vi "TLB Native Dynamic Events ver 0.24.vi"() -> ()   [LabVIEW 2018]
uses:
  Labview Training Phase 2/Enum Controls/States for Action Engine.ctl
  TLB Type Definitions/State Type Definitions, for 0.26g versions and later 2.ctl
  TLB Type Definitions/Intruction Type Definitions.ctl
  TLB Type Definitions/Encoder cluster.ctl
  TLB Type Definitions/PING CLUSTER.ctl
  <vilib>/Studica/Studica Toolkit/NavX/NavX.lvlib
  <vilib>/Studica/Studica Toolkit/Background/DIO Channel.ctl
  Underlying VI's/NavX VI/navX type def.ctl
  <vilib>/Studica/Studica Toolkit/Background/I2C Channel.ctl
  TLB Type Definitions/Vision cluster.ctl
  <vilib>/NI_Real-Time Target Support.lvlib
  TLB Type Definitions/Stepper cluster.ctl
  Experimental VI's/Archived VI's/MOTOR CONTROL NO PID Type Def.ctl
  Underlying VI's/I2C Master VI/I2C MASTER Type Def.ctl
  Underlying VI's/I2C Master VI/I2C_MASTER_WRITE_NEW Type Def.ctl
  <vilib>/userdefined/High Color/IMAQdx.ctl
  Underlying VI's/I2C Master VI/Arduino_Interfacing.ctl
  TLB Type Definitions/Yaw Cluster.ctl
  TLB Type Definitions/Time cluster.ctl
  TLB Type Definitions/Y Stepper cluster.ctl
  Underlying VI's/Modified webcam FGV/Webcam AE.ctl
  Underlying VI's/Elasped Timer/Elapsed timer control.ctl
  Underlying VI's/Motor Control VI with PID/MOTOR CONTROL WITH PID AE DATA MODE TYPE DEF.ctl
  Underlying VI's/Motor Control VI with PID/MOTOR CONTROL WITH PID AE DIRECTION TYPE DEF.ctl
  TLB Type Definitions/IR Sensor Type Def.ctl
  <vilib>/myRIO/Common/Instrument Driver Framework/myRIO v1.0/AI/typedefs/AI Channels Enum.ctl
  <vilib>/myRIO/Common/Instrument Driver Framework/myRIO v1.0/AI/typedefs/AI Channels List.ctl
  TLB Type Definitions/Motor Speed Cluster.ctl
  Underlying VI's/IMAQ Create Reference AE/IMAQ Reference AE.ctl
  TLB Type Definitions/Line Sensor Cluster.ctl
  Underlying VI's/Line Sensor AE/Line Sensor AE Type Def.ctl
  <vilib>/Studica/Studica Toolkit/NavX/TypeDefs/Flags/Z900_navX_Flags_CalibrationStatusTypeDef.ctl
  <vilib>/Studica/Studica Toolkit/NavX/TypeDefs/Flags/Z900_navX_Flags_OpStatusTypeDef.ctl
panel:
  out "Front Wall detected":bool
  out "CPU 1 Usage":dbl
  out "CPU 0 Usage":dbl
  out "Line sensors":T1
  out "IR Sensors":T2
  out "Time up":T3
  out "NAVX Values":T4
  out "Stepper position values":T5
  out "Encoder values":T6
  out "Ultrasonic sensors":T7
  out "Stop?":bool
  out "Selected Task":T8=enum."Start Task 9"
  out "Object recognition mode":enum16{"Ball", "Soap", "Gel", "Pipe", "None"}(ring)
  out "Correcte stepper":u8
  out "Image Processing Error":errorcluster
  out "Object Detection":T9
  out "Status":T12 {"OP Status" items=["INITIALIZING", "SELFTEST_IN_PROGRESS", "ERROR", "IMU_AUTOCAL_IN_PROGRESS", "NORMAL"]; "Calibration Status" items=["IMU_CAL_STATE_MASK"=3, "IMU_CAL_STATE_INPROGRESS"=0, "IMU_CAL_STATE_ACCUMULATE"=1, "IMU_CAL_STATE_COMPLETE"=2]}
  out "General Errors":errorcluster
  in  "Red LED":bool
  out "Table obstruct":bool
  out "x-y":dbl
  out "Obstacle detected":bool
  out "Speed & distance":T13
  out "Task selection":u8
  out "NavX Readings":T14
  out "Arduino Data":T15
  out "TASK ENABLE":bool
  out "Rising Edge":bool
  in  "Green LED":bool
  out "State Logic":T16=enum."Startup"
  out "elements":T8[](array[typedef])
  in  "STOP TASK":bool
  in  "OK Button":bool
  in  "STOP":bool
  out "Queue Errors":errorcluster
  out "Action Queue Items":i32
  out "State Logic Queue Items":i32
  out "Action Queues items":string[](array[string])=["Hardware reset", "Software reset", ""]
  out "Action State":string
  # "VISION"
  # "TLB FRAMEWORK STATUS"
  # "System Health Status Update"
  # "Test Programme written by Calvin Loke    Dated: 28 Aug 2019\nTest Programme revised by Dr Alex See   Dated 30 Aug 2019\n\nRevision date: 20/03/2020\nProgramme version:   TLB Native Dynamic Events ver 0.19a"
  # "0: Task 1\n1: Task 2\n2: Task 3\n3: Task 4\n4: Task 5\n5: Task 6\n6: Task 7\n7: Task 8 Ball\n8: Task 8 Soap\n9: Task 8 Gel\n10: Task 8 Pipe\n11: Task 9 Blue\n12: Task 9 Black\n13: Task 9 Green\n14: Task 9 Red\n15: Task 9 Yellow"
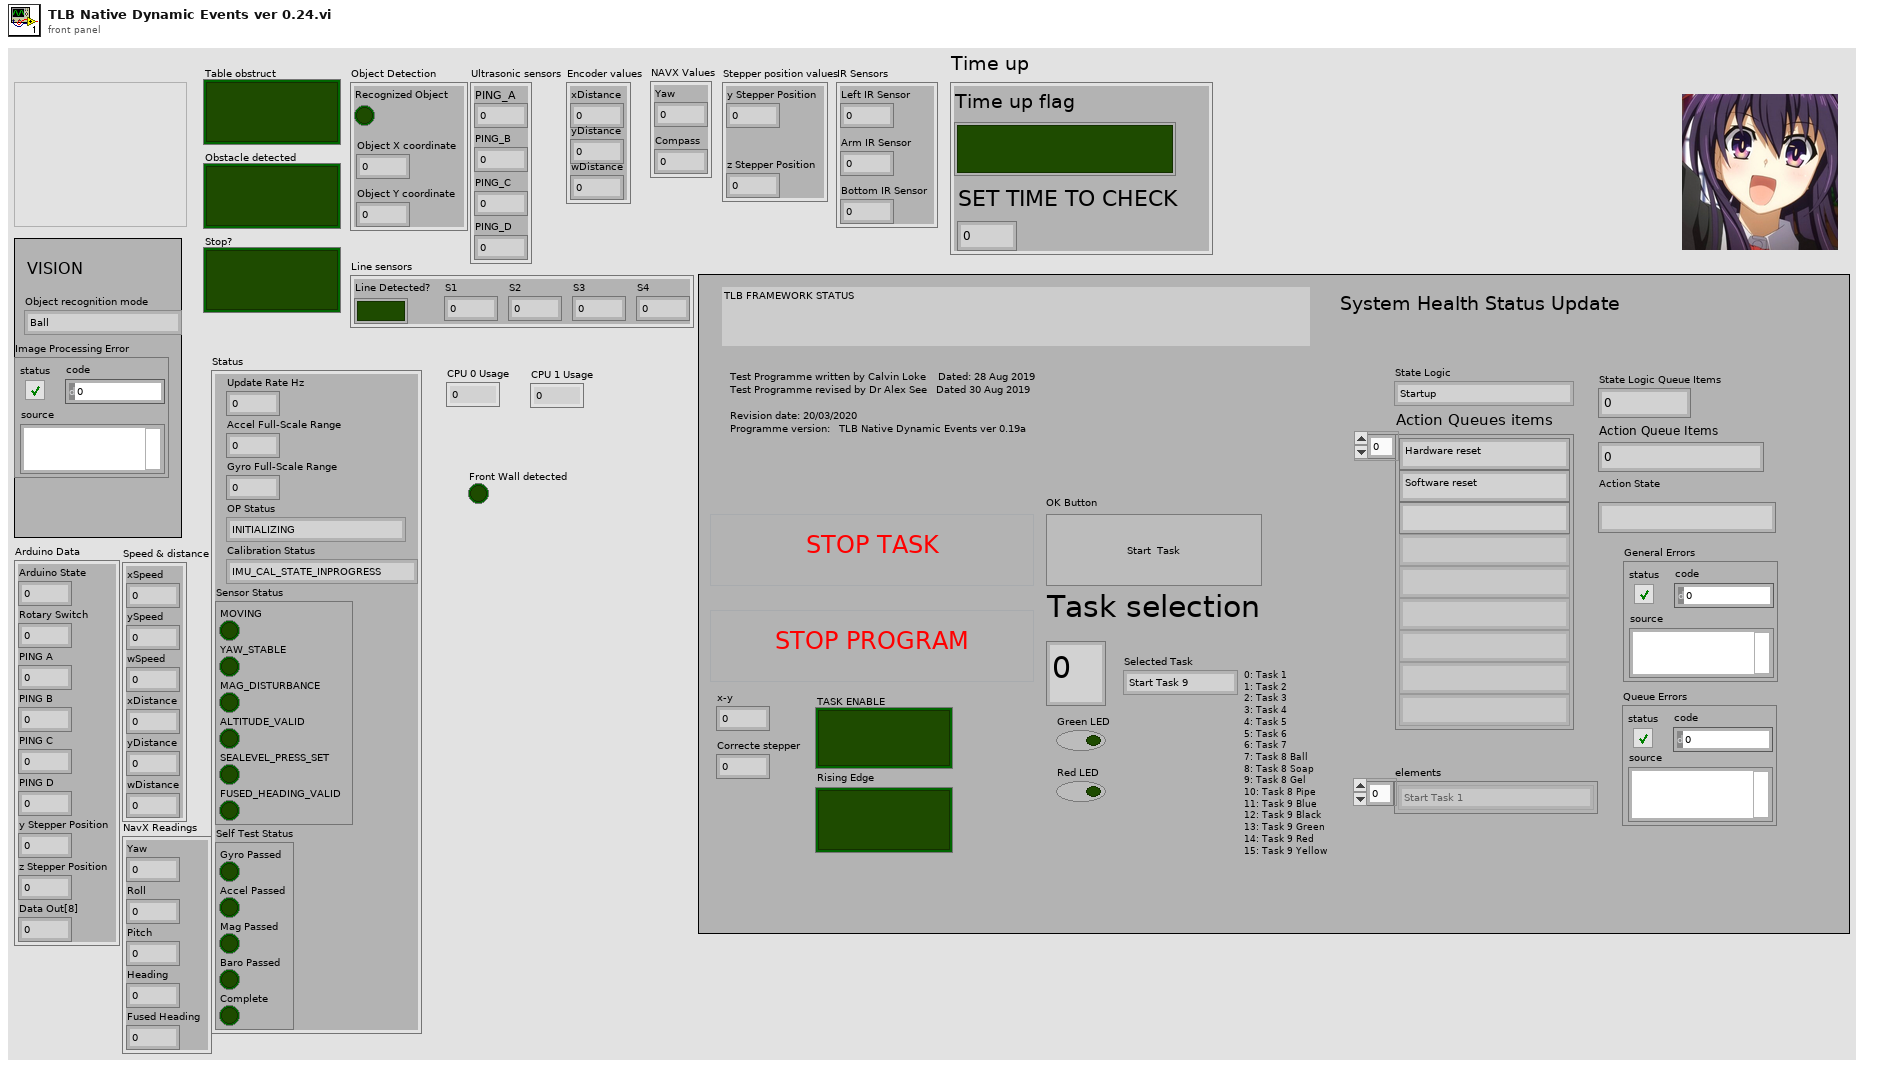
[diagram p1: front panel]
types:
  T1 = typedef "Line Sensor Cluster.ctl" = cluster{"Line Detected?":bool, "S1":dbl, "S2":dbl, "S3":dbl, "S4":dbl}
  T2 = typedef "IR Sensor Type Def.ctl" = cluster{"Left IR Sensor":dbl, "Arm IR Sensor":dbl, "Bottom IR Sensor":dbl}
  T3 = typedef "Time cluster.ctl" = cluster{"Time up flag":bool, "SET TIME TO CHECK":dbl}
  T4 = typedef "Yaw Cluster.ctl" = cluster{"Yaw":dbl, "Compass":dbl}
  T5 = typedef "Stepper cluster.ctl" = cluster{"y Stepper Position":u8, "z Stepper Position":u8}
  T6 = typedef "Encoder cluster.ctl" = cluster{"xDistance":dbl, "yDistance":dbl, "wDistance":dbl}
  T7 = typedef "PING CLUSTER.ctl" = cluster{"PING_A":u8, "PING_B":u8, "PING_C":u8, "PING_D":u8}
  T8 = typedef "Intruction Type Definitions.ctl" = enum16{"None", "Start Task 1", "Start Task 2", "Start Task 3", "Start Task 4", "Start Task 5", "Start Task 6", "Start Task 7", "Start Task 8 - BALL", "Start Task 8 - Gel", "Start Task 8 - Pipe", "Start Task 8 - Soap", "Start Task 9", "Start Task A", "Start Task B", "Exit"}
  T9 = typedef "Vision cluster.ctl" = cluster{"Recognized Object":bool, "Object X coordinate":dbl, "Object Y coordinate":dbl}
  T10 = typedef "NavX.lvlib/Z900_navX_Flags_OpStatusTypeDef.ctl" = u8
  T11 = typedef "NavX.lvlib/Z900_navX_Flags_CalibrationStatusTypeDef.ctl" = u8
  T12 = cluster{"Update Rate Hz":u8, "Accel Full-Scale Range":u8, "Gyro Full-Scale Range":u16, "OP Status":T10, "Calibration Status":T11, "Sensor Status":cluster{"MOVING":bool, "YAW_STABLE":bool, "MAG_DISTURBANCE":bool, "ALTITUDE_VALID":bool, "SEALEVEL_PRESS_SET":bool, "FUSED_HEADING_VALID":bool}, "Self Test Status":cluster{"Gyro Passed":bool, "Accel Passed":bool, "Mag Passed":bool, "Baro Passed":bool, "Complete":bool}}
  T13 = cluster{"xSpeed":dbl, "ySpeed":dbl, "wSpeed":dbl, "xDistance":dbl, "yDistance":dbl, "wDistance":dbl}
  T14 = cluster{"Yaw":dbl, "Roll":dbl, "Pitch":dbl, "Heading":dbl, "Fused Heading":dbl}
  T15 = cluster{"Arduino State":u8, "Rotary Switch":u8, "PING A":u8, "PING B":u8, "PING C":u8, "PING D":u8, "y Stepper Position":u8, "z Stepper Position":u8, "Data Out[8]":u8}
  T16 = typedef "State Type Definitions, for 0.26g versions and later 2.ctl" = enum16{"None", "Startup", "Move to Angle", "True Stop", "Idle", "Shutdown", "Task 1A", "Task 1B", "Task 2:Raise Arm", "Task 2:Sensor Mode", "Task 2:Reverse Mode", "Task 3", "Task 4_A", "Task 4_B", "Task 4_C", "Task 4_D", "Task 5A", "Task 5B", "Task 5C", "Task 5D", "Task 5E: POSITION ARM", "Task 5F: ARM GRAB HEIGHT", "Task 5G: CLOSE CLAW", "Task 5H: RAISE ARM", "Task 6_A", "Task 6_B", "Task 7", "Task 8A: RAISE ARM", "Task 8B: MOVE TO BOX", "Task 8C: CAM BURST", "Task 8D: PROCESS IMAGE", "Task 8E: ROBOT ADJUST", "Task 8F: CAM BURST 2", "Task 8G: PROCESS IMAGE 2", "Task 8H: ARM ADJUST", "Task 8I: ARM GRAB HEIGHT", "Task 8J: CLOSE CLAW", "Task 8K: RAISE MY SWORD", "Task 9A: Raise Arm", "Task 9B: Rotate to Angle", "Task 9C: Detect Box", "Task 9D: MOVE FORWARD", "Task 9E: MOVE LEFT", "Task 9F: SCAN BOX", "Task 9G: MOVE RIGHT", "Task 9H: SCAN BOX 2", "Task 9I: ROTATE 90 CW", "Task 9J: FORWARD", "Task 9K: RAM WALL", "Task 9L: MOVE RIGHT", "Task 9M: SCAN BOX 3", "Task 9M: MOVE RIGHT", "Task 9N: SCAN BOX 4", "PENIS", "PENIS 2", "PENIS 3", "Task 9R: PROCESS COLOUR", "Task A1: Task 9 Open cam", "Task A2: Task 9 Move Arm", "Task A3: Task 9 Set Timer", "Task A4: Tasl 9 Capture images", "Task A5: Task 9 Close camera", "Task A6: Process Colour", "Task A7: Dispose Camera Buffer"}
  T17 = typedef "Motor Speed Cluster.ctl" = cluster{"ySpeed":dbl, "xSpeed":dbl, "wSpeed":dbl}
  T18 = typedef "Y Stepper cluster.ctl" = cluster{"yStepper desired":u8}
  T19 = typedef "DIO Channel.ctl" = enum16{"Not Connected", "A/DIO1", "A/DIO2", "A/DIO3", "A/DIO4", "A/DIO5", "A/DIO6", "A/DIO7", "A/DIO13", "B/DIO1", "B/DIO2", "B/DIO3", "B/DIO4", "B/DIO5", "B/DIO6", "B/DIO7", "B/DIO13", "C/DIO0", "C/DIO1", "C/DIO2", "C/DIO3", "C/DIO4", "C/DIO5", "C/DIO6", "C/DIO7"}
  T20 = cluster{"DIO Channel":T19, "FPGA VI Reference Out":refnum<k20>}
  T21 = typedef "States for Action Engine.ctl" = enum16{"Initialize", "Write", "Read"}
  T22 = typedef "NI_Real-Time Target Support.lvlib/RT CPU Load.ctl" = cluster{"Total (%)":dbl, "Time Critical (%)":dbl, "Timed Structures (%)":dbl, "High (%)":dbl, "Above Normal (%)":dbl, "Normal (%)":dbl, "Background (%)":dbl, "Idle (%)":dbl, "ISR (%)":dbl}
  T23 = cluster{"CPU loads[0]":T22, "CPU loads[1]":T22, "CPU loads[2]":T22, "CPU loads[3]":T22, "CPU loads[4]":T22, "CPU loads[5]":T22, "CPU loads[6]":T22, "CPU loads[7]":T22, "CPU loads[8]":T22}
  T24 = typedef "navX type def.ctl" = enum16{"Get i2C reference", "Read Values", "Zero Yaw"}
  T25 = typedef "Arduino_Interfacing.ctl" = enum16{"Initialize", "Write to Arduino", "Read From Arduino"}
  T26 = typedef "I2C Channel.ctl" = enum16{"Not Connected", "A", "B"}
  T27 = cluster{"I2C Ref Out":cluster{"I2C Channel":T26, "FPGA VI Reference Out":refnum<k20>}, "Connected":bool, "Slave Address (7-bit)":u8, "Registry":u8[]}
  T28 = typedef "State Type Definitions.ctl" = enum16{"None", "Startup", "Move to Angle", "True Stop", "Idle", "Shutdown", "Task 1A", "Task 1B", "Task 2:Raise Arm", "Task 2:Sensor Mode", "Task 2:Reverse Mode", "Task 3", "Task 4_A", "Task 4_B", "Task 4_C", "Task 4_D", "Task 5A", "Task 5B", "Task 5C", "Task 5D", "Task 5E: POSITION ARM", "Task 5F: ARM GRAB HEIGHT", "Task 5G: CLOSE CLAW", "Task 5H: RAISE ARM", "Task 6_A", "Task 6_B", "Task 7", "Task 8A: RAISE ARM", "Task 8B: MOVE TO BOX", "Task 8C: CAM BURST", "Task 8D: PROCESS IMAGE", "Task 8E: ROBOT ADJUST", "Task 8F: CAM BURST 2", "Task 8G: PROCESS IMAGE 2", "Task 8H: ARM ADJUST", "Task 8I: ARM GRAB HEIGHT", "Task 8J: CLOSE CLAW", "Task 8K: RAISE MY SWORD", "Task 9A: Raise Arm", "Task 9B: Rotate to Angle", "Task 9C: Detect Box", "Task 9D: MOVE FORWARD", "Task 9E: MOVE LEFT", "Task 9F: SCAN IMAGE", "Task 9G: PROCESS COLOUR", "Task 9H: MOVE RIGHT", "Task 9I: SCAN IMAGE", "Task 9J: PROCESS COLOUR", "Task 9K: ROTATE 90 CW", "Task 9L: MOVE FORWARD", "Task 9M: MOVE RIGHT", "Task 9N: SCAN IMAGE", "Task 9O: PROCESS COLOUR", "Task 9P: MOVE RIGHT", "Task 9Q: SCAN IMAGE", "Task 9R: PROCESS COLOUR", "Task A1: Raise Arm", "Task A2: Rotate to Angle", "Task A3: Move Forward", "Task A4: Rotate CW 90"}
  T29 = typedef "MOTOR CONTROL WITH PID AE DIRECTION TYPE DEF.ctl" = enum16{"y-axis movement", "x-axis movement", "rotation", "stop", "reset encoders"}
  T30 = typedef "MOTOR CONTROL WITH PID AE DATA MODE TYPE DEF.ctl" = enum16{"Init AE", "Write to AE", "Read from AE"}
  T31 = typedef "Line Sensor AE Type Def.ctl" = enum16{"INIT AE", "READ FROM LINE SENSORS"}
  T32 = typedef "IMAQ Reference AE.ctl" = enum16{"Initialize AE", "Get IMAQ Reference", "Dispose Processing Buffer"}
  T33 = typedef "Elapsed timer control.ctl" = enum16{"Start", "Pause", "Initialize"}
  T34 = typedef "I2C_MASTER_WRITE_NEW Type Def.ctl" = enum16{"Ultrasonic sensors", "Stepper origin", "zStepper 13.3k", "zStepper 13k", "zStepper 12k", "zStepper 11k", "zStepper 10k", "zStepper 9k", "zStepper 8k", "zStepper 7k", "zStepper 6k", "zStepper 5k", "zStepper 4k", "zStepper 3k", "zStepper 2k", "zStepper 1k", "zStepper 900", "zStepper 800", "zStepper 700", "zStepper 600", "zStepper 500", "zStepper 400", "zStepper 300", "zStepper 200", "zStepper 100", "zStepper 0", "yStepper control", "Open Claw", "Close Claw", "Soft Reset"}
  T35 = typedef "Webcam AE.ctl" = enum16{"Initialize Camera", "Open Camera", "Continuous Acquisition", "Close Camera", "Retrieve Image", "Dispose Camera Image Buffer"}
  T36 = typedef "IMAQdx.ctl" = refnum<k21>
  T37 = typedef "MOTOR CONTROL NO PID Type Def.ctl" = enum16{"Init", "Front Back", "Left Right", "Rotate", "Stop", "Latch"}
  T38 = typedef "AI Channels List.ctl" = T39[]
  T39 = typedef "AI Channels Enum.ctl" = enum16{"Not Connected", "AudioIn/Left", "AudioIn/Right", "C/AI0", "C/AI1", "A/AI0", "A/AI1", "A/AI2", "A/AI3", "A/AI4", "A/AI5", "A/AI6", "A/AI7", "B/AI0", "B/AI1", "B/AI2", "B/AI3", "B/AI4", "B/AI5", "B/AI6", "B/AI7", "AI/AI0", "AI/AI1", "AI/AI2", "AI/AI3", "A/AI0 (DIFF)", "A/AI1 (DIFF)", "A/AI2 (DIFF)", "A/AI3 (DIFF)", "B/AI0 (DIFF)", "B/AI1 (DIFF)", "B/AI2 (DIFF)", "B/AI3 (DIFF)"}
  T40 = cluster{"S1":dbl, "S2":dbl, "S3":dbl, "S4":dbl, "Array[4]":dbl, "Array[5]":dbl, "Array[6]":dbl, "Array[7]":dbl, "Array[8]":dbl}
  T41 = typedef "I2C MASTER Type Def.ctl" = enum16{"Last State", "Mode 0", "Mode 1", "Mode 2", "Mode 3", "Mode 4", "Mode 5", "Mode 6", "Mode 7", "Mode 8", "Mode 9", "Mode 10"}
  T42 = typedef "IMAQ Image.ctl" = refnum<image>
  T43 = cluster{"Number of Matches":i32, "Object detected?":bool}
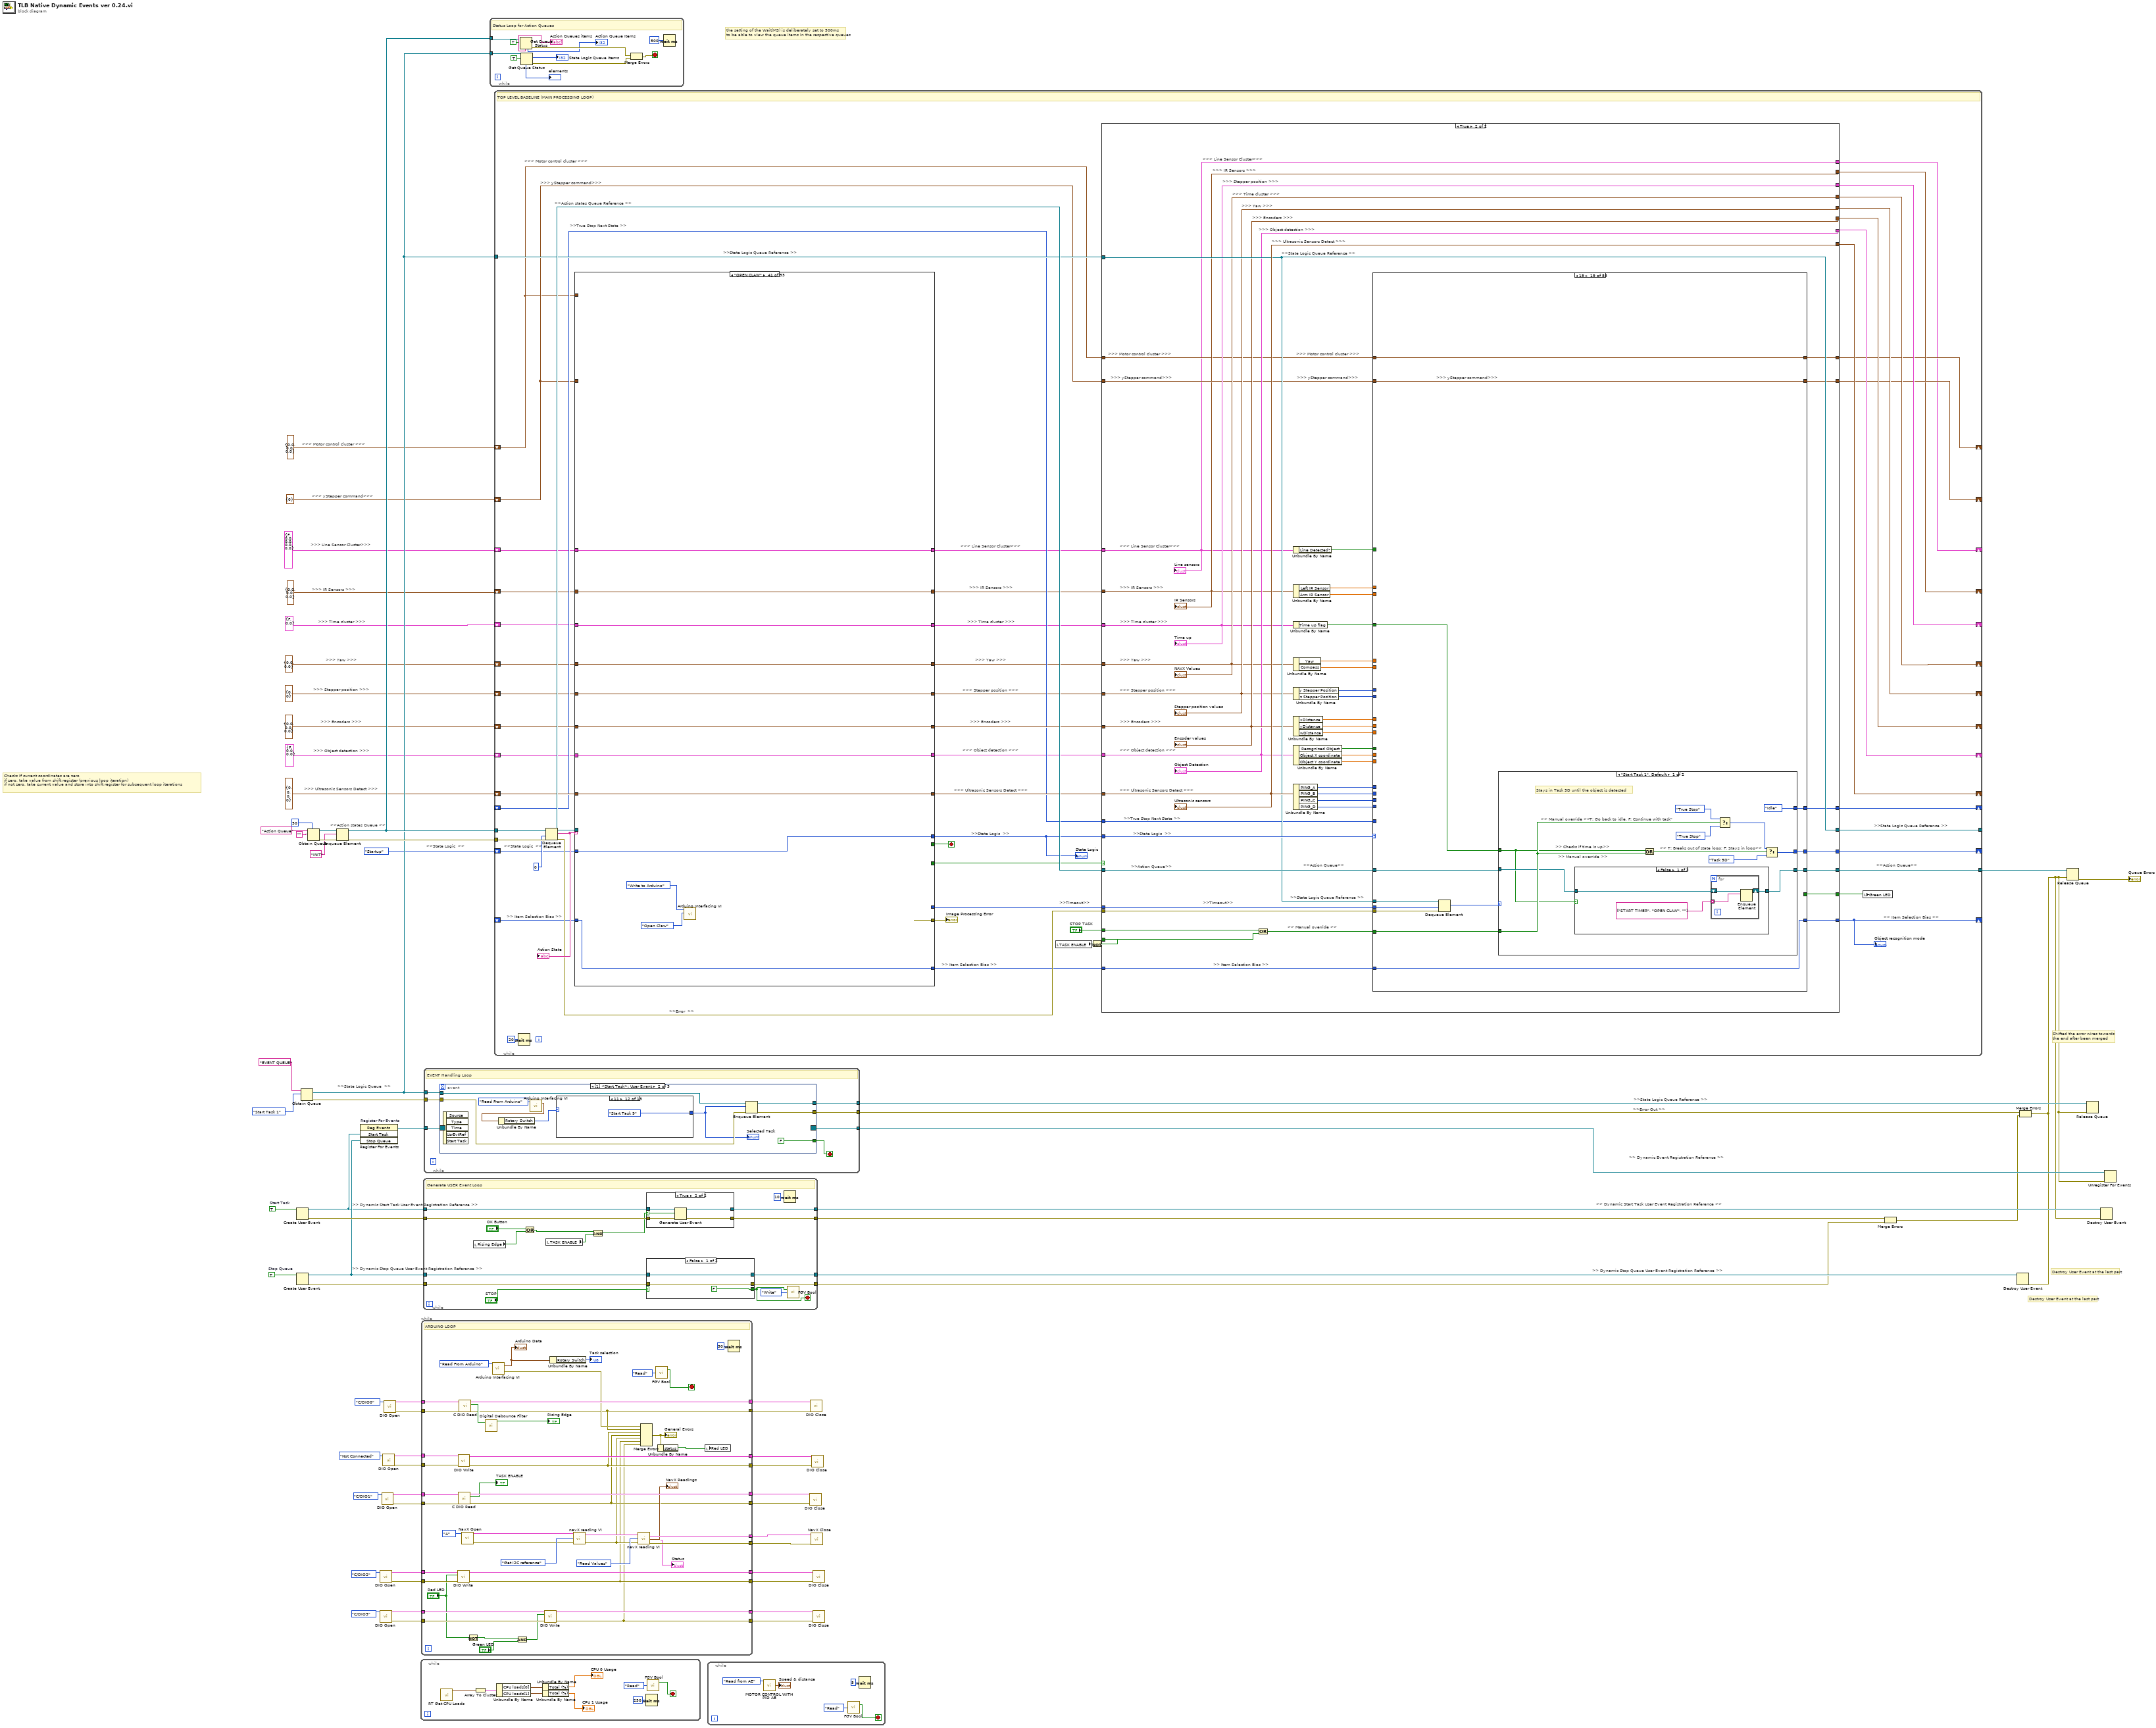
[diagram p0: block diagram]
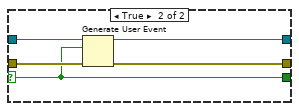
[diagram p2: hidden frame]
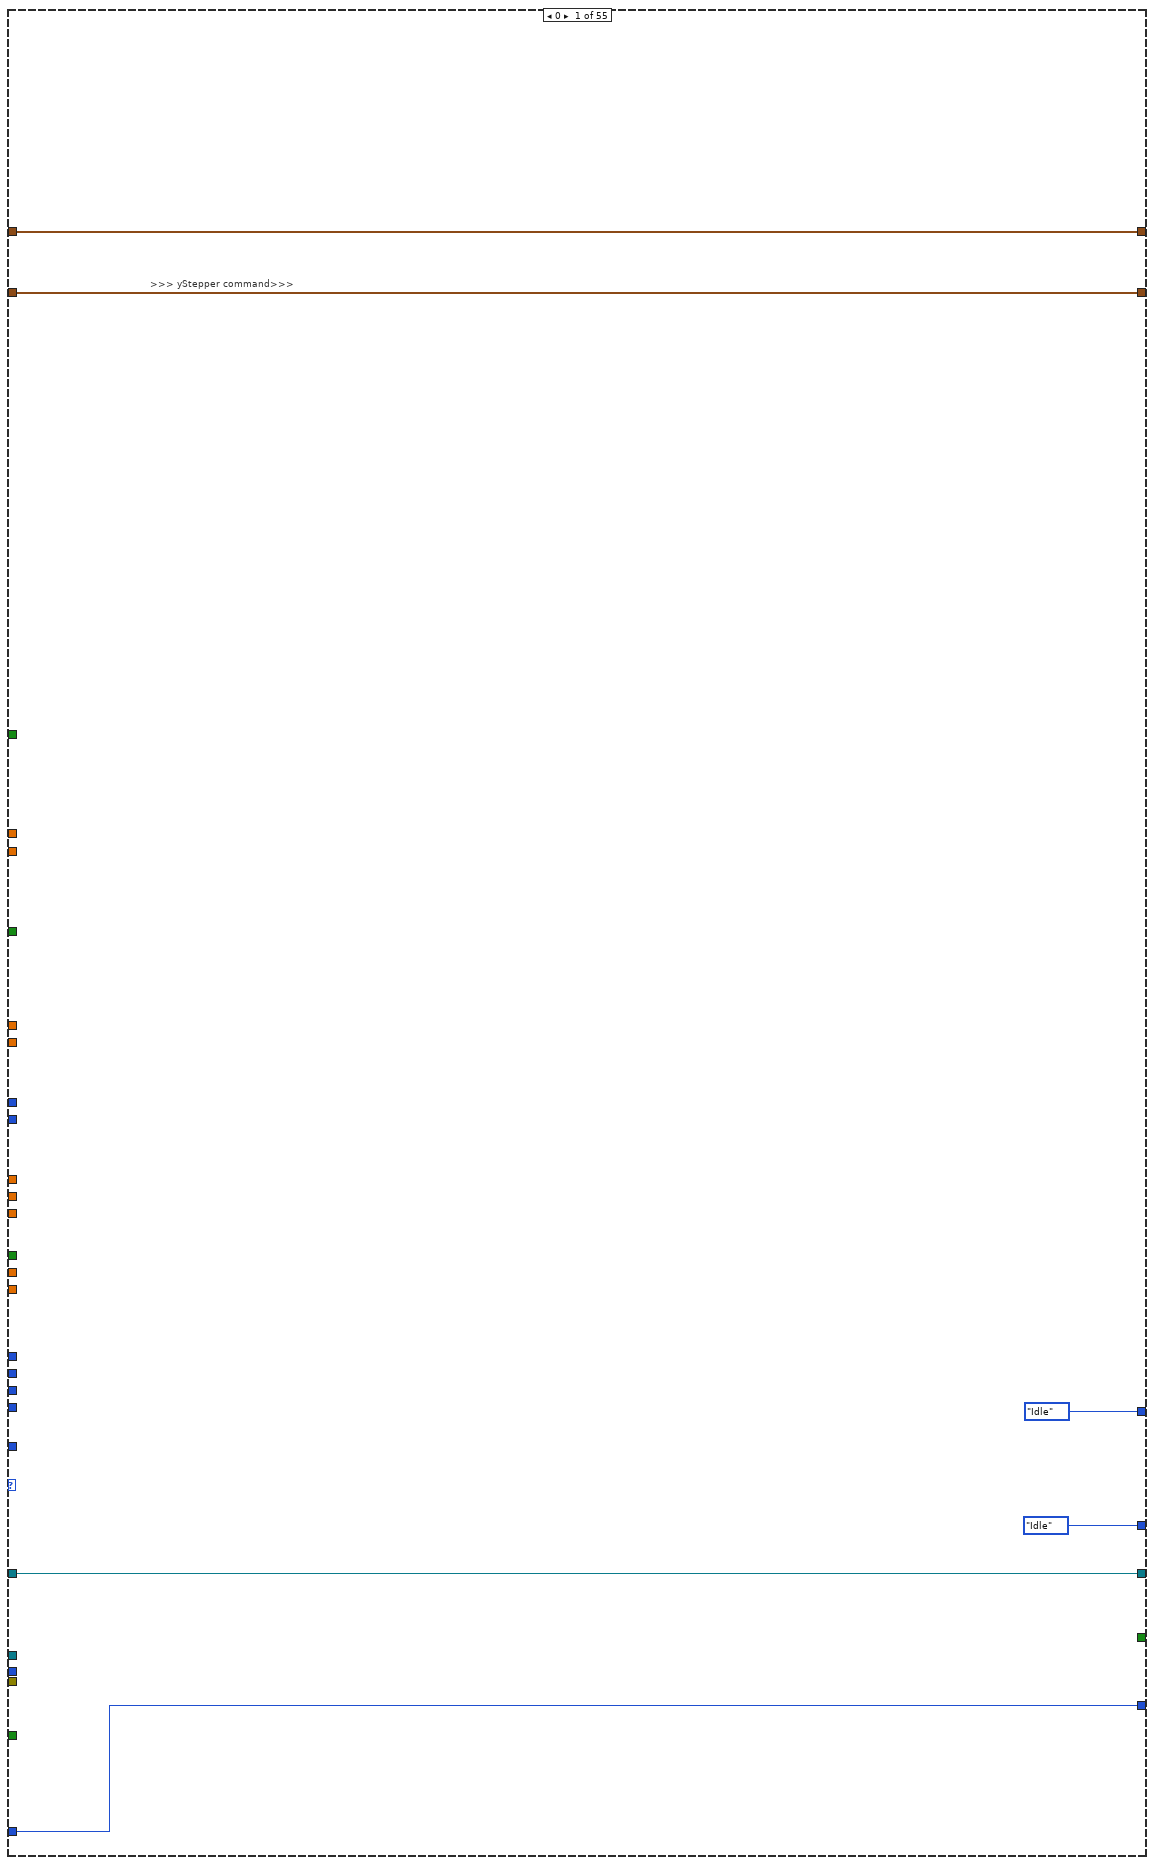
[diagram p5: hidden frame]
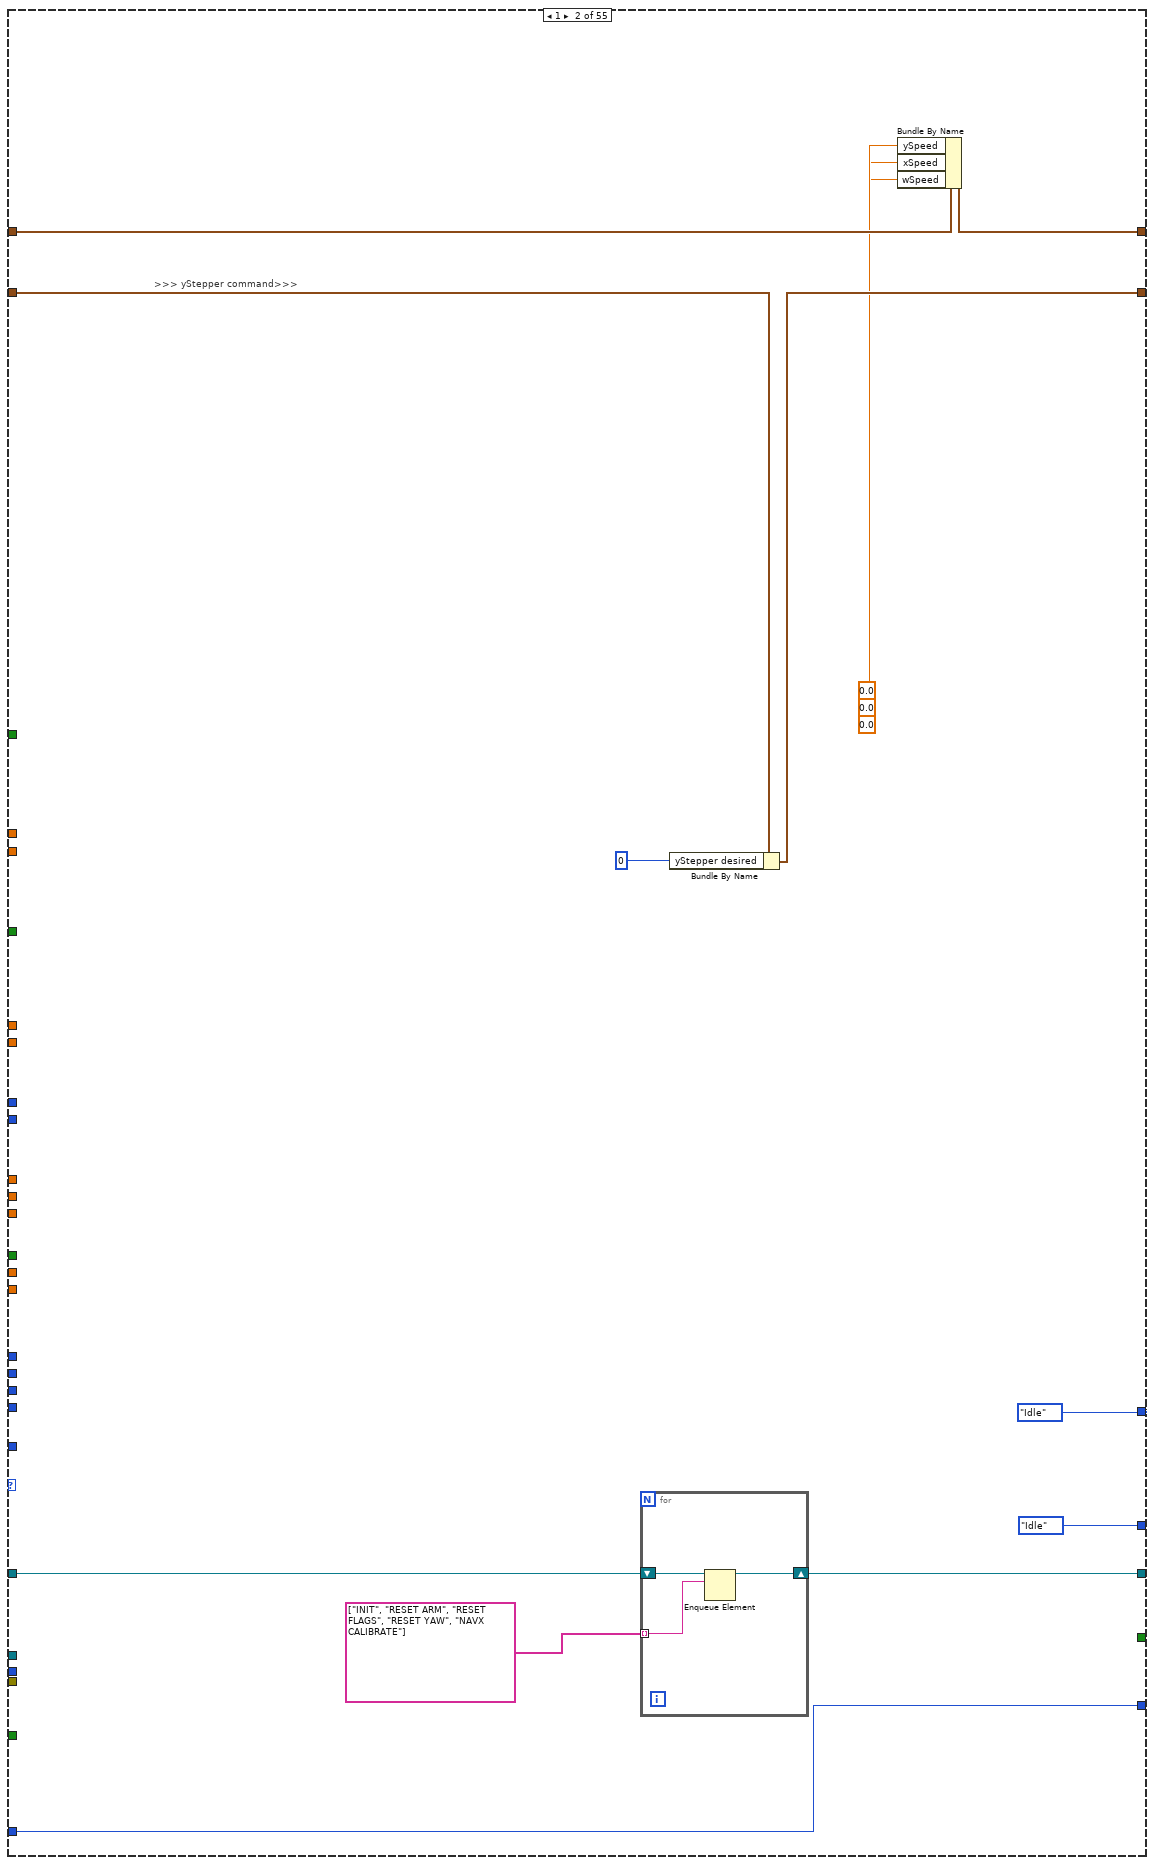
[diagram p6: hidden frame]
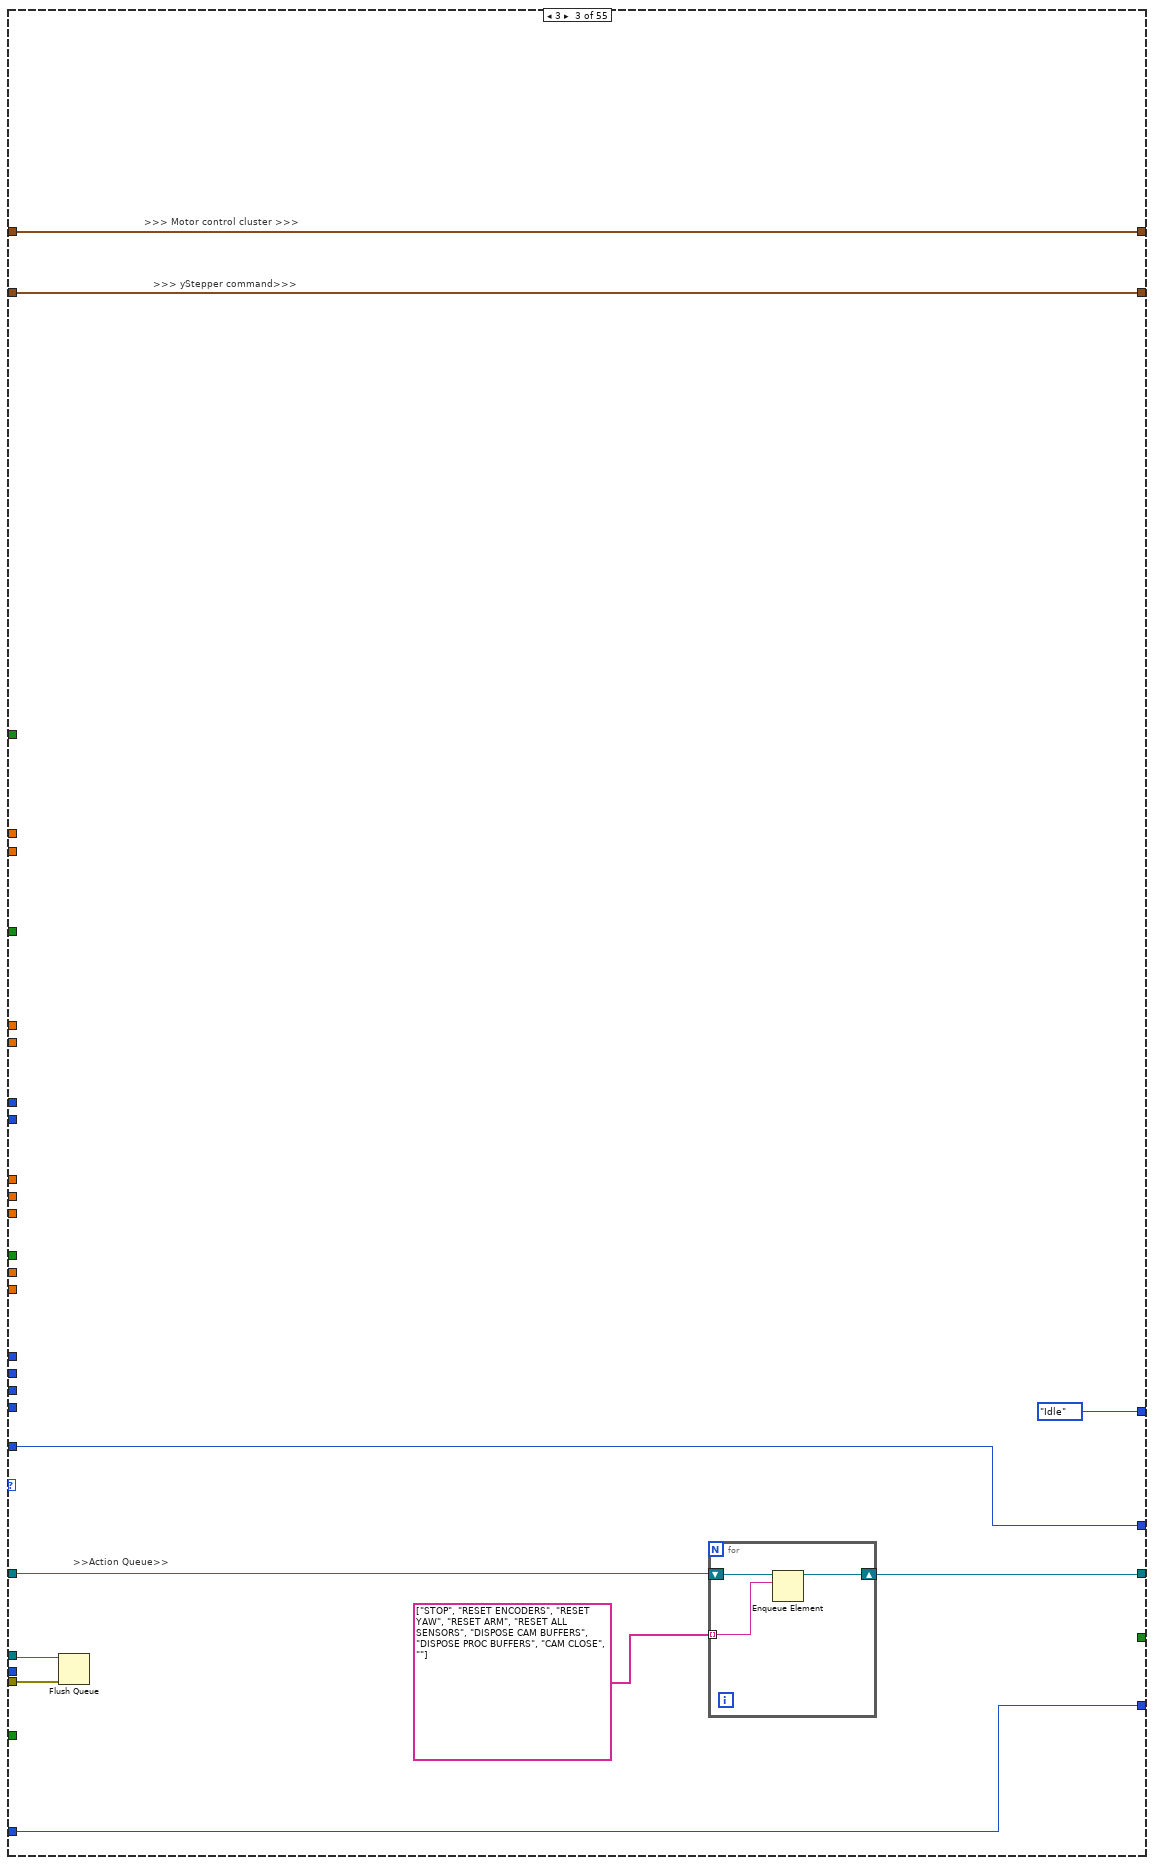
[diagram p7: hidden frame]
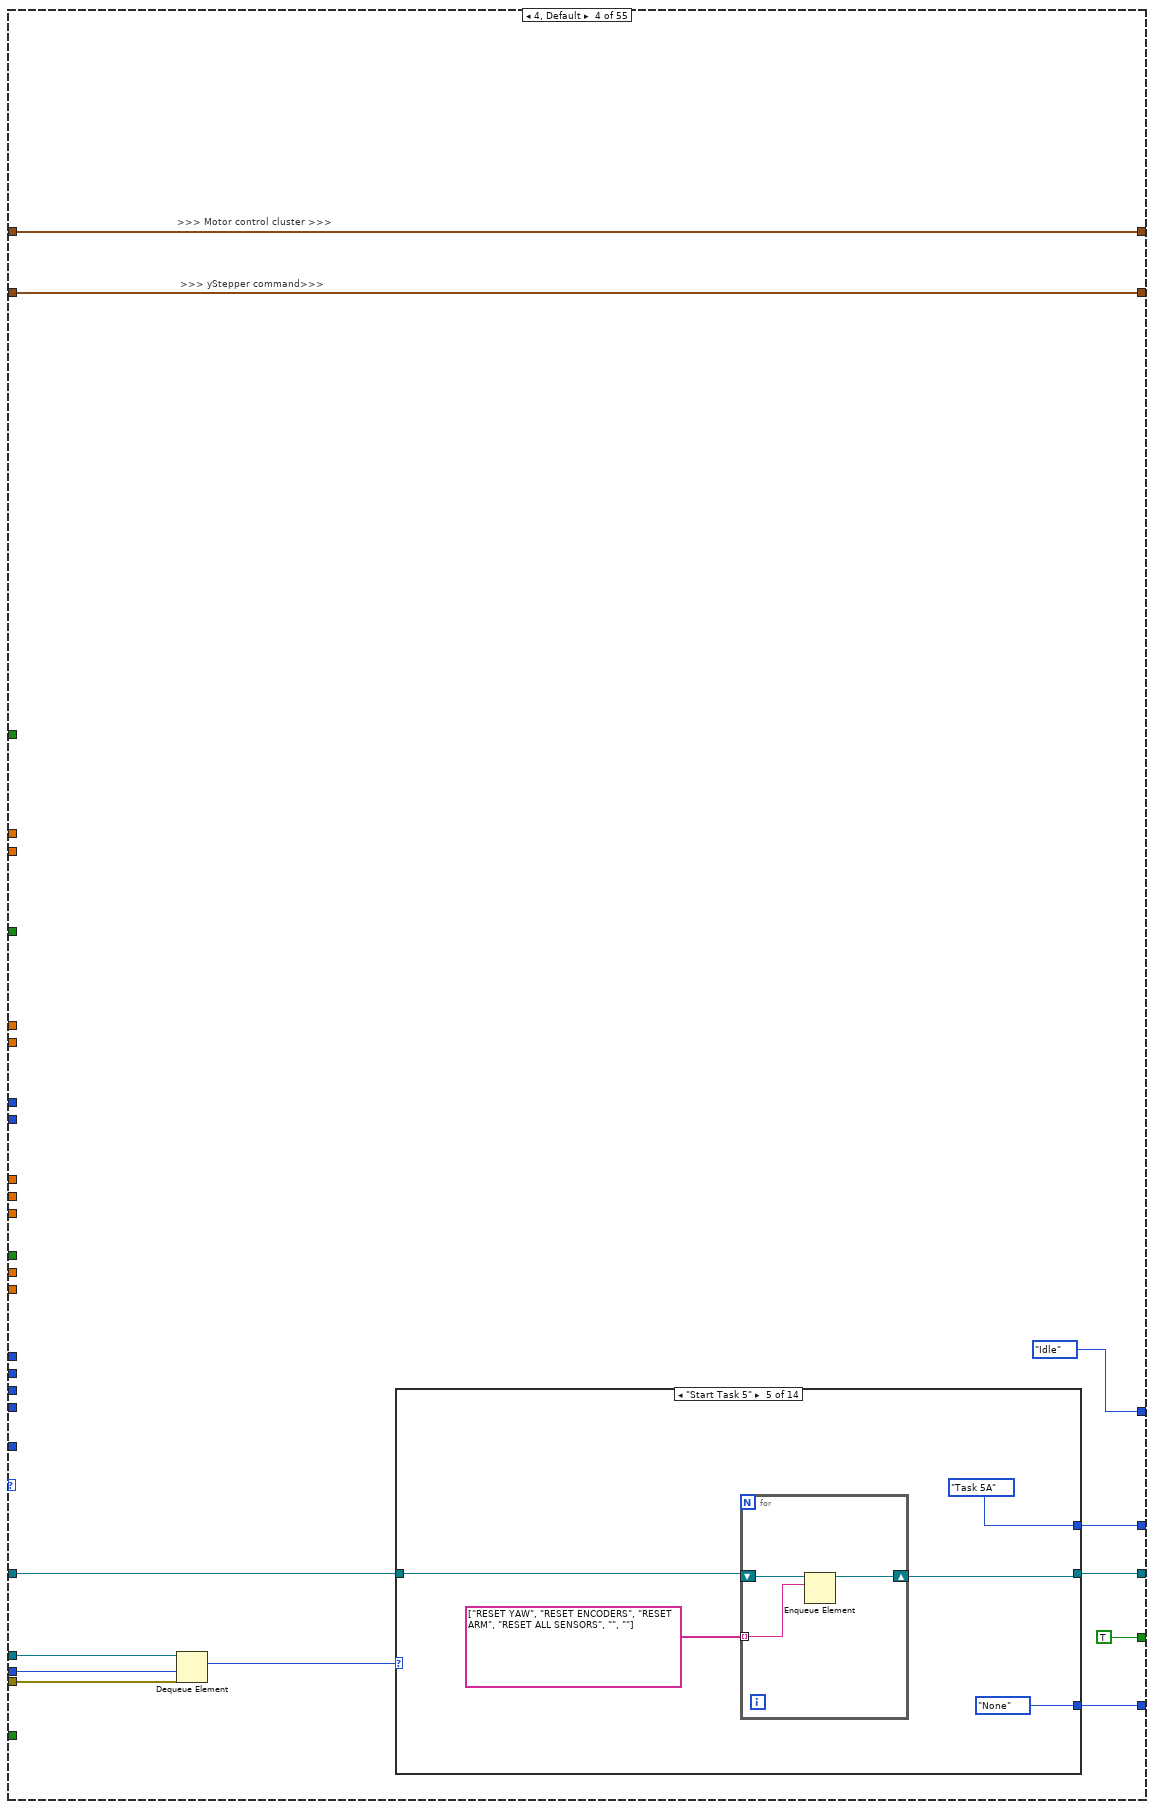
[diagram p8: hidden frame]
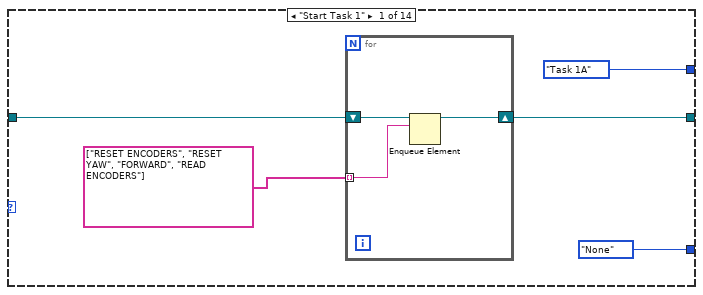
[diagram p9: hidden frame]
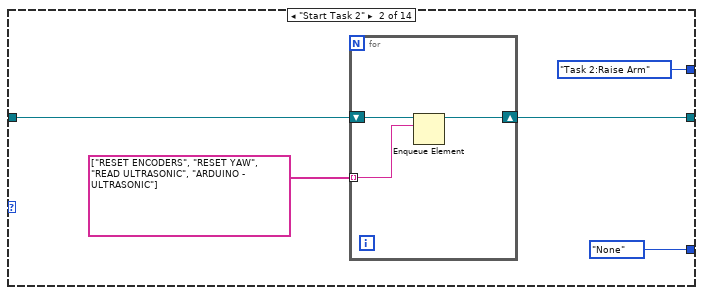
[diagram p10: hidden frame]
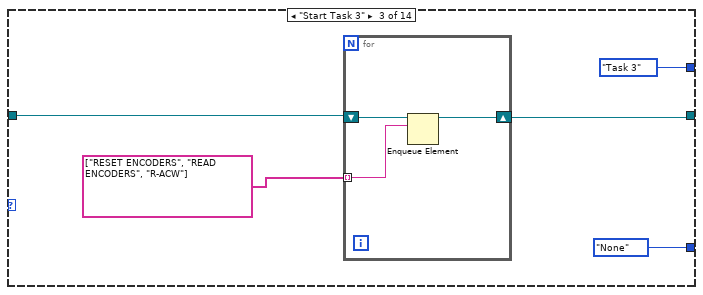
[diagram p11: hidden frame]
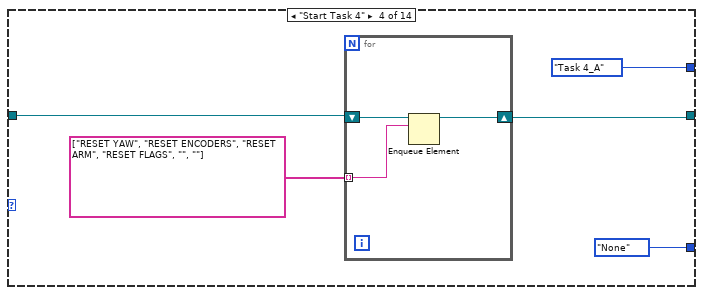
[diagram p12: hidden frame]
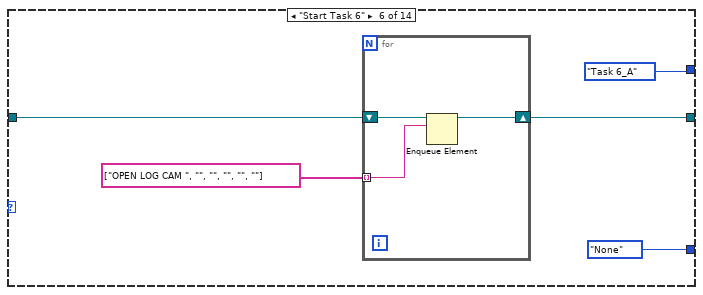
[diagram p13: hidden frame]
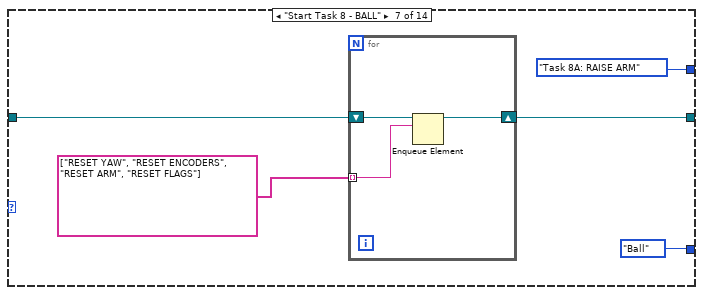
[diagram p14: hidden frame]
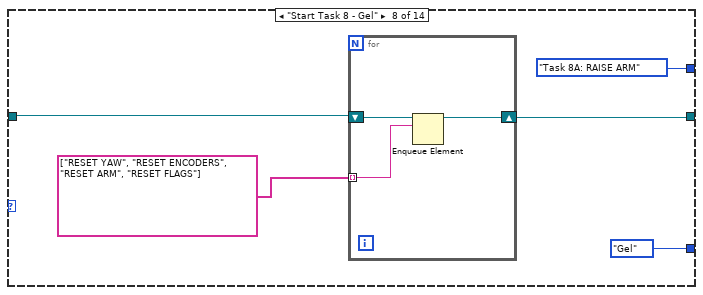
[diagram p15: hidden frame]
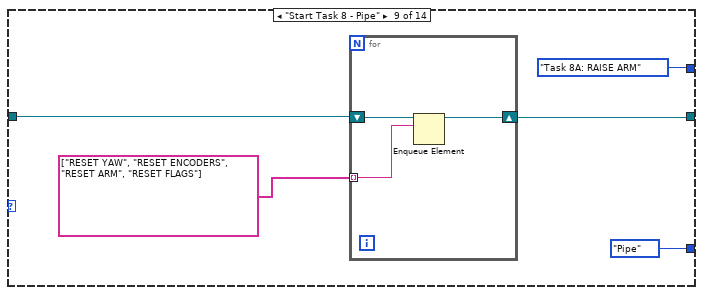
[diagram p16: hidden frame]
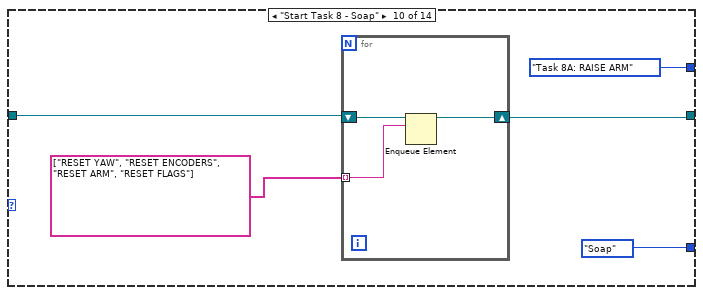
[diagram p17: hidden frame]
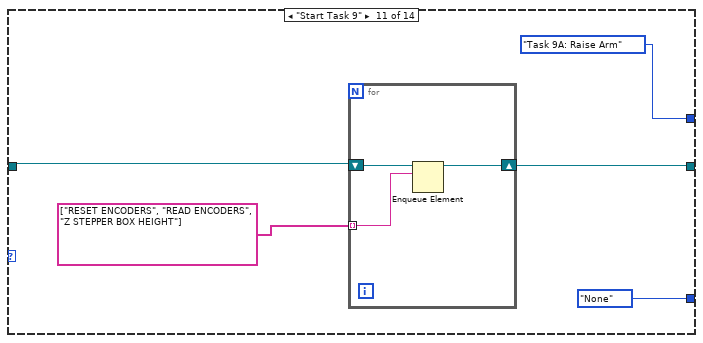
[diagram p18: hidden frame]
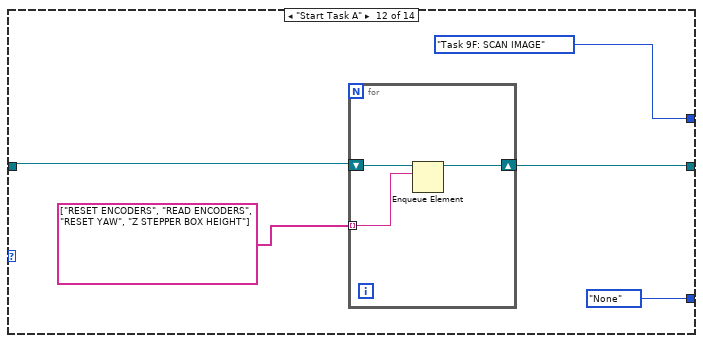
[diagram p19: hidden frame]
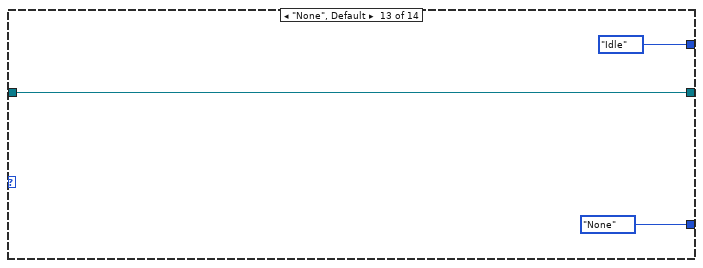
[diagram p20: hidden frame]
diagram:
  w68 = TRUE  # Stop Queue
  w67 = TRUE  # Start Task
  # ">>State Logic  >>"
  # ">>> Line Sensor Cluster>>>"
  # ">>> Motor control cluster >>>"
  # ">>> IR Sensors >>>"
  # "Checks if current coordinates are zero\nif zero, take value from shift register (previous loop iteration)\nif not zero, take current value and store into shift register for subsequent loop iterations"
  # ">>> yStepper command>>>"
  # ">>> Time cluster >>>"
  # ">>> Yaw >>>"
  # ">>> Stepper position >>>"
  # ">>> Encoders >>>"
  # ">>> Object detection >>>"
  # ">>> Ultrasonic Sensors Detect >>>"
  # "the setting of the Wait(MS) is deliberately set to 500ms\nto be able to view the queue items in the respective queues"
  # ">>Error Out >>"
  # ">> Dynamic Stop Queue User Event Registration Reference >>"
  # ">> Dynamic Start Task User Event Registration Reference >>"
  # ">> Dynamic Stop Queue User Event Registration Reference >>"
  # ">> Dynamic Start Task User Event Registration Reference >>"
  # ">> Dynamic Event Registration Reference >>"
  # ">>Action states Queue >>"
  # ">>State Logic Queue  >>"
  # ">>State Logic Queue Reference >>"
  # "Destroy User Event at the last part"
  # "Destroy User Event at the last part"
  # "Shifted the error wires towards\nthe end after been merged"
  n1 = Create User Event(user event datatype=w67) -> (user event=w59:refnum<user-event>, error out=w64:errorcluster)  [unwired: 1 in]
  n2 = Create User Event(user event datatype=w68) -> (user event=w60:refnum<user-event>, error out=w63:errorcluster)  [unwired: 1 in]
  n3 = Obtain Queue(name (unnamed)="EVENT QUEUE", element data type=Intruction_Type_Definitions."Start Task 1" ("Enum")) -> (queue out=w45:refnum<queue>, error out=w51:errorcluster)  [unwired: 3 in, 1 out]
  n4 = Obtain Queue(max queue size (-1, unlimited)=50, name (unnamed)="Action Queue", element data type="") -> (queue out=w54:refnum<queue>, error out=w50:errorcluster)  [unwired: 2 in, 1 out]
  n5 = Enqueue Element(queue=w54, element="INIT", error in (no error)=w50) -> (queue out=w46:refnum<queue>, error out=w49:errorcluster)  [unwired: 1 in, 1 out]
  n6 = register-events "Register For Events"(w59, w60) -> (reference out=w58:refnum<event-registration>)  [unwired: 2 in, 1 out]
  n7 = call <vilib>:"DIO Open.vi"("DIO Channel"=DIO_Channel."C/DIO2") -> ("error out"=w18:errorcluster, "DIO Info Out"=w19:T20)  [unwired: 9 in]
  n8 = call <vilib>:"DIO Open.vi"("DIO Channel"=DIO_Channel."C/DIO3") -> ("error out"=w13:errorcluster, "DIO Info Out"=w14:T20)  [unwired: 9 in]
  n9 = call <vilib>:"DIO Open.vi"("DIO Channel"=DIO_Channel."C/DIO1") -> ("error out"=w23:errorcluster, "DIO Info Out"=w24:T20)  [unwired: 9 in]
  n10 = call <vilib>:"DIO Open.vi"("DIO Channel"=DIO_Channel."Not Connected") -> ("error out"=w28:errorcluster, "DIO Info Out"=w30:T20)  [unwired: 9 in]
  n11 = call <vilib>:"DIO Open.vi"("DIO Channel"=DIO_Channel."C/DIO0") -> ("error out"=w33:errorcluster, "DIO Info Out"=w36:T20)  [unwired: 9 in]
  n12 = while {
    stop <- w75 stop-if-true
    n13 = call <vilib>:"RT Get CPU Loads.vi"() -> ("CPU loads"=w74:T22[])  [unwired: 10 in, 1 out]
    n14 = Array To Cluster(array=w74) -> (cluster=w73:T23)
    n15 = Unbundle By Name(w73) -> ("CPU loads[0]"=w72:T22, "CPU loads[1]"=w71:T22)
    n16 = Unbundle By Name(w72) -> ("Total (%)"=→"CPU 0 Usage":dbl)
    n17 = Unbundle By Name(w71) -> ("Total (%)"=→"CPU 1 Usage":dbl)
    n18 = Wait (ms)(milliseconds to wait=u32 250) -> ()  [unwired: 1 out]
    n19 = call "FGV Bool.vi"("Init/Read/Write State"=States_for_Action_Engine."Read") -> ("Output node"=w75:bool)  [unwired: 2 in, 1 out]
  }
  n20 = while {
    tunnel: w36 -> [w121]
    tunnel: [w120] -> w34
    tunnel: w33 -> [w119]
    tunnel: [w90] -> w32
    tunnel: w30 -> [w116]
    tunnel: [w115] -> w29
    tunnel: w28 -> [w114]
    tunnel: [w89] -> w27
    tunnel: [w113] -> w25
    tunnel: w24 -> [w112]
    tunnel: w23 -> [w111]
    tunnel: [w88] -> w22
    tunnel: w19 -> [w105]
    tunnel: w18 -> [w104]
    tunnel: [w103] -> w17
    tunnel: [w86] -> w16
    tunnel: w14 -> [w102]
    tunnel: w13 -> [w101]
    tunnel: [w100] -> w12
    tunnel: [w85] -> w11
    tunnel: [w97] -> w8
    tunnel: [w96] -> w9
    stop <- w123 stop-if-true
    # "ARDUINO LOOP"
    n21 = call <vilib>:"DIO Write.vi"("error in (no error)"=w104, "Input"="Red LED", "DIO Info In"=w105) -> ("error out"=w86:errorcluster, "DIO Info Out"=w103:T20)  [unwired: 7 in]
    n22 = call <vilib>:"DIO Write.vi"("error in (no error)"=w114, "DIO Info In"=w116) -> ("error out"=w89:errorcluster, "DIO Info Out"=w115:T20)  [unwired: 8 in]
    n23 = call <vilib>:"C DIO Read.vi"("error in (no error)"=w111, "DIO Info In in"=w112) -> ("error out"=w88:errorcluster, "IN"=→"TASK ENABLE":bool, "DIO Info In out"=w113:T20)  [unwired: 7 in]
    n24 = call <vilib>:"C DIO Read.vi"("error in (no error)"=w119, "DIO Info In in"=w121) -> ("error out"=w90:errorcluster, "IN"=w118:bool, "DIO Info In out"=w120:T20)  [unwired: 7 in]
    n25 = call <vilib>:"NavX Open.vi"("I2C Channel"=I2C_Channel."A") -> ("error out"=w107:errorcluster, "NavX Info"=w109:T27)  [unwired: 9 in]
    n26 = Not(x="Red LED") -> (.not. x?=w79:bool)
    n27 = call "Digital Debounce Filter.vi"("Boolean input"=w118) -> ("Rising Edge"=→"Rising Edge":bool)  [unwired: 1 in, 2 out]
    n28 = call "Arduino Interfacing VI.vi"("AE Mode"=Arduino_Interfacing."Read From Arduino") -> ("error out"=w91:errorcluster, "Arduino Data"=w93:T15)  [unwired: 3 in]
    "Arduino Data" <- w93
    n29 = And(x=w79, y="Green LED") -> (x .and. y?=w82:bool)
    n30 = call <vilib>:"DIO Write.vi"("error in (no error)"=w101, "Input"=w82, "DIO Info In"=w102) -> ("error out"=w85:errorcluster, "DIO Info Out"=w100:T20)  [unwired: 7 in]
    n31 = Unbundle By Name(w93) -> ("Rotary Switch"=→"Task selection":u8)
    n32 = call "navX reading VI.vi"("NavX Info In"=w109, "Mode"=navX_type_def."Get i2C reference", "error in (no error)"=w107) -> ("NavX Info Out"=w98:T27, "Error Out"=w87:errorcluster)  [unwired: 2 out]
    n33 = call "navX reading VI.vi"("NavX Info In"=w98, "Mode"=navX_type_def."Read Values", "error in (no error)"=w87) -> ("NavX Info Out"=w97:T27, "NavX Readings"=→"NavX Readings":T14, "Status"=→"Status":T12, "Error Out"=w96:errorcluster)
    n34 = Merge Errors(w91, w90, w89, w88, w87, w86, w85) -> (w83:errorcluster)
    "General Errors" <- w83
    n35 = call "FGV Bool.vi"("Init/Read/Write State"=States_for_Action_Engine."Read") -> ("Output node"=w123:bool)  [unwired: 2 in, 1 out]
    n36 = Unbundle By Name(w83) -> ("status"=w80:bool)
    n37 = local write "Red LED"(w80) -> ()
    n38 = Wait (ms)(milliseconds to wait=u32 50) -> ()  [unwired: 1 out]
  }
  n39 = while {
    tunnel: w59 -> [w141]
    tunnel: w60 -> [w140]
    tunnel: [w139] -> w66
    tunnel: [w138] -> w65
    tunnel: w64 -> [w137]
    tunnel: [w136] -> w62
    tunnel: w63 -> [w135]
    tunnel: [w134] -> w61
    stop <- w132 stop-if-true
    # "Generate USER Event Loop"
    n40 = local read "Rising Edge"() -> (w129:bool)
    n41 = Or(x="OK Button", y=w129) -> (x .or. y?=w128:bool)
    n42 = local read "TASK ENABLE"() -> (w127:bool)
    n43 = And(x=w128, y=w127) -> (x .and. y?=w126:bool)
    n44 = case shown="True" w126 {
      selector: w126 -> [_ w152]
      tunnel: w141 -> [w151 w156]
      tunnel: [w151 w155] -> w138
      tunnel: w137 -> [w150 w154]
      tunnel: [w150 w153] -> w136
      frame False {
      }
      frame True {
        n45 = Generate User Event(user event=w156, event data cluster=w152, error in=w154) -> (user event out=w155:refnum<user-event>, error out=w153:errorcluster)  [unwired: 1 in]
      }
    }
    n46 = case shown="False" "STOP" {
      selector: "STOP" -> [_ w145]
      tunnel: w140 -> [w144 w149]
      tunnel: [w144 w148] -> w139
      tunnel: w135 -> [w143 w147]
      tunnel: [w143 w146] -> w134
      tunnel: [FALSE w145] -> w132
      frame False {
      }
      frame True {
        n47 = Generate User Event(user event=w149, event data cluster=w145, error in=w147) -> (user event out=w148:refnum<user-event>, error out=w146:errorcluster)  [unwired: 1 in]
      }
    }
    n48 = Wait (ms)(milliseconds to wait=u32 10) -> ()  [unwired: 1 out]
    n49 = call "FGV Bool.vi"("Init/Read/Write State"=States_for_Action_Engine."Write", "Input Node"=w132) -> ()  [unwired: 1 in, 2 out]
  }
  n50 = while {
    tunnel: w58 -> [w163]
    tunnel: [w162] -> w57
    tunnel: w45 -> [w160]
    tunnel: [w159] -> w56
    tunnel: w51 -> [w158]
    tunnel: [w157] -> w48
    stop <- w161 stop-if-true
    # "EVENT Handling Loop"
    n51 = event shown="[1] <Start Task>: User Event" {
      selector: w163 -> [_ _ _]
      dyn-events: [_ _ _] -> w162
      timeout: _ -> [_ _ _]
      tunnel: [FALSE FALSE w197] -> w161
      tunnel: w160 -> [w168 w177 w195]
      tunnel: [w167 w176 w196] -> w159
      tunnel: w158 -> [w166 w175 w194]
      tunnel: [w165 w174 w193] -> w157
      event Timeout {
        n52 = event-data() -> ()  [unwired: 1 in, 3 out]
        n53 = Enqueue Element(queue=w168, element=Intruction_Type_Definitions."Start Task 1" ("Enum"), error in (no error)=w166) -> (queue out=w167:refnum<queue>, error out=w165:errorcluster)  [unwired: 1 in, 1 out]
      }
      event User Event {
        n54 = event-data() -> ()  [unwired: 1 in, 5 out]
        n55 = call "Arduino Interfacing VI.vi"("AE Mode"=Arduino_Interfacing."Read From Arduino") -> ("Arduino Data"=w171:T15)  [unwired: 3 in, 1 out]
        n56 = Unbundle By Name(w171) -> ("Rotary Switch"=w170:u8)
        n57 = case shown="11" w170 {
          tunnel: [Intruction_Type_Definitions."Start Task 1" ("Enum") Intruction_Type_Definitions."Start Task 2" ("Enum") Intruction_Type_Definitions."Start Task 3" ("Enum") Intruction_Type_Definitions."Start Task 4" ("Enum") Intruction_Type_Definitions."Start Task 5" ("Enum") Intruction_Type_Definitions."Start Task 6" ("Enum") Intruction_Type_Definitions."Start Task 7" ("Enum") Intruction_Type_Definitions."Start Task 8 - BALL" ("Enum") Intruction_Type_Definitions."Start Task 8 - Soap" ("Enum") Intruction_Type_Definitions."Start Task 8 - Gel" ("Enum") Intruction_Type_Definitions."Start Task 8 - Pipe" ("Enum") Intruction_Type_Definitions."Start Task 9" ("Enum") Intruction_Type_Definitions."None" ("Enum")] -> w173
          frame 0, Default {
          }
          frame 1 {
          }
          frame 2 {
          }
          frame 3 {
          }
          frame 4 {
          }
          frame 5 {
          }
          frame 6 {
          }
          frame 7 {
          }
          frame 8 {
          }
          frame 9 {
          }
          frame 10 {
          }
          frame 11 {
          }
          frame 12 {
          }
        }
        "Selected Task" <- w173
        n58 = Enqueue Element(queue=w177, element=w173, error in (no error)=w175) -> (queue out=w176:refnum<queue>, error out=w174:errorcluster)  [unwired: 1 in, 1 out]
      }
      event User Event {
        n59 = event-data() -> ("Stop Queue"=w197:bool)  [unwired: 1 in, 4 out]
        n60 = Enqueue Element At Opposite End(queue=w195, element=Intruction_Type_Definitions."Exit" ("Enum"), error in (no error)=w194) -> (queue out=w196:refnum<queue>, error out=w193:errorcluster)  [unwired: 1 in, 1 out]
      }
    }
  }
  n61 = while {
    tunnel: w46 -> [w207]
    tunnel: w45 -> [w204]
    stop <- w201 stop-if-true
    # "Status Loop for Action Queues"
    n62 = Get Queue Status(queue=w207, return elements? (F)=TRUE) -> (error out=w203:errorcluster, # elements in queue=→"Action Queue Items":i32, elements=→"Action Queues items":string[])  [unwired: 1 in, 5 out]
    n63 = Get Queue Status(queue=w204, return elements? (F)=TRUE) -> (# pending remove=→"State Logic Queue Items":i32, error out=w202:errorcluster, elements=→"elements":T8[])  [unwired: 1 in, 5 out]
    n64 = Merge Errors(w203, w202) -> (w201:errorcluster)
    n65 = Wait (ms)(milliseconds to wait=u32 500) -> ()  [unwired: 1 out]
  }
  n66 = while {
    tunnel: w45 -> [w251]
    tunnel: w46 -> [w263]
    tunnel: w49 -> [w261]
    tunnel: [w260] -> _
    tunnel: [w259] -> w39
    shift-right: [w252] -> _
    shift-left: T7 {"PING_A"=0, "PING_B"=0, "PING_C"=0, "PING_D"=0} -> [w254]
    shift-right: [w245] -> _
    shift-left: State_Type_Definitions,_for_0.26g_versions_and_later_2."Startup" ("Enum") -> [w248]
    shift-right: [w241] -> _
    shift-left: T6 {"xDistance"=0.0, "yDistance"=0.0, "wDistance"=0.0} -> [w243]
    shift-right: [w238] -> _
    shift-left: _ -> [w237]
    shift-right: [w234] -> _
    shift-left: T9 {"Recognized Object"=FALSE, "Object X coordinate"=0.0, "Object Y coordinate"=0.0} -> [w236]
    shift-right: [w231] -> _
    shift-left: T5 {"y Stepper Position"=0, "z Stepper Position"=0} -> [w233]
    shift-right: [w228] -> _
    shift-left: T4 {"Yaw"=0.0, "Compass"=0.0} -> [w230]
    shift-right: [w225] -> _
    shift-left: T3 {"Time up flag"=FALSE, "SET TIME TO CHECK"=0.0} -> [w227]
    shift-right: [w223] -> _
    shift-left: T18 {"yStepper desired"=0} -> [w224]
    shift-right: [w219] -> _
    shift-left: T2 {"Left IR Sensor"=0.0, "Arm IR Sensor"=0.0, "Bottom IR Sensor"=0.0} -> [w221]
    shift-right: [w217] -> _
    shift-left: T17 {"ySpeed"=0.0, "xSpeed"=0.0, "wSpeed"=0.0} -> [w218]
    shift-right: [w214] -> _
    shift-left: T1 {"Line Detected?"=FALSE, "S1"=0.0, "S2"=0.0, "S3"=0.0, "S4"=0.0} -> [w216]
    shift-right: [w212] -> _
    shift-left: _ -> [w211]
    stop <- w250 stop-if-true
    # ">>Action Queue>>"
    # ">>State Logic Queue Reference >>"
    # ">>> Line Sensor Cluster>>>"
    # ">>> IR Sensors >>>"
    # ">>> Time cluster >>>"
    # ">>> Object detection >>>"
    # ">>> Yaw >>>"
    # ">>> Ultrasonic Sensors Detect >>>"
    # ">>> Encoders >>>"
    # ">>> Stepper position >>>"
    # ">>State Logic  >>"
    # ">> Item Selection Bias >>"
    # ">> Item Selection Bias >>"
    # ">> Item Selection Bias >>"
    # ">>State Logic  >>"
    # ">>> Motor control cluster >>>"
    # ">>> yStepper command>>>"
    # ">>True Stop Next State >>"
    # ">>Error  >>"
    # ">>Timeout>>"
    # ">>Action states Queue Reference >>"
    # ">>State Logic Queue Reference >>"
    # "TOP LEVEL BASELINE (MAIN PROCESSING LOOP)"
    n67 = Wait (ms)(milliseconds to wait=u32 20) -> ()  [unwired: 1 out]
    n68 = Dequeue Element(queue=w263, timeout in ms (-1)=0, error in (no error)=w261) -> (queue out=w255:refnum<queue>, element=w262:string, error out=w256:errorcluster)  [unwired: 1 out]
    "Action State" <- w262
    n69 = case shown="\"OPEN CLAW\"" w262 {
      tunnel: [_ _ _ _ _ _ _ _ _ _ _ _ _ _ _ _ _ _ _ _ 0 w3075 _ _ _ _ _ _ _ _ _ _ _ _ _ _ _ _ _ _ _ _ _ _ _ _ _ _ _ _ _ _ _] -> w258
      tunnel: w255 -> [_ _ _ _ _ _ _ _ _ _ _ _ _ _ _ _ _ _ _ _ _ _ _ _ _ _ _ _ _ _ _ _ _ _ _ _ _ _ _ _ _ _ _ _ _ _ _ _ _ _ _ _ _]
      tunnel: w254 -> [w2771 w2782 w2796 w2809 w2828 w2842 w2855 w2868 w2883 w2897 w2910 w2919 w2936 w2952 w2966 w2978 w3001 w3010 w3039 w3051 w3064 w3076 w3087 w3099 w3116 w3150 w3186 w3199 w3209 w3220 w3232 w3246 w3261 w3272 w3283 w3302 w3312 w3327 w3336 w3348 w3360 w3372 w3381 w3398 w3407 w3425 w3433 w3447 w3461 w3475 w3489 w3503 w3516]
      tunnel: [w2771 w2782 w2796 w2809 w2828 w2842 w2855 w2868 w2883 w2897 w2910 w2919 w2936 w2953 w2966 w2978 w3001 w3010 w3040 w3051 w3064 w3076 w3087 w3099 w3116 w3149 w3185 w3199 w3209 w3220 w3232 w3246 w3261 w3272 w3283 w3302 w3312 w3327 w3336 w3348 w3360 w3372 w3381 w3398 w3407 w3425 w3433 w3447 w3461 w3475 w3489 w3503 w3516] -> w253
      tunnel: [TRUE TRUE _ _ _ _ _ _ _ _ _ _ _ _ _ _ _ _ _ _ _ _ _ _ _ _ _ _ _ _ _ _ _ _ _ _ _ _ _ _ _ _ _ _ _ _ _ _ _ _ _ _ _] -> w250
      tunnel: w248 -> [w2769 w2780 w2795 w2808 w2827 w2841 w2854 w2867 w2882 w2896 w2909 w2918 w2935 w2951 w2965 w2976 w2994 w3009 w3038 w3050 w3061 w3073 w3086 w3098 w3115 w3148 w3184 w3198 w3208 w3219 w3224 w3245 w3260 w3271 w3282 w3301 w3311 w3321 w3335 w3347 w3359 w3371 w3380 w3389 w3406 w3424 w3432 w3446 w3460 w3474 w3488 w3502 w3515]
      tunnel: [_ _ _ _ _ _ _ _ _ _ _ _ _ _ _ _ _ _ _ _ _ TRUE _ _ _ _ _ _ _ _ _ _ _ _ _ _ _ _ _ _ _ _ _ _ _ _ _ _ _ _ _ _ _] -> w247
      tunnel: [w2769 w2780 w2795 w2808 w2827 w2841 w2854 w2867 w2882 w2896 w2909 w2918 w2935 w2951 w2965 w2976 w2994 w3009 w3038 w3050 w3061 w3073 w3086 w3098 w3115 w3148 w3184 w3198 w3208 w3219 w3224 w3245 w3260 w3271 w3282 w3301 w3311 w3321 w3335 w3347 w3359 w3371 w3380 w3389 w3406 w3424 w3432 w3446 w3460 w3474 w3488 w3502 w3515] -> w246
      tunnel: w243 -> [w2768 w2779 w2794 w2811 w2826 w2840 w2853 w2866 w2881 w2895 w2908 w2920 w2934 w2950 w2967 w2980 w2996 w3011 w3037 w3052 w3060 w3072 w3088 w3100 w3111 w3139 w3174 w3197 w3211 w3221 w3229 w3247 w3262 w3273 w3284 w3303 w3314 w3325 w3338 w3350 w3362 w3374 w3383 w3393 w3409 w3427 w3435 w3449 w3463 w3477 w3491 w3505 w3518]
      tunnel: [w2768 w2779 w2794 w2811 w2826 w2840 w2853 w2866 w2881 w2895 w2908 w2920 w2933 w2950 w2967 w2980 w2996 w3011 w3036 w3052 w3060 w3072 w3088 w3100 w3111 w3138 w3173 w3197 w3211 w3221 w3229 w3247 w3262 w3273 w3284 w3303 w3314 w3325 w3338 w3350 w3362 w3374 w3383 w3393 w3409 w3427 w3435 w3449 w3463 w3477 w3491 w3505 w3518] -> w242
      tunnel: w236 -> [w2767 w2778 w2793 w2810 w2825 w2839 w2852 w2865 w2880 w2894 w2906 w2917 w2932 w2949 w2960 w2979 w2995 w3008 w3028 w3049 w3059 w3071 w3085 w3097 w3114 w3143 w3179 w3195 w3210 w3218 w3230 w3244 w3259 w3267 w3281 w3297 w3313 w3326 w3337 w3349 w3361 w3373 w3382 w3392 w3408 w3426 w3434 w3448 w3462 w3476 w3490 w3504 w3517]
      tunnel: [w2767 w2778 w2793 w2810 w2825 w2839 w2852 w2865 w2880 w2894 w2906 w2917 w2932 w2949 w2960 w2979 w2995 w3008 w3027 w3049 w3059 w3071 w3085 w3097 w3113 w3142 w3178 w3195 w3210 w3218 w3230 w3244 w3259 w3267 w3281 w3296 w3313 w3326 w3337 w3349 w3361 w3373 w3382 w3392 w3408 w3426 w3434 w3448 w3462 w3476 w3490 w3504 w3517] -> w235
      tunnel: w233 -> [w2766 w2777 w2792 w2812 w2824 w2838 w2851 w2864 w2879 w2893 w2905 w2916 w2931 w2948 w2968 w2981 w2997 w3007 w3033 w3048 w3058 w3070 w3084 w3096 w3110 w3134 w3169 w3194 w3207 w3217 w3228 w3243 w3258 w3270 w3280 w3304 w3315 w3324 w3334 w3346 w3358 w3370 w3384 w3394 w3410 w3423 w3436 w3450 w3464 w3478 w3492 w3506 w3519]
      tunnel: [w2766 w2777 w2792 w2812 w2824 w2838 w2851 w2864 w2879 w2893 w2905 w2916 w2931 w2948 w2968 w2981 w2997 w3007 w3032 w3048 w3058 w3070 w3084 w3096 w3110 w3133 w3168 w3194 w3207 w3217 w3228 w3243 w3258 w3270 w3280 w3304 w3315 w3324 w3334 w3346 w3358 w3370 w3384 w3394 w3410 w3422 w3436 w3450 w3464 w3478 w3492 w3506 w3519] -> w232
      tunnel: w230 -> [w2765 w2776 w2790 w2813 w2822 w2836 w2849 w2863 w2877 w2891 w2904 w2915 w2930 w2941 w2963 w2982 w2998 w3006 w3023 w3047 w3057 w3069 w3083 w3095 w3109 w3130 w3165 w3193 w3204 w3216 w3227 w3242 w3257 w3269 w3279 w3305 w3316 w3323 w3333 w3343 w3355 w3367 w3385 w3395 w3411 w3417 w3437 w3451 w3465 w3479 w3493 w3507 w3520]
      tunnel: [w2765 w2776 w2790 w2813 w2822 w2836 w2849 w2863 w2877 w2891 w2904 w2915 w2930 w2941 w2962 w2982 w2998 w3006 w3022 w3047 w3057 w3069 w3083 w3095 w3109 w3129 w3164 w3193 w3204 w3216 w3227 w3242 w3257 w3269 w3279 w3305 w3316 w3323 w3333 w3343 w3355 w3367 w3385 w3395 w3411 w3417 w3437 w3451 w3465 w3479 w3493 w3507 w3520] -> w229
      tunnel: w227 -> [w2763 w2775 w2791 w2814 w2823 w2837 w2850 w2862 w2878 w2892 w2903 w2914 w2929 w2940 w2959 w2983 w2999 w3005 w3019 w3044 w3056 w3068 w3082 w3094 w3108 w3127 w3162 w3191 w3203 w3215 w3226 w3241 w3256 w3268 w3278 w3306 w3317 w3322 w3332 w3342 w3354 w3366 w3386 w3396 w3412 w3416 w3431 w3445 w3459 w3473 w3487 w3501 w3514]
      tunnel: [w2763 w2775 w2791 w2814 w2823 w2837 w2850 w2862 w2878 w2892 w2903 w2914 w2929 w2940 w2959 w2983 w2999 w3005 w3019 w3044 w3056 w3068 w3082 w3094 w3107 w3126 w3161 w3191 w3203 w3215 w3226 w3241 w3256 w3268 w3278 w3306 w3317 w3322 w3332 w3342 w3354 w3366 w3386 w3396 w3412 w3416 w3431 w3443 w3457 w3471 w3485 w3499 w3513] -> w226
      tunnel: w224 -> [_ _ _ _ _ _ _ _ _ _ _ _ _ _ _ _ _ _ _ _ _ _ _ _ _ _ _ _ _ _ _ _ _ _ _ _ _ _ _ _ _ _ _ _ w3403 _ _ _ _ _ _ _ _]
      tunnel: [w2762 w2774 w2785 w2804 w2817 w2831 w2845 w2858 w2873 w2886 w2900 w2913 w2923 w2939 w2956 w2974 w3000 w3004 w3016 w3043 w3055 w3067 w3081 w3091 w3101 w3120 w3153 w3190 w3202 w3214 w3231 w3235 w3250 w3265 w3276 w3290 w3309 w3328 w3331 w3341 w3353 w3365 w3377 w3397 w3401 w3415 w3430 w3440 w3454 w3468 w3482 w3496 w3510] -> w220
      tunnel: w221 -> [w2762 w2774 w2785 w2804 w2817 w2831 w2845 w2858 w2873 w2886 w2900 w2913 w2923 w2939 w2956 w2975 w3000 w3004 w3016 w3043 w3055 w3067 w3081 w3091 w3101 w3121 w3154 w3190 w3202 w3214 w3231 w3235 w3250 w3265 w3276 w3290 w3309 w3328 w3331 w3341 w3353 w3365 w3377 w3397 w3401 w3415 w3430 w3440 w3454 w3468 w3482 w3496 w3510]
      tunnel: w218 -> [_ _ _ _ _ _ _ _ w2872 _ _ _ _ _ _ _ _ _ _ _ _ _ _ _ _ _ _ _ _ _ _ _ _ _ _ _ _ _ _ _ _ _ _ _ _ _ _ _ _ _ _ _ _]
      tunnel: w216 -> [w2761 w2773 w2784 w2798 w2816 w2830 w2844 w2857 w2870 w2885 w2899 w2912 w2922 w2938 w2955 w2970 w2993 w3003 w3014 w3042 w3054 w3066 w3080 w3090 w3104 w3123 w3157 w3189 w3201 w3213 w3223 w3234 w3249 w3264 w3275 w3287 w3308 w3319 w3330 w3340 w3352 w3364 w3376 w3388 w3400 w3414 w3429 w3439 w3453 w3467 w3481 w3495 w3509]
      tunnel: [w2761 w2773 w2784 w2798 w2816 w2830 w2844 w2857 w2870 w2885 w2899 w2912 w2922 w2938 w2955 w2970 w2992 w3003 w3014 w3042 w3054 w3066 w3080 w3090 w3103 w3122 w3156 w3189 w3201 w3213 w3223 w3234 w3249 w3264 w3275 w3287 w3308 w3319 w3330 w3340 w3352 w3364 w3376 w3388 w3400 w3414 w3429 w3439 w3453 w3467 w3481 w3495 w3509] -> w215
      tunnel: [_ _ _ _ _ _ _ _ _ _ _ _ _ _ _ _ _ _ _ _ _ _ _ _ _ _ _ _ _ _ _ _ _ _ _ w3286 _ _ _ _ _ _ _ _ _ _ _ _ _ _ _ _ _] -> w213
      tunnel: w211 -> [w2760 w2772 w2783 w2797 w2815 w2829 w2843 w2856 w2869 w2884 w2898 w2911 w2921 w2937 w2954 w2969 w2984 w3002 w3012 w3041 w3053 w3065 w3079 w3089 w3105 w3124 w3158 w3188 w3200 w3212 w3222 w3233 w3248 w3263 w3274 w3285 w3307 w3318 w3329 w3339 w3351 w3363 w3375 w3387 w3399 w3413 w3428 w3438 w3452 w3466 w3480 w3494 w3508]
      tunnel: [w2760 w2772 w2783 w2797 w2815 w2829 w2843 w2856 w2869 w2884 w2898 w2911 w2921 w2937 w2954 w2969 w2984 w3002 w3012 w3041 w3053 w3065 w3079 w3089 w3105 w3124 w3158 w3188 w3200 w3212 w3222 w3233 w3248 w3263 w3274 w3285 w3307 w3318 w3329 w3339 w3351 w3363 w3375 w3387 w3399 w3413 w3428 w3438 w3452 w3466 w3480 w3494 w3508] -> w210
      frame "Exit" {
        # ">>State Logic  >>"
        # ">>> Time cluster >>>"
        # ">>> Yaw >>>"
        # ">>> Stepper position >>>"
        # ">>> Encoders >>>"
        # ">>> Object detection >>>"
        # ">>> Ultrasonic Sensors Detect >>>"
        n70 = call "Imaq Dispose"("All Images? (No)"=TRUE) -> ()  [unwired: 5 in, 1 out]
      }
      frame "----Movement States----" {
        # ">>State Logic  >>"
        # ">>> Time cluster >>>"
        # ">>> Yaw >>>"
        # ">>> Stepper position >>>"
        # ">>> Encoders >>>"
        # ">>> Object detection >>>"
        # ">>> Ultrasonic Sensors Detect >>>"
      }
      frame "FORWARD" {
        # ">>State Logic  >>"
        # ">>> Time cluster >>>"
        # ">>> Yaw >>>"
        # ">>> Stepper position >>>"
        # ">>> Encoders >>>"
        # ">>> Object detection >>>"
        # ">>> Ultrasonic Sensors Detect >>>"
        n71 = Unbundle By Name(w2790) -> ("Yaw"=w2786:dbl)
        n72 = call "MOTOR CONTROL WITH PID AE.vi"("Yaw"=w2786, "Speed"=50.0, "Direction"=MOTOR_CONTROL_WITH_PID_AE_DIRECTION_TYPE_DEF."y-axis movement", "AE Mode"=MOTOR_CONTROL_WITH_PID_AE_DATA_MODE_TYPE_DEF."Write to AE") -> ()  [unwired: 1 out]
      }
      frame "FORWARD - IR ASSIST" {
        # ">>State Logic  >>"
        # ">>> Time cluster >>>"
        # ">>> Yaw >>>"
        # ">>> Stepper position >>>"
        # ">>> Encoders >>>"
        # ">>> Object detection >>>"
        # ">>> Ultrasonic Sensors Detect >>>"
        n73 = Unbundle By Name(w2804) -> ("Left IR Sensor"=w2803:dbl)
        n74 = Subtract(x=w2803, y=20.0) -> (x-y=w2801:dbl)
        n75 = Multiply(x=w2801, y=0.25) -> (x*y=w2799:dbl)
        n76 = call "MOTOR CONTROL WITH PID AE.vi"("Yaw"=w2799, "Speed"=30.0, "Direction"=MOTOR_CONTROL_WITH_PID_AE_DIRECTION_TYPE_DEF."y-axis movement", "AE Mode"=MOTOR_CONTROL_WITH_PID_AE_DATA_MODE_TYPE_DEF."Write to AE") -> ()  [unwired: 1 out]
      }
      frame "LEFT" {
        # ">>State Logic  >>"
        # ">>> Time cluster >>>"
        # ">>> Yaw >>>"
        # ">>> Stepper position >>>"
        # ">>> Encoders >>>"
        # ">>> Object detection >>>"
        # ">>> Ultrasonic Sensors Detect >>>"
        n77 = Unbundle By Name(w2822) -> ("Yaw"=w2819:dbl)
        n78 = call "MOTOR CONTROL WITH PID AE.vi"("Yaw"=w2819, "Speed"=-20.0, "Direction"=MOTOR_CONTROL_WITH_PID_AE_DIRECTION_TYPE_DEF."x-axis movement", "AE Mode"=MOTOR_CONTROL_WITH_PID_AE_DATA_MODE_TYPE_DEF."Write to AE") -> ()  [unwired: 1 out]
      }
      frame "RIGHT" {
        # ">>> Time cluster >>>"
        # ">>> Yaw >>>"
        # ">>> Stepper position >>>"
        # ">>> Encoders >>>"
        # ">>> Object detection >>>"
        # ">>> Ultrasonic Sensors Detect >>>"
        n79 = Unbundle By Name(w2836) -> ("Yaw"=w2832:dbl)
        n80 = call "MOTOR CONTROL WITH PID AE.vi"("Yaw"=w2832, "Speed"=20.0, "Direction"=MOTOR_CONTROL_WITH_PID_AE_DIRECTION_TYPE_DEF."x-axis movement", "AE Mode"=MOTOR_CONTROL_WITH_PID_AE_DATA_MODE_TYPE_DEF."Write to AE") -> ()  [unwired: 1 out]
      }
      frame "R-ACW" {
        # ">>> IR Sensors >>>"
        # ">>> Time cluster >>>"
        # ">>> Yaw >>>"
        # ">>> Stepper position >>>"
        # ">>> Encoders >>>"
        # ">>> Object detection >>>"
        # ">>> Ultrasonic Sensors Detect >>>"
        n81 = call "MOTOR CONTROL WITH PID AE.vi"("Speed"=10.0, "Direction"=MOTOR_CONTROL_WITH_PID_AE_DIRECTION_TYPE_DEF."rotation", "AE Mode"=MOTOR_CONTROL_WITH_PID_AE_DATA_MODE_TYPE_DEF."Write to AE") -> ()  [unwired: 1 in, 1 out]
      }
      frame "R-CW" {
        (unwired) -0.2 ("Speed")
        # ">>> Time cluster >>>"
        # ">>> Yaw >>>"
        # ">>> Stepper position >>>"
        # ">>> Encoders >>>"
        # ">>> Object detection >>>"
        # ">>> Ultrasonic Sensors Detect >>>"
        n82 = call "MOTOR CONTROL WITH PID AE.vi"("Speed"=-10.0, "Direction"=MOTOR_CONTROL_WITH_PID_AE_DIRECTION_TYPE_DEF."rotation", "AE Mode"=MOTOR_CONTROL_WITH_PID_AE_DATA_MODE_TYPE_DEF."Write to AE") -> ()  [unwired: 1 in, 1 out]
      }
      frame "X AXIS - SLOW" {
        # ">>> Line Sensor Cluster>>>"
        # ">>> IR Sensors >>>"
        # ">>> Time cluster >>>"
        # ">>> Yaw >>>"
        # ">>> Stepper position >>>"
        # ">>> Encoders >>>"
        # ">>> Object detection >>>"
        # ">>> Ultrasonic Sensors Detect >>>"
        n83 = Unbundle By Name(w2872) -> ("xSpeed"=w2871:dbl)
        n84 = Unbundle By Name(w2877) -> ("Yaw"=w2874:dbl)
        n85 = call "MOTOR CONTROL WITH PID AE.vi"("Yaw"=w2874, "Speed"=w2871, "Direction"=MOTOR_CONTROL_WITH_PID_AE_DIRECTION_TYPE_DEF."x-axis movement", "AE Mode"=MOTOR_CONTROL_WITH_PID_AE_DATA_MODE_TYPE_DEF."Write to AE") -> ()  [unwired: 1 out]
      }
      frame "REVERSE" {
        # ">>> Time cluster >>>"
        # ">>> Yaw >>>"
        # ">>> Stepper position >>>"
        # ">>> Encoders >>>"
        # ">>> Object detection >>>"
        # ">>> Ultrasonic Sensors Detect >>>"
        n86 = Unbundle By Name(w2891) -> ("Yaw"=w2887:dbl)
        n87 = call "MOTOR CONTROL WITH PID AE.vi"("Yaw"=w2887, "Speed"=-50.0, "Direction"=MOTOR_CONTROL_WITH_PID_AE_DIRECTION_TYPE_DEF."y-axis movement", "AE Mode"=MOTOR_CONTROL_WITH_PID_AE_DATA_MODE_TYPE_DEF."Write to AE") -> ()  [unwired: 1 out]
      }
      frame "STOP" {
        n88 = Wait (ms)(milliseconds to wait=u32 100) -> ()  [unwired: 1 out]
        n89 = call "MOTOR CONTROL WITH PID AE.vi"("Direction"=MOTOR_CONTROL_WITH_PID_AE_DIRECTION_TYPE_DEF."stop", "AE Mode"=MOTOR_CONTROL_WITH_PID_AE_DATA_MODE_TYPE_DEF."Write to AE") -> ()  [unwired: 2 in, 1 out]
      }
      frame "----SENSOR READING---- " {
      }
      frame "READ ENCODERS" {
        # ">>> Time cluster >>>"
        # ">>> Yaw >>>"
        # ">>> Stepper position >>>"
        # ">>> Object detection >>>"
        # ">>> Current encoder distance >>>"
        # ">>> Ultrasonic Sensors Detect >>>"
        n90 = call "MOTOR CONTROL WITH PID AE.vi"("AE Mode"=MOTOR_CONTROL_WITH_PID_AE_DATA_MODE_TYPE_DEF."Read from AE") -> ("Speed & distance"=w2927:T13)  [unwired: 3 in]
        n91 = Unbundle By Name(w2927) -> ("xDistance"=w2926:dbl, "yDistance"=w2925:dbl, "wDistance"=w2924:dbl)
        n92 = Bundle By Name(cluster=w2934, "xDistance"=w2926, "yDistance"=w2925, "wDistance"=w2924) -> (w2933:T6)
      }
      frame "READ ULTRASONIC" {
        (unwired) navX_type_def."Read Values" ("Mode")
        (unwired) MOTOR_CONTROL_NO_PID_Type_Def."Latch" ("Direction")
        # ">>> Line Sensor Cluster>>>"
        # ">>> IR Sensors >>>"
        # ">>State Logic  >>"
        # ">>> Time cluster >>>"
        # ">>> Ultrasonic Sensors Detect >>>"
        # ">>> Object detection >>>"
        # ">>> Encoders >>>"
        # ">>> Stepper position >>>"
        # ">>> Yaw >>>"
        n93 = call "Arduino Interfacing VI.vi"("AE Mode"=Arduino_Interfacing."Read From Arduino") -> ("Arduino Data"=w2946:T15)  [unwired: 3 in, 1 out]
        n94 = Unbundle By Name(w2946) -> ("PING A"=w2945:u8, "PING B"=w2944:u8, "PING C"=w2943:u8, "PING D"=w2942:u8)
        n95 = Bundle By Name(cluster=w2952, "PING_A"=w2945, "PING_B"=w2944, "PING_C"=w2943, "PING_D"=w2942) -> (w2953:T7)
      }
      frame "READ NAVX" {
        # ">> Item Selection Bias >>"
        # ">>State Logic  >>"
        # ">>> Line Sensor Cluster>>>"
        # ">>> IR Sensors >>>"
        # ">>> Time cluster >>>"
        # ">>> Yaw >>>"
        # ">>> Ultrasonic Sensors Detect >>>"
        # ">>> Object detection >>>"
        # ">>> Encoders >>>"
        # ">>> Stepper position >>>"
        n96 = call "navX reading VI.vi"("Mode"=navX_type_def."Read Values") -> ("NavX Readings"=w2958:T14)  [unwired: 2 in, 3 out]
        n97 = Unbundle By Name(w2958) -> ("Heading"=w2957:dbl)
        n98 = Unbundle By Name(w2958) -> ("Yaw"=w2961:dbl)
        n99 = Bundle By Name(cluster=w2963, "Yaw"=w2961, "Compass"=w2957) -> (w2962:T4)
      }
      frame "READ IR" {
        w2972 = T38 [enum."B/AI1"] items=["Not Connected", "AudioIn/Left", "AudioIn/Right", "C/AI0", "C/AI1", "A/AI0", "A/AI1", "A/AI2", "A/AI3", "A/AI4", "A/AI5", "A/AI6", "A/AI7", "B/AI0", "B/AI1", "B/AI2", "B/AI3", "B/AI4", "B/AI5", "B/AI6", "B/AI7", "AI/AI0", "AI/AI1", "AI/AI2", "AI/AI3", "A/AI0 (DIFF)", "A/AI1 (DIFF)", "A/AI2 (DIFF)", "A/AI3 (DIFF)", "B/AI0 (DIFF)", "B/AI1 (DIFF)", "B/AI2 (DIFF)", "B/AI3 (DIFF)"] ("AI Channel")
        w2977 = T38 [enum."B/AI0"] items=["Not Connected", "AudioIn/Left", "AudioIn/Right", "C/AI0", "C/AI1", "A/AI0", "A/AI1", "A/AI2", "A/AI3", "A/AI4", "A/AI5", "A/AI6", "A/AI7", "B/AI0", "B/AI1", "B/AI2", "B/AI3", "B/AI4", "B/AI5", "B/AI6", "B/AI7", "AI/AI0", "AI/AI1", "AI/AI2", "AI/AI3", "A/AI0 (DIFF)", "A/AI1 (DIFF)", "A/AI2 (DIFF)", "A/AI3 (DIFF)", "B/AI0 (DIFF)", "B/AI1 (DIFF)", "B/AI2 (DIFF)", "B/AI3 (DIFF)"] ("AI Channel")
        # ">>State Logic  >>"
        # ">>> Time cluster >>>"
        # ">>> Ultrasonic Sensors Detect >>>"
        # ">>> Object detection >>>"
        # ">>> Encoders >>>"
        # ">>> Stepper position >>>"
        # ">>> Yaw >>>"
        n100 = call <vilib>:"Sharp IR.vi"("AI Channel"=w2972) -> ("Sharp IR Distance"=w2971:dbl)  [unwired: 8 in, 2 out]
        n101 = call <vilib>:"Sharp IR.vi"("AI Channel"=w2977) -> ("Sharp IR Distance"=w2973:dbl)  [unwired: 8 in, 2 out]
        n102 = Bundle By Name(cluster=w2975, "Left IR Sensor"=w2973, "Arm IR Sensor"=w2971) -> (w2974:T2)
      }
      frame "READ LINE SENSOR" {
        # ">>> IR Sensors >>>"
        # ">>> Line Sensor Cluster>>>"
        # ">>State Logic  >>"
        # ">>> Time cluster >>>"
        # ">>> Object detection >>>"
        # ">>> Yaw >>>"
        # ">>> Ultrasonic Sensors Detect >>>"
        # ">>> Encoders >>>"
        # ">>> Stepper position >>>"
        n103 = call "Line Sensor AE.vi"("AE State"=Line_Sensor_AE_Type_Def."READ FROM LINE SENSORS") -> ("Line Detected?"=w2990:bool, "Line Sensor Raw Values"=w2989:T40)
        n104 = Unbundle By Name(w2989) -> ("S1"=w2988:dbl, "S2"=w2987:dbl, "S3"=w2986:dbl, "S4"=w2985:dbl)
        n105 = Bundle By Name(cluster=w2993, "Line Detected?"=w2990, "S1"=w2988, "S2"=w2987, "S3"=w2986, "S4"=w2985) -> (w2992:T1)
      }
      frame "----SYSTEM MODES----" {
        (unwired) I2C_MASTER_Type_Def."Last State" ("Arduino Mode")
        # ">>> Object detection >>>"
        # ">>> Yaw >>>"
        # ">>> Ultrasonic Sensors Detect >>>"
        # ">>> Encoders >>>"
        # ">>> Stepper position >>>"
      }
      frame "INIT" {
        w3034 = u8 0
        w3035 = 0.0
        # ">>> IR Sensors >>>"
        # ">>> IR Sensors >>>"
        # ">>> Line Sensor Cluster>>>"
        # ">>> Time cluster >>>"
        # ">>> Object detection >>>"
        # ">>> Yaw >>>"
        # ">>> Ultrasonic Sensors Detect >>>"
        # ">>> Encoders >>>"
        # ">>> Stepper position >>>"
        # ">>State Logic  >>"
        n106 = call "Arduino Interfacing VI.vi"("AE Mode"=Arduino_Interfacing."Initialize") -> ()  [unwired: 3 in, 2 out]
        n107 = call "FGV Bool.vi"("Init/Read/Write State"=States_for_Action_Engine."Initialize") -> ()  [unwired: 2 in, 2 out]
        n108 = call "Elasped Timer.vi"("Action"=Elapsed_timer_control."Initialize") -> ()  [unwired: 7 in, 4 out]
        n109 = call "MOTOR CONTROL WITH PID AE.vi"("AE Mode"=MOTOR_CONTROL_WITH_PID_AE_DATA_MODE_TYPE_DEF."Init AE") -> ()  [unwired: 3 in, 1 out]
        n110 = call "IMAQ Reference AE.vi"("IMAQ AE States"=IMAQ_Reference_AE."Initialize AE") -> ()  [unwired: 1 in, 2 out]
        n111 = call "Line Sensor AE.vi"("AE State"=Line_Sensor_AE_Type_Def."INIT AE") -> ()  [unwired: 2 out]
        n112 = Bundle By Name(cluster=w3028, "Recognized Object"=FALSE, "Object X coordinate"=0.0, "Object Y coordinate"=0.0) -> (w3027:T9)
        n113 = Bundle By Name(cluster=w3033, "y Stepper Position"=u8 0, "z Stepper Position"=u8 0) -> (w3032:T5)
        n114 = Bundle By Name(cluster=w3037, "xDistance"=w3035, "yDistance"=w3035, "wDistance"=w3035) -> (w3036:T6)
        n115 = Bundle By Name(cluster=w3039, "PING_A"=w3034, "PING_B"=w3034, "PING_C"=w3034, "PING_D"=w3034) -> (w3040:T7)
        n116 = Bundle By Name(cluster=w3023, "Yaw"=0.0) -> (w3022:T4)
      }
      frame "ARDUINO - ULTRASONIC" {
        # ">>> Time cluster >>>"
        # ">>> Line Sensor Cluster>>>"
        # ">>> Object detection >>>"
        # ">>> Yaw >>>"
        # ">>> Ultrasonic Sensors Detect >>>"
        # ">>> Encoders >>>"
        # ">>> Stepper position >>>"
        # ">>State Logic  >>"
        n117 = call "Arduino Interfacing VI.vi"("Data to Write"=I2C_MASTER_WRITE_NEW_Type_Def."Ultrasonic sensors", "AE Mode"=Arduino_Interfacing."Write to Arduino") -> ()  [unwired: 2 in, 2 out]
      }
      frame "NAVX CALIBRATE" {
        # ">>> Object detection >>>"
        # ">>> Yaw >>>"
        # ">>> Ultrasonic Sensors Detect >>>"
        # ">>> Encoders >>>"
        # ">>> Stepper position >>>"
        # ">>State Logic  >>"
        # "Adds a 15 second delay to the startup process \nfor the NavX to calibrate"
        n118 = Wait (ms)(milliseconds to wait=u32 1000) -> ()  [unwired: 1 out]
      }
      frame "NO ACTION", Default {
        (unwired) u8 0 ("y Stepper value")
        (unwired) TRUE ("Latch")
        (unwired) navX_type_def."Read Values" ("Mode")
        (unwired) MOTOR_CONTROL_NO_PID_Type_Def."Latch" ("Direction")
        # ">>> Object detection >>>"
        # ">>> Yaw >>>"
        # ">>> Ultrasonic Sensors Detect >>>"
        # ">>> Encoders >>>"
        # ">>> Stepper position >>>"
        # ">>State Logic  >>"
        n119 = case shown="4" w3073 {
          tunnel: [0 100] -> w3075
          frame 1, Default {
          }
          frame 4 {
          }
        }
      }
      frame "----RESET CASES----" {
        (unwired) I2C_MASTER_Type_Def."Last State" ("Arduino Mode")
        # ">>> Object detection >>>"
        # ">>> Yaw >>>"
        # ">>> Ultrasonic Sensors Detect >>>"
        # ">>> Encoders >>>"
        # ">>> Stepper position >>>"
        # ">>State Logic  >>"
      }
      frame "RESET ENCODERS" {
        # ">>> Object detection >>>"
        # ">>> Yaw >>>"
        # ">>> Ultrasonic Sensors Detect >>>"
        # ">>> Encoders >>>"
        # ">>> Stepper position >>>"
        # ">>State Logic  >>"
        n120 = call "MOTOR CONTROL WITH PID AE.vi"("Direction"=MOTOR_CONTROL_WITH_PID_AE_DIRECTION_TYPE_DEF."reset encoders", "AE Mode"=MOTOR_CONTROL_WITH_PID_AE_DATA_MODE_TYPE_DEF."Write to AE") -> ()  [unwired: 2 in, 1 out]
      }
      frame "RESET FLAGS" {
        # ">>> Line Sensor Cluster>>>"
        # ">>> IR Sensors >>>"
        # ">>> Time cluster >>>"
        # ">>> Object detection >>>"
        # ">>> Yaw >>>"
        # ">>> Ultrasonic Sensors Detect >>>"
        # ">>> Encoders >>>"
        # ">>> Stepper position >>>"
        # ">>> Line Sensor Cluster>>>"
        # ">>> IR Sensors >>>"
        # ">>> Time cluster >>>"
        # ">>> Object detection >>>"
        # ">>> Yaw >>>"
        # ">>> Ultrasonic Sensors Detect >>>"
        # ">>> Encoders >>>"
        # ">>> Stepper position >>>"
        # "Resets BOOLEAN FLAGS only"
        n121 = Wait (ms)(milliseconds to wait=u32 20) -> ()  [unwired: 1 out]
        n122 = Bundle By Name(cluster=w3114, "Recognized Object"=FALSE) -> (w3113:T9)
        n123 = Bundle By Name(cluster=w3104, "Line Detected?"=FALSE) -> (w3103:T1)
        n124 = Bundle By Name(cluster=w3108, "Time up flag"=FALSE) -> (w3107:T3)
      }
      frame "RESET SENSOR VALUES" {
        w3118 = 0.0 ("S4")
        w3119 = 0.0 ("S4")
        # "Resets SENSOR VALUES only"
        # ">>> Line Sensor Cluster>>>"
        # ">>> IR Sensors >>>"
        # ">>> Time cluster >>>"
        # ">>> Object detection >>>"
        # ">>> Yaw >>>"
        # ">>> Ultrasonic Sensors Detect >>>"
        # ">>> Encoders >>>"
        # ">>> Stepper position >>>"
        # ">>> Line Sensor Cluster>>>"
        # ">>> IR Sensors >>>"
        # ">>> Time cluster >>>"
        # ">>> Object detection >>>"
        # ">>> Yaw >>>"
        # ">>> Ultrasonic Sensors Detect >>>"
        # ">>> Encoders >>>"
        # ">>> Stepper position >>>"
        # "Resets any software variables\nand/or non-critical states"
        n125 = Wait (ms)(milliseconds to wait=u32 20) -> ()  [unwired: 1 out]
        n126 = Bundle By Name(cluster=w3127, "SET TIME TO CHECK"=0.0) -> (w3126:T3)
        n127 = Bundle By Name(cluster=w3143, "Object X coordinate"=0.0, "Object Y coordinate"=0.0) -> (w3142:T9)
        n128 = Bundle By Name(cluster=w3134, "y Stepper Position"=u8 0, "z Stepper Position"=u8 0) -> (w3133:T5)
        n129 = Bundle By Name(cluster=w3121, "Left IR Sensor"=w3118, "Arm IR Sensor"=w3118) -> (w3120:T2)
        n130 = Bundle By Name(cluster=w3139, "xDistance"=0.0, "yDistance"=0.0, "wDistance"=0.0) -> (w3138:T6)
        n131 = Bundle By Name(cluster=w3150, "PING_A"=u8 0, "PING_B"=u8 0, "PING_C"=u8 0, "PING_D"=u8 0) -> (w3149:T7)
        n132 = Bundle By Name(cluster=w3130, "Yaw"=0.0) -> (w3129:T4)
        n133 = Bundle By Name(cluster=w3123, "S1"=w3119, "S2"=w3119, "S3"=w3119, "S4"=w3119) -> (w3122:T1)
      }
      frame "RESET ALL SENSORS" {
        w3152 = 0.0 ("SET TIME TO CHECK")
        # ">>> Line Sensor Cluster>>>"
        # ">>> IR Sensors >>>"
        # ">>> Time cluster >>>"
        # ">>> Object detection >>>"
        # ">>> Yaw >>>"
        # ">>> Ultrasonic Sensors Detect >>>"
        # ">>> Encoders >>>"
        # ">>> Stepper position >>>"
        # ">>> Line Sensor Cluster>>>"
        # ">>> IR Sensors >>>"
        # ">>> Time cluster >>>"
        # ">>> Object detection >>>"
        # ">>> Yaw >>>"
        # ">>> Ultrasonic Sensors Detect >>>"
        # ">>> Encoders >>>"
        # ">>> Stepper position >>>"
        # "Resets ALL SENSOR PARAMTERS"
        n134 = Wait (ms)(milliseconds to wait=u32 20) -> ()  [unwired: 1 out]
        n135 = Bundle By Name(cluster=w3162, "Time up flag"=FALSE, "SET TIME TO CHECK"=0.0) -> (w3161:T3)
        n136 = Bundle By Name(cluster=w3179, "Recognized Object"=FALSE, "Object X coordinate"=0.0, "Object Y coordinate"=0.0) -> (w3178:T9)
        n137 = Bundle By Name(cluster=w3169, "y Stepper Position"=u8 0, "z Stepper Position"=u8 0) -> (w3168:T5)
        n138 = Bundle By Name(cluster=w3157, "Line Detected?"=FALSE) -> (w3156:T1)
        n139 = Bundle By Name(cluster=w3154, "Left IR Sensor"=w3152, "Arm IR Sensor"=w3152) -> (w3153:T2)
        n140 = Bundle By Name(cluster=w3174, "xDistance"=0.0, "yDistance"=0.0, "wDistance"=0.0) -> (w3173:T6)
        n141 = Bundle By Name(cluster=w3186, "PING_A"=u8 0, "PING_B"=u8 0, "PING_C"=u8 0, "PING_D"=u8 0) -> (w3185:T7)
        n142 = Bundle By Name(cluster=w3165, "Yaw"=0.0) -> (w3164:T4)
      }
      frame "RESET YAW" {
        n143 = Wait (ms)(milliseconds to wait=u32 100) -> ()  [unwired: 1 out]
        n144 = call "navX reading VI.vi"("Mode"=navX_type_def."Zero Yaw") -> ()  [unwired: 2 in, 4 out]
      }
      frame "RESET ARM" {
        n145 = call "Arduino Interfacing VI.vi"("Data to Write"=I2C_MASTER_WRITE_NEW_Type_Def."Soft Reset", "AE Mode"=Arduino_Interfacing."Write to Arduino") -> ()  [unwired: 2 in, 2 out]
      }
      frame "--------CAM STATES-------" {
      }
      frame "OPEN IMAQ REF" {
        # ">>> Line Sensor Cluster>>>"
        # ">>State Logic  >>"
        # ">>> Time cluster >>>"
        # ">>> Object detection >>>"
        # ">>> Yaw >>>"
        # ">>> Ultrasonic Sensors Detect >>>"
        # ">>> Encoders >>>"
        # ">>> Stepper position >>>"
        # ">>> IR Sensors >>>"
        n146 = call "IMAQ Reference AE.vi"("IMAQ AE States"=IMAQ_Reference_AE."Initialize AE") -> ()  [unwired: 1 in, 2 out]
      }
      frame "OPEN LOG CAM" {
        n147 = call "Webcam AE.vi"("Session In"=T36 "cam0", "Camera states"=Webcam_AE."Initialize Camera") -> ("error out"=w3238:errorcluster, "Session Out"=w3237:T36)  [unwired: 1 in, 1 out]
        n148 = call "Webcam AE.vi"("error in (no error)"=w3238, "Session In"=w3237, "Camera states"=Webcam_AE."Open Camera") -> ()  [unwired: 3 out]
      }
      frame "OPEN LIFE CAM" {
        n149 = call "Webcam AE.vi"("Session In"=T36 "cam1", "Camera states"=Webcam_AE."Initialize Camera") -> ("error out"=w3253:errorcluster, "Session Out"=w3252:T36)  [unwired: 1 in, 1 out]
        n150 = call "Webcam AE.vi"("error in (no error)"=w3253, "Session In"=w3252, "Camera states"=Webcam_AE."Open Camera") -> ()  [unwired: 3 out]
      }
      frame "CAM ACQ" {
        # ">>State Logic  >>"
        # ">>> Time cluster >>>"
        # ">>> Yaw >>>"
        # ">>> Stepper position >>>"
        # ">>> Encoders >>>"
        # ">>> Object detection >>>"
        # ">>> Ultrasonic Sensors Detect >>>"
        n151 = call "Webcam AE.vi"("Camera states"=Webcam_AE."Continuous Acquisition") -> ()  [unwired: 2 in, 3 out]
      }
      frame "CAM CLOSE" {
        # ">>State Logic  >>"
        # ">>> Time cluster >>>"
        # ">>> Yaw >>>"
        # ">>> Stepper position >>>"
        # ">>> Encoders >>>"
        # ">>> Object detection >>>"
        # ">>> Ultrasonic Sensors Detect >>>"
        n152 = call "Webcam AE.vi"("Camera states"=Webcam_AE."Close Camera") -> ()  [unwired: 2 in, 3 out]
      }
      frame "PROCESS IMAGE" {
        # ">>> Line Sensor Cluster>>>"
        # ">>> IR Sensors >>>"
        # ">> Item Selection Bias >>"
        # ">> Item Selection Bias >>"
        # ">>State Logic  >>"
        # ">>> Time cluster >>>"
        # ">>> Yaw >>>"
        # ">>> Stepper position >>>"
        # ">>> Encoders >>>"
        # ">>> Object detection >>>"
        # ">>> Ultrasonic Sensors Detect >>>"
        n153 = call "Webcam AE.vi"("Camera states"=Webcam_AE."Retrieve Image") -> ("error out"=w3298:errorcluster, "Image Out"=w3299:T42)  [unwired: 2 in, 1 out]
        n154 = call "IMAQ Reference AE.vi"("IMAQ AE States"=IMAQ_Reference_AE."Get IMAQ Reference") -> ("Image Out"=w3288:T42)  [unwired: 1 in, 1 out]
        n155 = call "Object Detection SubVI.vi"("Error In"=w3298, "Mode"=w3285, "Image Dest"=w3288, "Image in"=w3299) -> ("Error out"=w3286:errorcluster, "Object Center Coordinates"=w3295:cluster{"x":sgl, "y":sgl}, "Object detection cluster"=w3291:T43)  [unwired: 1 out]
        n156 = Unbundle By Name(w3291) -> ("Object detected?"=w3292:bool)
        n157 = Unbundle By Name(w3295) -> ("x"=w3294:sgl, "y"=w3293:sgl)
        n158 = Bundle By Name(cluster=w3297, "Recognized Object"=w3292, "Object X coordinate"=w3294, "Object Y coordinate"=w3293) -> (w3296:T9)
      }
      frame "DISPOSE CAM BUFFERS" {
        # ">> Item Selection Bias >>"
        # ">>> Line Sensor Cluster>>>"
        # ">>> IR Sensors >>>"
        # ">>State Logic  >>"
        # ">>> Time cluster >>>"
        # ">>> Yaw >>>"
        # ">>> Stepper position >>>"
        # ">>> Encoders >>>"
        # ">>> Object detection >>>"
        # ">>> Ultrasonic Sensors Detect >>>"
        n159 = call "Webcam AE.vi"("Camera states"=Webcam_AE."Dispose Camera Image Buffer") -> ()  [unwired: 2 in, 3 out]
      }
      frame "DISPOSE PROC BUFFERS" {
        # ">>> Line Sensor Cluster>>>"
        # ">>State Logic  >>"
        # ">>> IR Sensors >>>"
        # ">>> Time cluster >>>"
        # ">>> Object detection >>>"
        # ">>> Yaw >>>"
        # ">>> Ultrasonic Sensors Detect >>>"
        # ">>> Encoders >>>"
        # ">>> Stepper position >>>"
        n160 = call "IMAQ Reference AE.vi"("IMAQ AE States"=IMAQ_Reference_AE."Dispose Processing Buffer") -> ()  [unwired: 1 in, 2 out]
      }
      frame "-----ARM ACTIONS-----" {
      }
      frame "CLOSE CLAW" {
        n161 = call "Arduino Interfacing VI.vi"("Data to Write"=I2C_MASTER_WRITE_NEW_Type_Def."Close Claw", "AE Mode"=Arduino_Interfacing."Write to Arduino") -> ()  [unwired: 2 in, 2 out]
      }
      frame "OPEN CLAW" {
        n162 = call "Arduino Interfacing VI.vi"("Data to Write"=I2C_MASTER_WRITE_NEW_Type_Def."Open Claw", "AE Mode"=Arduino_Interfacing."Write to Arduino") -> ()  [unwired: 2 in, 2 out]
      }
      frame "Z STEPPER CAM HEIGHT" {
        n163 = call "Arduino Interfacing VI.vi"("Data to Write"=I2C_MASTER_WRITE_NEW_Type_Def."zStepper 6k", "AE Mode"=Arduino_Interfacing."Write to Arduino") -> ()  [unwired: 2 in, 2 out]
      }
      frame "Z STEPPER GRAB HEIGHT" {
        # ">>State Logic  >>"
        # ">>> Time cluster >>>"
        # ">>> Yaw >>>"
        # ">>> Stepper position >>>"
        # ">>> Encoders >>>"
        # ">>> Object detection >>>"
        # ">>> Ultrasonic Sensors Detect >>>"
        n164 = call "Arduino Interfacing VI.vi"("Data to Write"=I2C_MASTER_WRITE_NEW_Type_Def."zStepper 100", "AE Mode"=Arduino_Interfacing."Write to Arduino") -> ()  [unwired: 2 in, 2 out]
      }
      frame "Z STEPPER BOX HEIGHT" {
        # ">>> IR Sensors >>>"
        # ">>> Time cluster >>>"
        # ">>> Yaw >>>"
        # ">>> Stepper position >>>"
        # ">>> Encoders >>>"
        # ">>> Object detection >>>"
        # ">>> Ultrasonic Sensors Detect >>>"
        n165 = call "Arduino Interfacing VI.vi"("Data to Write"=I2C_MASTER_WRITE_NEW_Type_Def."zStepper 4k", "AE Mode"=Arduino_Interfacing."Write to Arduino") -> ()  [unwired: 2 in, 2 out]
      }
      frame "Y STEPPER CONTROL" {
        # ">>State Logic  >>"
        # ">>> yStepper command>>>"
        # ">>> Time cluster >>>"
        # ">>> Yaw >>>"
        # ">>> Stepper position >>>"
        # ">>> Encoders >>>"
        # ">>> Object detection >>>"
        # ">>> Ultrasonic Sensors Detect >>>"
        n166 = Unbundle By Name(w3403) -> ("yStepper desired"=w3402:u8)
        n167 = call "Arduino Interfacing VI.vi"("y Stepper value"=w3402, "Data to Write"=I2C_MASTER_WRITE_NEW_Type_Def."yStepper control", "AE Mode"=Arduino_Interfacing."Write to Arduino") -> ()  [unwired: 1 in, 2 out]
      }
      frame "READ STEPPER VALUES" {
        # ">>State Logic  >>"
        # ">>> Time cluster >>>"
        # ">>> Yaw >>>"
        # ">>> Stepper position >>>"
        # ">>> Encoders >>>"
        # ">>> Object detection >>>"
        # ">>> Ultrasonic Sensors Detect >>>"
        n168 = call "Arduino Interfacing VI.vi"("AE Mode"=Arduino_Interfacing."Read From Arduino") -> ("Arduino Data"=w3420:T15)  [unwired: 3 in, 1 out]
        n169 = Unbundle By Name(w3420) -> ("y Stepper Position"=w3419:u8, "z Stepper Position"=w3418:u8)
        n170 = Bundle By Name(cluster=w3423, "y Stepper Position"=w3419, "z Stepper Position"=w3418) -> (w3422:T5)
      }
      frame " -----TIMING-----" {
        # ">>State Logic  >>"
        # ">>> Time cluster >>>"
        # ">>> Yaw >>>"
        # ">>> Stepper position >>>"
        # ">>> Encoders >>>"
        # ">>> Object detection >>>"
        # ">>> Ultrasonic Sensors Detect >>>"
      }
      frame "SET TIMER 1" {
        # ">>State Logic  >>"
        # ">>> Time cluster >>>"
        # ">>> Yaw >>>"
        # ">>> Stepper position >>>"
        # ">>> Encoders >>>"
        # ">>> Object detection >>>"
        # ">>> Ultrasonic Sensors Detect >>>"
        n171 = call "Elasped Timer.vi"("Time Setting"=1.0, "Action"=Elapsed_timer_control."Initialize") -> ()  [unwired: 6 in, 4 out]
        n172 = Bundle By Name(cluster=w3445, "Time up flag"=FALSE) -> (w3443:T3)
      }
      frame "SET TIMER 2" {
        # ">>State Logic  >>"
        # ">>> Time cluster >>>"
        # ">>> Yaw >>>"
        # ">>> Stepper position >>>"
        # ">>> Encoders >>>"
        # ">>> Object detection >>>"
        # ">>> Ultrasonic Sensors Detect >>>"
        n173 = call "Elasped Timer.vi"("Time Setting"=2.0, "Action"=Elapsed_timer_control."Initialize") -> ()  [unwired: 6 in, 4 out]
        n174 = Bundle By Name(cluster=w3459, "Time up flag"=FALSE) -> (w3457:T3)
      }
      frame "SET TIMER 3" {
        # ">>State Logic  >>"
        # ">>> Time cluster >>>"
        # ">>> Yaw >>>"
        # ">>> Stepper position >>>"
        # ">>> Encoders >>>"
        # ">>> Object detection >>>"
        # ">>> Ultrasonic Sensors Detect >>>"
        n175 = call "Elasped Timer.vi"("Time Setting"=3.0, "Action"=Elapsed_timer_control."Initialize") -> ()  [unwired: 6 in, 4 out]
        n176 = Bundle By Name(cluster=w3473, "Time up flag"=FALSE) -> (w3471:T3)
      }
      frame "SET TIMER 4" {
        # ">>State Logic  >>"
        # ">>> Time cluster >>>"
        # ">>> Yaw >>>"
        # ">>> Stepper position >>>"
        # ">>> Encoders >>>"
        # ">>> Object detection >>>"
        # ">>> Ultrasonic Sensors Detect >>>"
        n177 = call "Elasped Timer.vi"("Time Setting"=4.0, "Action"=Elapsed_timer_control."Initialize") -> ()  [unwired: 6 in, 4 out]
        n178 = Bundle By Name(cluster=w3487, "Time up flag"=FALSE) -> (w3485:T3)
      }
      frame "SET TIMER 5" {
        # ">>State Logic  >>"
        # ">>> Time cluster >>>"
        # ">>> Yaw >>>"
        # ">>> Stepper position >>>"
        # ">>> Encoders >>>"
        # ">>> Object detection >>>"
        # ">>> Ultrasonic Sensors Detect >>>"
        n179 = call "Elasped Timer.vi"("Time Setting"=5.0, "Action"=Elapsed_timer_control."Initialize") -> ()  [unwired: 6 in, 4 out]
        n180 = Bundle By Name(cluster=w3501, "Time up flag"=FALSE) -> (w3499:T3)
      }
      frame "START TIMER" {
        # ">>State Logic  >>"
        # ">>> Time cluster >>>"
        # ">>> Yaw >>>"
        # ">>> Stepper position >>>"
        # ">>> Encoders >>>"
        # ">>> Object detection >>>"
        # ">>> Ultrasonic Sensors Detect >>>"
        n181 = call "Elasped Timer.vi"("Action"=Elapsed_timer_control."Start") -> ("Time Out?!"=w3511:bool)  [unwired: 7 in, 3 out]
        n182 = Bundle By Name(cluster=w3514, "Time up flag"=w3511) -> (w3513:T3)
      }
    }
    "State Logic" <- w246
    "Image Processing Error" <- w213
    n183 = local read "TASK ENABLE"() -> (w240:bool)
    n184 = Not(x=w240) -> (.not. x?=w239:bool)
    n185 = case shown="True" w247 {
      tunnel: w251 -> [w278 w318]
      tunnel: w255 -> [w274 w320]
      tunnel: [w278 w318] -> w260
      tunnel: [w274 w321] -> w259
      tunnel: w256 -> [_ w316]
      tunnel: w258 -> [_ w317]
      tunnel: w253 -> [w277 w323]
      tunnel: [w277 w323] -> w252
      tunnel: "STOP TASK" -> [_ w306]
      tunnel: w246 -> [w276 w322]
      tunnel: [w276 w319] -> w245
      tunnel: w242 -> [w275 w312]
      tunnel: [w275 w312] -> w241
      tunnel: w239 -> [_ w307]
      tunnel: [w273 w304] -> w238
      tunnel: w237 -> [w273 w303]
      tunnel: w235 -> [w272 w300]
      tunnel: [w272 w300] -> w234
      tunnel: w232 -> [w271 w296]
      tunnel: [w271 w296] -> w231
      tunnel: w229 -> [w270 w294]
      tunnel: [w270 w294] -> w228
      tunnel: w226 -> [w269 w292]
      tunnel: [w269 w292] -> w225
      tunnel: w224 -> [w268 w291]
      tunnel: [w268 w290] -> w223
      tunnel: [_ w288] -> w222
      tunnel: w220 -> [w267 w286]
      tunnel: [w267 w286] -> w219
      tunnel: w218 -> [w266 w285]
      tunnel: [w266 w284] -> w217
      tunnel: w215 -> [w265 w281]
      tunnel: [w265 w281] -> w214
      tunnel: [w264 w280] -> w212
      tunnel: w210 -> [w264 w279]
      frame False {
        # ">> Item Selection Bias >>"
        # ">>State Logic Queue Reference >>"
        # ">>Action states Queue Reference >>"
        # ">>True Stop Next State >>"
        # ">>State Logic  >>"
        # ">>> IR Sensors >>>"
        # ">>> Line Sensor Cluster>>>"
        # ">>> Line Sensor Cluster>>>"
        # ">>> Motor control cluster >>>"
        # ">>> yStepper command>>>"
        # ">>> Motor control cluster >>>"
        # ">>> yStepper command>>>"
        # ">>> Motor control cluster >>>"
        # ">>> IR Sensors >>>"
        # ">>> IR Sensors >>>"
        # ">>> yStepper command>>>"
        # ">>> Time cluster >>>"
        # ">>> Yaw >>>"
        # ">>> Stepper position >>>"
        # ">>> Encoders >>>"
        # ">>> Object detection >>>"
        # ">>> Ultrasonic Sensors Detect >>>"
        # ">>> Time cluster >>>"
        # ">>> Yaw >>>"
        # ">>> Stepper position >>>"
        # ">>> Encoders >>>"
        # ">>> Object detection >>>"
        # ">>> Ultrasonic Sensors Detect >>>"
      }
      frame True {
        # ">> Item Selection Bias >>"
        # ">>> IR Sensors >>>"
        # ">>> Line Sensor Cluster>>>"
        # ">>> Line Sensor Cluster>>>"
        # ">>> Motor control cluster >>>"
        # ">>> yStepper command>>>"
        # ">>> IR Sensors >>>"
        # ">>> Motor control cluster >>>"
        # ">>State Logic Queue Reference >>"
        # ">>Timeout>>"
        # ">>> yStepper command>>>"
        # ">>> Time cluster >>>"
        # ">>> Object detection >>>"
        # ">>> Yaw >>>"
        # ">>> Ultrasonic Sensors Detect >>>"
        # ">>> Encoders >>>"
        # ">>> Stepper position >>>"
        # ">>State Logic  >>"
        # ">>True Stop Next State >>"
        # ">>Action Queue>>"
        # ">> Manual override >>"
        # ">>> Time cluster >>>"
        # ">>> Yaw >>>"
        # ">>> Stepper position >>>"
        # ">>> Encoders >>>"
        # ">>> Object detection >>>"
        # ">>> Ultrasonic Sensors Detect >>>"
        # ">>Action Queue>>"
        # ">>State Logic Queue Reference >>"
        n186 = Or(x=w306, y=w307) -> (x .or. y?=w305:bool)
        n187 = Unbundle By Name(w281) -> ("Line Detected?"=w282:bool)
        n188 = Unbundle By Name(w286) -> ("Left IR Sensor"=w287:dbl, "Arm IR Sensor"=w283:dbl)
        n189 = Unbundle By Name(w292) -> ("Time up flag"=w293:bool)
        n190 = Unbundle By Name(w294) -> ("Yaw"=w295:dbl, "Compass"=w289:dbl)
        n191 = Unbundle By Name(w296) -> ("y Stepper Position"=w298:u8, "z Stepper Position"=w297:u8)
        n192 = Unbundle By Name(w312) -> ("xDistance"=w309:dbl, "yDistance"=w310:dbl, "wDistance"=w311:dbl)
        n193 = Unbundle By Name(w300) -> ("Recognized Object"=w299:bool, "Object X coordinate"=w302:dbl, "Object Y coordinate"=w301:dbl)
        n194 = Unbundle By Name(w323) -> ("PING_A"=w315:u8, "PING_B"=w314:u8, "PING_C"=w313:u8, "PING_D"=w308:u8)
        n195 = case shown="19" w322 {
          tunnel: [w328 w340 w354 w365 w483 w500 w546 w583 w637 w680 w728 w772 w827 w875 w919 w979 w1020 w1063 w1112 w1155 w1208 w1246 w1298 w1342 w1386 w1416 w1434 w1480 w1521 w1570 w1623 w1662 w1711 w1754 w1807 w1845 w1897 w1933 w1982 w2025 w2078 w2122 w2167 w2219 w2260 w2308 w2347 w2389 w2444 w2498 w2536 w2582 w2631 w2672 w2716] -> w321
          tunnel: w320 -> [w328 w343 w355 w368 w485 w501 w547 w592 w635 w684 w729 w778 w820 w878 w926 w969 w1023 w1069 w1111 w1158 w1198 w1252 w1288 w1337 w1377 w1416 w1424 w1483 w1527 w1569 w1622 w1668 w1710 w1757 w1797 w1851 w1887 w1937 w1989 w2030 w2083 w2127 w2171 w2217 w2261 w2309 w2349 w2399 w2454 w2497 w2540 w2588 w2630 w2676 w2720]
          tunnel: [State_Type_Definitions,_for_0.26g_versions_and_later_2."Idle" ("Enum") State_Type_Definitions,_for_0.26g_versions_and_later_2."Idle" ("Enum") w350 w367 State_Type_Definitions,_for_0.26g_versions_and_later_2."Shutdown" ("Enum") w502 w548 w590 w638 w681 w727 w773 w826 w876 w921 w978 w1021 w1070 w1113 w1157 w1207 w1253 w1297 w1343 w1378 State_Type_Definitions,_for_0.26g_versions_and_later_2."Idle" ("Enum") w1433 w1481 w1528 w1571 w1624 w1669 w1712 w1756 w1806 w1852 w1896 w1934 w1983 w2026 w2079 w2123 w2168 w2220 w2259 w2307 w2348 w2394 w2455 w2499 w2537 w2583 w2632 w2673 w2717] -> w319
          tunnel: w318 -> [_ _ w353 w371 _ w506 w553 w586 w634 w685 w736 w777 w824 w879 w925 w976 w1018 w1068 w1109 w1159 w1205 w1251 w1295 w1340 w1385 _ w1431 w1478 w1526 w1567 w1620 w1667 w1708 w1758 w1804 w1850 w1894 w1941 w1988 w2033 w2086 w2130 w2174 w2216 w2262 w2302 w2350 w2398 w2453 w2496 w2544 w2587 w2629 w2680 w2721]
          tunnel: w317 -> [_ _ _ w370 _ w505 w552 w585 w633 w686 w735 w776 w823 w872 w924 w975 w1017 w1067 w1108 w1160 w1204 w1250 w1294 w1339 w1383 _ w1430 w1477 w1525 w1566 w1619 w1666 w1707 w1759 w1803 w1849 w1893 w1936 w1987 w2032 w2085 w2129 w2170 w2215 w2263 w2303 w2351 w2397 w2452 w2495 w2543 w2586 w2628 w2679 w2722]
          tunnel: w316 -> [_ _ w352 w366 _ w504 w551 w584 w632 w687 w734 w775 w822 w871 w923 w977 w1019 w1066 w1107 w1161 w1206 w1249 w1296 w1338 w1384 _ w1432 w1479 w1524 w1565 w1618 w1665 w1706 w1760 w1805 w1848 w1895 w1940 w1986 w2031 w2084 w2128 w2173 w2214 w2264 w2304 w2352 w2396 w2451 w2494 w2542 w2585 w2627 w2678 w2723]
          tunnel: w305 -> [_ _ _ _ _ w491 w545 w591 w631 w688 w731 w771 w825 w877 w927 w970 w1024 w1064 w1110 w1162 w1199 w1247 w1289 w1341 w1381 _ w1425 w1484 w1522 w1568 w1621 w1663 w1709 w1761 w1798 w1846 w1888 w1939 w1981 w2029 w2082 w2126 w2172 w2213 w2265 w2305 w2353 w2395 w2450 w2493 w2541 w2584 w2626 w2677 w2724]
          tunnel: w315 -> [_ _ _ _ _ _ _ _ _ _ _ _ _ _ _ _ _ _ _ _ _ _ _ _ _ _ _ _ _ _ _ _ _ _ _ _ _ _ _ _ _ _ _ _ _ _ _ _ _ _ _ _ _ _ _]
          tunnel: w314 -> [_ _ _ _ _ _ _ _ w630 _ _ _ w816 w860 w917 _ _ _ _ _ _ _ _ _ _ _ _ w1470 _ _ _ _ _ _ _ _ _ _ _ _ w2073 _ _ _ _ _ _ _ w2448 _ _ _ _ _ _]
          tunnel: w313 -> [_ _ _ _ _ _ _ _ w629 _ _ _ w817 w861 w918 _ _ _ _ _ _ _ _ _ _ _ _ w1471 _ _ _ _ _ _ _ _ _ _ _ _ w2072 _ _ _ _ _ _ _ w2449 _ _ _ _ _ _]
          tunnel: w311 -> [_ _ _ _ _ _ _ _ _ _ w733 _ _ _ _ _ _ _ _ _ _ _ _ _ _ _ _ _ _ _ _ _ _ _ _ _ _ _ _ _ _ _ _ _ _ _ _ w2392 _ _ _ _ _ _ _]
          tunnel: w310 -> [_ _ _ _ _ w499 w544 _ _ w679 _ _ _ _ w922 _ _ _ _ _ _ _ _ _ _ _ _ _ _ _ _ _ _ _ _ _ _ _ _ _ _ _ _ _ _ _ _ _ w2440 _ _ _ _ _ _]
          tunnel: w309 -> [_ _ _ _ _ _ _ _ _ _ _ _ _ w866 _ _ _ _ _ _ _ _ _ _ _ _ _ _ _ _ w1609 _ _ _ _ _ _ _ _ _ _ _ _ _ w2254 _ _ _ _ _ _ _ w2625 _ _]
          tunnel: w308 -> [_ _ _ _ _ _ _ _ _ _ _ _ _ _ _ _ _ _ _ _ _ _ _ _ _ _ _ _ _ _ _ _ _ _ _ _ _ _ _ _ _ _ _ _ _ _ _ _ _ _ _ _ _ _ _]
          tunnel: [State_Type_Definitions,_for_0.26g_versions_and_later_2."Idle" ("Enum") State_Type_Definitions,_for_0.26g_versions_and_later_2."Idle" ("Enum") State_Type_Definitions,_for_0.26g_versions_and_later_2."Idle" ("Enum") State_Type_Definitions,_for_0.26g_versions_and_later_2."Idle" ("Enum") State_Type_Definitions,_for_0.26g_versions_and_later_2."Shutdown" ("Enum") w497 w542 w589 w636 w682 w724 w770 w819 w874 w920 w980 w1022 w1062 w1114 w1156 w1209 w1245 w1299 w1344 w1379 w1418 w1435 w1482 w1520 w1572 w1625 w1661 w1713 w1755 w1808 w1844 w1898 w1935 w1984 w2028 w2081 w2125 w2169 w2218 w2258 w2306 w2346 w2393 w2456 w2500 w2538 w2581 w2633 w2674 w2718] -> w304
          tunnel: w303 -> [_ _ w350 _ _ _ _ _ _ _ _ _ _ _ _ _ _ _ _ _ _ _ _ _ _ w1418 _ _ _ _ _ _ _ _ _ _ _ _ _ _ _ _ _ _ _ _ _ _ _ _ _ _ _ _ _]
          tunnel: w299 -> [_ _ _ _ _ _ _ _ _ _ _ _ _ _ _ _ _ _ _ _ _ _ _ _ w1380 _ _ _ _ _ _ _ _ _ _ _ _ _ _ _ _ _ _ _ _ _ _ _ _ _ _ _ _ _ _]
          tunnel: w302 -> [_ _ _ _ _ _ _ _ _ _ _ _ _ _ _ _ _ _ _ _ _ _ _ _ _ _ _ _ _ _ w1615 _ _ _ _ _ _ _ _ _ _ _ _ _ _ _ _ _ _ _ _ _ _ _ _]
          tunnel: w301 -> [_ _ _ _ _ _ _ _ _ _ _ _ _ _ _ _ _ _ _ w1151 _ _ _ _ _ _ _ _ _ _ _ _ _ w1750 _ _ _ _ _ _ _ _ _ _ _ _ _ _ _ _ _ _ _ _ _]
          tunnel: w298 -> [_ _ _ _ _ _ _ _ _ _ _ _ _ _ _ _ _ _ _ w1150 _ _ _ _ _ _ _ _ _ _ _ _ _ w1749 _ _ _ _ _ _ _ _ _ _ _ _ _ _ _ _ _ _ _ _ _]
          tunnel: w297 -> [_ _ _ _ _ _ _ w588 _ _ _ w768 _ _ _ w973 _ w1058 _ _ w1202 _ w1292 w1336 _ _ w1428 _ _ _ _ _ _ _ w1801 _ w1891 w1938 _ _ _ _ _ _ _ _ _ _ _ _ _ _ _ _ _]
          tunnel: w295 -> [_ _ _ _ _ _ _ _ _ _ _ _ _ _ _ _ _ _ _ _ _ _ _ _ _ _ _ _ _ _ _ _ _ _ _ _ _ _ _ _ _ _ _ _ _ _ _ _ _ _ _ _ _ _ _]
          tunnel: w293 -> [_ _ _ _ _ _ _ _ _ _ _ _ _ _ _ _ w1012 _ w1104 _ _ w1243 _ _ _ _ _ _ w1518 w1562 _ w1659 w1703 _ _ w1842 _ _ _ _ _ _ w2163 _ _ w2301 w2345 _ _ _ w2539 w2580 _ w2675 w2719]
          tunnel: w291 -> [w326 w338 w349 w363 w481 w496 w541 w587 w628 w683 w723 w769 w818 w870 w916 w968 w1015 w1061 w1105 w1153 w1197 w1244 w1287 w1333 w1376 w1419 w1423 w1475 w1519 w1563 w1616 w1660 w1704 w1752 w1796 w1843 w1886 w1932 w1985 w2027 w2080 w2124 w2166 w2212 w2267 w2311 w2355 w2401 w2458 w2502 w2546 w2590 w2638 w2682 w2726]
          tunnel: [w326 w337 w349 w363 w481 w496 w541 w587 w628 w683 w723 w769 w818 w870 w916 w968 w1015 w1061 w1105 w1152 w1197 w1244 w1287 w1333 w1376 w1419 w1423 w1475 w1519 w1563 w1616 w1660 w1704 w1751 w1796 w1843 w1886 w1932 w1985 w2027 w2080 w2124 w2166 w2212 w2267 w2311 w2355 w2401 w2458 w2502 w2546 w2590 w2638 w2682 w2726] -> w290
          tunnel: w289 -> [_ _ _ _ _ _ _ _ _ _ _ _ _ _ _ _ _ _ _ _ _ _ _ _ _ _ _ _ _ _ _ _ _ _ _ _ _ _ w1980 _ _ _ _ _ _ _ _ _ _ _ _ _ _ _ _]
          tunnel: [_ _ _ TRUE _ _ _ _ _ _ _ _ _ _ _ _ _ _ _ _ _ _ _ _ _ _ _ _ _ _ _ _ _ _ _ _ _ _ _ _ _ _ _ _ _ _ _ _ _ _ _ _ _ _ _] -> w288
          tunnel: w287 -> [_ _ _ _ _ _ _ _ _ _ _ _ _ _ _ _ _ _ _ _ _ _ _ _ _ _ _ _ _ _ _ _ _ _ _ _ _ _ _ _ _ _ _ _ _ _ _ _ _ _ _ _ _ _ _]
          tunnel: w285 -> [w325 w335 w348 w361 w480 w495 w540 w582 w627 w676 w722 w765 w811 w859 w915 w967 w1014 w1060 w1103 w1147 w1196 w1242 w1286 w1332 w1375 w1420 w1422 w1468 w1517 w1561 w1612 w1658 w1702 w1746 w1795 w1841 w1885 w1931 w1976 w2024 w2077 w2121 w2165 w2211 w2269 w2313 w2357 w2403 w2460 w2504 w2548 w2592 w2640 w2684 w2728]
          tunnel: [w325 w334 w348 w361 w480 w495 w540 w582 w627 w676 w722 w765 w811 w859 w915 w967 w1014 w1060 w1103 w1147 w1196 w1242 w1286 w1332 w1375 w1420 w1422 w1468 w1517 w1561 w1611 w1658 w1702 w1746 w1795 w1841 w1885 w1931 w1976 w2024 w2077 w2121 w2165 w2211 w2269 w2313 w2357 w2403 w2460 w2504 w2548 w2592 w2640 w2684 w2728] -> w284
          tunnel: w283 -> [_ _ _ _ _ _ _ _ _ _ _ _ _ _ _ _ _ _ _ _ _ _ _ _ _ _ _ _ _ _ _ _ _ _ _ _ _ _ _ _ w2075 _ _ w2210 _ _ _ _ w2446 _ _ _ _ _ _]
          tunnel: w282 -> [_ _ _ _ _ w492 _ _ _ _ _ _ _ _ w913 _ _ _ _ _ _ _ _ _ _ _ _ _ _ _ _ _ _ _ _ _ _ _ _ w2023 _ w2119 _ _ w2256 _ _ _ _ w2492 _ _ w2624 _ _]
          tunnel: [w324 w330 w347 w360 w479 w494 w539 w581 w626 w675 w721 w764 w810 w858 w914 w966 w1013 w1059 w1102 w1146 w1195 w1241 w1285 w1331 w1374 w1415 w1421 w1467 w1516 w1560 w1604 w1657 w1701 w1745 w1794 w1840 w1884 w1930 w1975 w2022 w2074 w2120 w2164 w2207 w2268 w2312 w2356 w2402 w2459 w2503 w2547 w2591 w2639 w2683 w2727] -> w280
          tunnel: w279 -> [w324 w330 w347 _ w479 w494 w539 w581 w626 w675 w721 w764 w810 w858 w914 w966 w1013 w1059 w1102 w1146 w1195 w1241 w1285 w1331 w1374 w1415 w1421 w1467 w1516 w1560 w1604 w1657 w1701 w1745 w1794 w1840 w1884 w1930 w1975 w2022 w2074 w2120 w2164 w2207 w2268 w2312 w2356 w2402 w2459 w2503 w2547 w2591 w2639 w2683 w2727]
          frame 0 {
            # ">>> yStepper command>>>"
          }
          frame 1 {
            # ">>> yStepper command>>>"
            n196 = for {
              shift-right: [w346] -> w340
              shift-left: w343 -> [w345]
              tunnel: string[] ["INIT", "RESET ARM", "RESET FLAGS", "RESET YAW", "NAVX CALIBRATE"] -> [w344] mode=indexing
              n197 = Enqueue Element(queue=w345, element=w344) -> (queue out=w346:refnum<queue>)  [unwired: 2 in, 2 out]
            }
            n198 = Bundle By Name(cluster=w338, "yStepper desired"=u8 0) -> (w337:T18)
            n199 = Bundle By Name(cluster=w335, "ySpeed"=0.0, "xSpeed"=0.0, "wSpeed"=0.0) -> (w334:T17)
          }
          frame 3 {
            # ">>Action Queue>>"
            # ">>> Motor control cluster >>>"
            # ">>> yStepper command>>>"
            n200 = Flush Queue(queue=w353, error in (no error)=w352) -> ()  [unwired: 3 out]
            n201 = for {
              shift-right: [w359] -> w354
              shift-left: w355 -> [w358]
              tunnel: string[] ["STOP", "RESET ENCODERS", "RESET YAW", "RESET ARM", "RESET ALL SENSORS", "DISPOSE CAM BUFFERS", "DISPOSE PROC BUFFERS", "CAM CLOSE", ""] -> [w357] mode=indexing
              n202 = Enqueue Element(queue=w358, element=w357) -> (queue out=w359:refnum<queue>)  [unwired: 2 in, 2 out]
            }
          }
          frame 4, Default {
            # ">>> Motor control cluster >>>"
            # ">>> yStepper command>>>"
            n203 = Dequeue Element(queue=w371, timeout in ms (-1)=w370, error in (no error)=w366) -> (element=w369:T8)  [unwired: 3 out]
            n204 = case shown="\"Start Task 5\"" w369 {
              tunnel: [w374 w382 w390 w398 w406 w414 w422 w430 w438 w445 w455 w463 w470 w473] -> w365
              tunnel: w368 -> [w375 w383 w391 w399 w407 w415 w423 w431 w439 w446 w454 w462 w470 w474]
              tunnel: [State_Type_Definitions,_for_0.26g_versions_and_later_2."Task 1A" ("Enum") State_Type_Definitions,_for_0.26g_versions_and_later_2."Task 2:Raise Arm" ("Enum") State_Type_Definitions,_for_0.26g_versions_and_later_2."Task 3" ("Enum") State_Type_Definitions,_for_0.26g_versions_and_later_2."Task 4_A" ("Enum") State_Type_Definitions,_for_0.26g_versions_and_later_2."Task 5A" ("Enum") State_Type_Definitions,_for_0.26g_versions_and_later_2."Task 6_A" ("Enum") State_Type_Definitions,_for_0.26g_versions_and_later_2."Task 8A: RAISE ARM" ("Enum") State_Type_Definitions,_for_0.26g_versions_and_later_2."Task 8A: RAISE ARM" ("Enum") State_Type_Definitions,_for_0.26g_versions_and_later_2."Task 8A: RAISE ARM" ("Enum") State_Type_Definitions,_for_0.26g_versions_and_later_2."Task 8A: RAISE ARM" ("Enum") State_Type_Definitions,_for_0.26g_versions_and_later_2."Task 9A: Raise Arm" ("Enum") State_Type_Definitions."Task 9F: SCAN IMAGE" ("Enum") State_Type_Definitions,_for_0.26g_versions_and_later_2."Idle" ("Enum") State_Type_Definitions,_for_0.26g_versions_and_later_2."Shutdown" ("Enum")] -> w367
              tunnel: [enum16{"Ball", "Soap", "Gel", "Pipe", "None"}."None" ("Object recognition mode") enum16{"Ball", "Soap", "Gel", "Pipe", "None"}."None" ("Object recognition mode") enum16{"Ball", "Soap", "Gel", "Pipe", "None"}."None" ("Object recognition mode") enum16{"Ball", "Soap", "Gel", "Pipe", "None"}."None" ("Object recognition mode") enum16{"Ball", "Soap", "Gel", "Pipe", "None"}."None" ("Object recognition mode") enum16{"Ball", "Soap", "Gel", "Pipe", "None"}."None" ("Object recognition mode") enum16{"Ball", "Soap", "Gel", "Pipe", "None"}."Ball" ("Object recognition mode") enum16{"Ball", "Soap", "Gel", "Pipe", "None"}."Gel" ("Object recognition mode") enum16{"Ball", "Soap", "Gel", "Pipe", "None"}."Pipe" ("Object recognition mode") enum16{"Ball", "Soap", "Gel", "Pipe", "None"}."Soap" ("Object recognition mode") enum16{"Ball", "Soap", "Gel", "Pipe", "None"}."None" ("Object recognition mode") enum16{"Ball", "Soap", "Gel", "Pipe", "None"}."None" ("Object recognition mode") enum16{"Ball", "Soap", "Gel", "Pipe", "None"}."None" ("Object recognition mode") enum16{"Ball", "Soap", "Gel", "Pipe", "None"}."None" ("Object recognition mode")] -> w360
              frame "Start Task 1" {
                n205 = for {
                  shift-right: [w379] -> w374
                  shift-left: w375 -> [w378]
                  tunnel: string[] ["RESET ENCODERS", "RESET YAW", "FORWARD", "READ ENCODERS"] -> [w377] mode=indexing
                  n206 = Enqueue Element(queue=w378, element=w377) -> (queue out=w379:refnum<queue>)  [unwired: 2 in, 2 out]
                }
              }
              frame "Start Task 2" {
                n207 = for {
                  shift-right: [w387] -> w382
                  shift-left: w383 -> [w386]
                  tunnel: string[] ["RESET ENCODERS", "RESET YAW", "READ ULTRASONIC", "ARDUINO - ULTRASONIC"] -> [w385] mode=indexing
                  n208 = Enqueue Element(queue=w386, element=w385) -> (queue out=w387:refnum<queue>)  [unwired: 2 in, 2 out]
                }
              }
              frame "Start Task 3" {
                n209 = for {
                  shift-right: [w395] -> w390
                  shift-left: w391 -> [w394]
                  tunnel: string[] ["RESET ENCODERS", "READ ENCODERS", "R-ACW"] -> [w393] mode=indexing
                  n210 = Enqueue Element(queue=w394, element=w393) -> (queue out=w395:refnum<queue>)  [unwired: 2 in, 2 out]
                }
              }
              frame "Start Task 4" {
                n211 = for {
                  shift-right: [w403] -> w398
                  shift-left: w399 -> [w402]
                  tunnel: string[] ["RESET YAW", "RESET ENCODERS", "RESET ARM", "RESET FLAGS", "", ""] -> [w401] mode=indexing
                  n212 = Enqueue Element(queue=w402, element=w401) -> (queue out=w403:refnum<queue>)  [unwired: 2 in, 2 out]
                }
              }
              frame "Start Task 5" {
                n213 = for {
                  shift-right: [w411] -> w406
                  shift-left: w407 -> [w410]
                  tunnel: string[] ["RESET YAW", "RESET ENCODERS", "RESET ARM", "RESET ALL SENSORS", "", ""] -> [w409] mode=indexing
                  n214 = Enqueue Element(queue=w410, element=w409) -> (queue out=w411:refnum<queue>)  [unwired: 2 in, 2 out]
                }
              }
              frame "Start Task 6" {
                n215 = for {
                  shift-right: [w419] -> w414
                  shift-left: w415 -> [w418]
                  tunnel: string[] ["OPEN LOG CAM ", "", "", "", "", ""] -> [w417] mode=indexing
                  n216 = Enqueue Element(queue=w418, element=w417) -> (queue out=w419:refnum<queue>)  [unwired: 2 in, 2 out]
                }
              }
              frame "Start Task 8 - BALL" {
                n217 = for {
                  shift-right: [w427] -> w422
                  shift-left: w423 -> [w426]
                  tunnel: string[] ["RESET YAW", "RESET ENCODERS", "RESET ARM", "RESET FLAGS"] -> [w425] mode=indexing
                  n218 = Enqueue Element(queue=w426, element=w425) -> (queue out=w427:refnum<queue>)  [unwired: 2 in, 2 out]
                }
              }
              frame "Start Task 8 - Gel" {
                n219 = for {
                  shift-right: [w435] -> w430
                  shift-left: w431 -> [w434]
                  tunnel: string[] ["RESET YAW", "RESET ENCODERS", "RESET ARM", "RESET FLAGS"] -> [w433] mode=indexing
                  n220 = Enqueue Element(queue=w434, element=w433) -> (queue out=w435:refnum<queue>)  [unwired: 2 in, 2 out]
                }
              }
              frame "Start Task 8 - Pipe" {
                n221 = for {
                  shift-right: [w443] -> w438
                  shift-left: w439 -> [w442]
                  tunnel: string[] ["RESET YAW", "RESET ENCODERS", "RESET ARM", "RESET FLAGS"] -> [w441] mode=indexing
                  n222 = Enqueue Element(queue=w442, element=w441) -> (queue out=w443:refnum<queue>)  [unwired: 2 in, 2 out]
                }
              }
              frame "Start Task 8 - Soap" {
                n223 = for {
                  shift-right: [w451] -> w445
                  shift-left: w446 -> [w450]
                  tunnel: string[] ["RESET YAW", "RESET ENCODERS", "RESET ARM", "RESET FLAGS"] -> [w449] mode=indexing
                  n224 = Enqueue Element(queue=w450, element=w449) -> (queue out=w451:refnum<queue>)  [unwired: 2 in, 2 out]
                }
              }
              frame "Start Task 9" {
                n225 = for {
                  shift-right: [w459] -> w455
                  shift-left: w454 -> [w458]
                  tunnel: string[] ["RESET ENCODERS", "READ ENCODERS", "Z STEPPER BOX HEIGHT"] -> [w457] mode=indexing
                  n226 = Enqueue Element(queue=w458, element=w457) -> (queue out=w459:refnum<queue>)  [unwired: 2 in, 2 out]
                }
              }
              frame "Start Task A" {
                n227 = for {
                  shift-right: [w467] -> w463
                  shift-left: w462 -> [w466]
                  tunnel: string[] ["RESET ENCODERS", "READ ENCODERS", "RESET YAW", "Z STEPPER BOX HEIGHT"] -> [w465] mode=indexing
                  n228 = Enqueue Element(queue=w466, element=w465) -> (queue out=w467:refnum<queue>)  [unwired: 2 in, 2 out]
                }
              }
              frame "None", Default {
              }
              frame "Exit" {
                n229 = for {
                  shift-right: [w478] -> w473
                  shift-left: w474 -> [w477]
                  tunnel: string[] ["STOP", "RESET ENCODERS", "RESET YAW", "EXIT"] -> [w476] mode=indexing
                  n230 = Enqueue Element(queue=w477, element=w476) -> (queue out=w478:refnum<queue>)  [unwired: 2 in, 2 out]
                }
              }
            }
          }
          frame 5 {
            # ">> Item Selection Bias >>"
            # ">>> yStepper command>>>"
            n231 = for {
              shift-right: [w489] -> w483
              shift-left: w485 -> [w488]
              tunnel: string[] ["INIT", "RESET ENCODERS", "RESET FLAGS", "CAM CLOSE", "DISPOSE BUFFERS", "EXIT", ""] -> [w487] mode=indexing
              n232 = Enqueue Element(queue=w488, element=w487) -> (queue out=w489:refnum<queue>)  [unwired: 2 in, 2 out]
            }
          }
          frame 6 {
            # ">>> Motor control cluster >>>"
            # ">> Line detection >>"
            # ">> Checks if 1 metre moved >>"
            # ">>> yStepper command>>>"
            # "Use 250"
            n233 = Greater?(x=w499, y=265.0) -> (0:w493:bool)
            n234 = Dequeue Element(queue=w506, timeout in ms (-1)=w505, error in (no error)=w504) -> (element=w503:T8)  [unwired: 3 out]
            n235 = And(x=w492, y=w493) -> (x .and. y?=w490:bool)
            n236 = case shown="\"Start Task 1\", Default" w503 {
              tunnel: w491 -> [w507 _]
              tunnel: [w517 State_Type_Definitions,_for_0.26g_versions_and_later_2."True Stop" ("Enum")] -> w502
              tunnel: w501 -> [w515 w532]
              tunnel: [w514 w531] -> w500
              tunnel: [State_Type_Definitions,_for_0.26g_versions_and_later_2."Idle" ("Enum") State_Type_Definitions,_for_0.26g_versions_and_later_2."Shutdown" ("Enum")] -> w497
              tunnel: w490 -> [w508 _]
              frame "Start Task 1", Default {
                n237 = Or(x=w508, y=w507) -> (x .or. y?=w509:bool)
                n238 = case shown="True" w509 {
                  tunnel: w515 -> [w520 w526]
                  tunnel: [w519 w524] -> w514
                  frame False {
                    n239 = for {
                      shift-right: [w522] -> w519
                      shift-left: w520 -> [w523]
                      tunnel: string[] ["READ ENCODERS", "READ NAVX", "FORWARD", "READ LINE SENSOR"] ("element") -> [w521] mode=indexing
                      n240 = Enqueue Element(queue=w523, element=w521) -> (queue out=w522:refnum<queue>)  [unwired: 2 in, 2 out]
                    }
                  }
                  frame True {
                    n241 = for {
                      shift-right: [w528] -> w524
                      shift-left: w526 -> [w529]
                      tunnel: string[] ["RESET YAW", "RESET ENCODERS", "STOP", ""] -> [w527] mode=indexing
                      n242 = Enqueue Element(queue=w529, element=w527) -> (queue out=w528:refnum<queue>)  [unwired: 2 in, 2 out]
                    }
                  }
                }
                n243 = Select(t=State_Type_Definitions,_for_0.26g_versions_and_later_2."True Stop" ("Enum"), s=w507, f=State_Type_Definitions,_for_0.26g_versions_and_later_2."Task 1B" ("Enum")) -> (s? t:f=w512:T16)
                n244 = Select(t=w512, s=w508, f=State_Type_Definitions,_for_0.26g_versions_and_later_2."Task 1A" ("Enum")) -> (s? t:f=w517:T16)
              }
              frame "Exit" {
                n245 = for {
                  shift-right: [w536] -> w531
                  shift-left: w532 -> [w537]
                  tunnel: string[] ["STOP", "RESET ENCODERS", "RESET YAW", ""] -> [w535] mode=indexing
                  n246 = Enqueue Element(queue=w537, element=w535) -> (queue out=w536:refnum<queue>)  [unwired: 2 in, 2 out]
                }
              }
            }
          }
          frame 7 {
            # ">>> Motor control cluster >>>"
            # ">> Line detection >>"
            # ">> Adds small distance overhead after 1M >>"
            # ">>> yStepper command>>>"
            n247 = Greater?(x=w544, y=50.0) -> (0:w538:bool)
            n248 = Dequeue Element(queue=w553, timeout in ms (-1)=w552, error in (no error)=w551) -> (element=w550:T8)  [unwired: 3 out]
            n249 = Or(x=w538, y=w545) -> (x .or. y?=w549:bool)
            n250 = case shown="\"Start Task 1\", Default" w550 {
              tunnel: w549 -> [w556 _]
              tunnel: [w560 State_Type_Definitions,_for_0.26g_versions_and_later_2."True Stop" ("Enum")] -> w548
              tunnel: w547 -> [w557 w575]
              tunnel: [w555 w574] -> w546
              tunnel: [State_Type_Definitions,_for_0.26g_versions_and_later_2."Idle" ("Enum") State_Type_Definitions,_for_0.26g_versions_and_later_2."Shutdown" ("Enum")] -> w542
              frame "Start Task 1", Default {
                n251 = case shown="True" w556 {
                  tunnel: w557 -> [w563 w569]
                  tunnel: [w562 w567] -> w555
                  frame False {
                    n252 = for {
                      shift-right: [w565] -> w562
                      shift-left: w563 -> [w566]
                      tunnel: string[] ["READ ENCODERS", "READ NAVX", "FORWARD", "READ LINE SENSOR"] ("element") -> [w564] mode=indexing
                      n253 = Enqueue Element(queue=w566, element=w564) -> (queue out=w565:refnum<queue>)  [unwired: 2 in, 2 out]
                    }
                  }
                  frame True {
                    n254 = for {
                      shift-right: [w571] -> w567
                      shift-left: w569 -> [w572]
                      tunnel: string[] ["RESET YAW", "RESET ENCODERS", "STOP", ""] -> [w570] mode=indexing
                      n255 = Enqueue Element(queue=w572, element=w570) -> (queue out=w571:refnum<queue>)  [unwired: 2 in, 2 out]
                    }
                  }
                }
                n256 = Select(t=State_Type_Definitions,_for_0.26g_versions_and_later_2."True Stop" ("Enum"), s=w556, f=State_Type_Definitions,_for_0.26g_versions_and_later_2."Task 1B" ("Enum")) -> (s? t:f=w560:T16)
              }
              frame "Exit" {
                n257 = for {
                  shift-right: [w579] -> w574
                  shift-left: w575 -> [w580]
                  tunnel: string[] ["STOP", "RESET ENCODERS", "RESET YAW", ""] -> [w578] mode=indexing
                  n258 = Enqueue Element(queue=w580, element=w578) -> (queue out=w579:refnum<queue>)  [unwired: 2 in, 2 out]
                }
              }
            }
          }
          frame 8 {
            # ">> Stepper height reeached >>"
            # ">>> yStepper command>>>"
            # ">> Manual override >>"
            n259 = Dequeue Element(queue=w586, timeout in ms (-1)=w585, error in (no error)=w584) -> (element=w595:T8)  [unwired: 3 out]
            n260 = Equal?(x=w588, y=u8 60) -> (x = y?=w593:bool)
            n261 = case shown="\"Start Task 1\", Default" w595 {
              tunnel: [w606 State_Type_Definitions,_for_0.26g_versions_and_later_2."True Stop" ("Enum")] -> w590
              tunnel: [w604 w621] -> w583
              tunnel: w592 -> [w603 _]
              tunnel: w591 -> [w597 _]
              tunnel: [State_Type_Definitions,_for_0.26g_versions_and_later_2."Idle" ("Enum") State_Type_Definitions,_for_0.26g_versions_and_later_2."Shutdown" ("Enum")] -> w589
              tunnel: w593 -> [w596 _]
              frame "Start Task 1", Default {
                # ">> WIill proceed to part ii if not manual override >>"
                # ">>If ENABLE or Trigger is set to true>>"
                n262 = Or(x=w596, y=w597) -> (x .or. y?=w598:bool)
                n263 = case shown="True" w596 {
                  tunnel: [w609 w615] -> w604
                  tunnel: w603 -> [w608 w614]
                  frame False {
                    n264 = for {
                      shift-right: [w611] -> w609
                      shift-left: w608 -> [w612]
                      tunnel: string[] ["Z STEPPER CAM HEIGHT", "READ STEPPER VALUES"] ("element") -> [w610] mode=indexing
                      n265 = Enqueue Element(queue=w612, element=w610) -> (queue out=w611:refnum<queue>)  [unwired: 2 in, 2 out]
                    }
                  }
                  frame True {
                    n266 = for {
                      shift-right: [w617] -> w615
                      shift-left: w614 -> [w618]
                      tunnel: string[] ["ARDUINO - ULTRASONIC", "READ ULTRASONIC", "", "", "", ""] -> [w616] mode=indexing
                      n267 = Enqueue Element(queue=w618, element=w616) -> (queue out=w617:refnum<queue>)  [unwired: 2 in, 2 out]
                    }
                  }
                }
                n268 = Select(t=State_Type_Definitions,_for_0.26g_versions_and_later_2."True Stop" ("Enum"), s=w597, f=State_Type_Definitions,_for_0.26g_versions_and_later_2."Task 2:Sensor Mode" ("Enum")) -> (s? t:f=w600:T16)
                n269 = Select(t=w600, s=w598, f=State_Type_Definitions,_for_0.26g_versions_and_later_2."Task 2:Raise Arm" ("Enum")) -> (s? t:f=w606:T16)
              }
              frame "Exit" {
                n270 = for {
                  shift-right: [w624] -> w621
                  shift-left: _ -> [w625]
                  tunnel: string[] ["STOP", "RESET ENCODERS", "RESET YAW", ""] -> [w623] mode=indexing
                  n271 = Enqueue Element(queue=w625, element=w623) -> (queue out=w624:refnum<queue>)  [unwired: 2 in, 2 out]
                }
              }
            }
          }
          frame 9 {
            w642 = u8 20 ("y")
            # ">>> yStepper command>>>"
            # ">>Object detected>>"
            n272 = Dequeue Element(queue=w634, timeout in ms (-1)=w633, error in (no error)=w632) -> (element=w643:T8)  [unwired: 3 out]
            n273 = Less?(x=w630, y=w642) -> (x < y?=w641:bool)
            n274 = Less?(x=w629, y=w642) -> (x < y?=w640:bool)
            n275 = Or(x=w641, y=w640) -> (x .or. y?=w639:bool)
            "Obstacle detected" <- w639
            n276 = case shown="\"Start Task 1\", Default" w643 {
              tunnel: w639 -> [w646 _]
              tunnel: [w653 State_Type_Definitions,_for_0.26g_versions_and_later_2."True Stop" ("Enum")] -> w638
              tunnel: w631 -> [w645 _]
              tunnel: w635 -> [w652 w669]
              tunnel: [w651 w670] -> w637
              tunnel: [State_Type_Definitions,_for_0.26g_versions_and_later_2."Idle" ("Enum") State_Type_Definitions,_for_0.26g_versions_and_later_2."Shutdown" ("Enum")] -> w636
              frame "Start Task 1", Default {
                n277 = case shown="False" w646 {
                  tunnel: w652 -> [w656 w663]
                  tunnel: [w657 w662] -> w651
                  frame False {
                    n278 = for {
                      tunnel: string[] ["READ ULTRASONIC", "STOP"] ("element") -> [w658] mode=indexing
                      shift-right: [w660] -> w657
                      shift-left: w656 -> [w659]
                      n279 = Enqueue Element(queue=w659, element=w658) -> (queue out=w660:refnum<queue>)  [unwired: 2 in, 2 out]
                    }
                  }
                  frame True {
                    n280 = for {
                      shift-right: [w665] -> w662
                      shift-left: w663 -> [w666]
                      tunnel: string[] ["RESET ENCODERS", "READ NAVX", "READ ENCODERS"] -> [w664] mode=indexing
                      n281 = Enqueue Element(queue=w666, element=w664) -> (queue out=w665:refnum<queue>)  [unwired: 2 in, 2 out]
                    }
                  }
                }
                n282 = Or(x=w646, y=w645) -> (x .or. y?=w644:bool)
                n283 = Select(t=State_Type_Definitions,_for_0.26g_versions_and_later_2."True Stop" ("Enum"), s=w645, f=State_Type_Definitions,_for_0.26g_versions_and_later_2."Task 2:Reverse Mode" ("Enum")) -> (s? t:f=w647:T16)
                n284 = Select(t=w647, s=w644, f=State_Type_Definitions,_for_0.26g_versions_and_later_2."Task 2:Sensor Mode" ("Enum")) -> (s? t:f=w653:T16)
              }
              frame "Exit" {
                n285 = for {
                  shift-right: [w673] -> w670
                  shift-left: w669 -> [w674]
                  tunnel: string[] ["STOP", "RESET ENCODERS", "RESET YAW", "ARDUINO MODE 0"] -> [w672] mode=indexing
                  n286 = Enqueue Element(queue=w674, element=w672) -> (queue out=w673:refnum<queue>)  [unwired: 2 in, 2 out]
                }
              }
            }
          }
          frame 10 {
            # ">>> yStepper command>>>"
            n287 = Dequeue Element(queue=w685, timeout in ms (-1)=w686, error in (no error)=w687) -> (element=w689:T8)  [unwired: 3 out]
            n288 = Less?(x=w679, y=-50.0) -> (x < y?=w677:bool)
            n289 = case shown="\"Start Task 1\", Default" w689 {
              tunnel: [w699 State_Type_Definitions,_for_0.26g_versions_and_later_2."True Stop" ("Enum")] -> w681
              tunnel: w688 -> [w692 _]
              tunnel: w684 -> [w698 w715]
              tunnel: [w697 w716] -> w680
              tunnel: [State_Type_Definitions,_for_0.26g_versions_and_later_2."Idle" ("Enum") State_Type_Definitions,_for_0.26g_versions_and_later_2."Shutdown" ("Enum")] -> w682
              tunnel: w677 -> [w690 _]
              frame "Start Task 1", Default {
                n290 = case shown="True" w690 {
                  tunnel: w698 -> [w702 w709]
                  tunnel: [w703 w708] -> w697
                  frame False {
                    n291 = for {
                      tunnel: string[] ["READ ENCODERS", "REVERSE", "READ NAVX"] ("element") -> [w704] mode=indexing
                      shift-right: [w706] -> w703
                      shift-left: w702 -> [w705]
                      n292 = Enqueue Element(queue=w705, element=w704) -> (queue out=w706:refnum<queue>)  [unwired: 2 in, 2 out]
                    }
                  }
                  frame True {
                    n293 = for {
                      shift-right: [w711] -> w708
                      shift-left: w709 -> [w712]
                      tunnel: string[] ["STOP", "ARDUINO - ULTRASONIC", "READ ULTRASONIC", "RESET ENCODERS"] -> [w710] mode=indexing
                      n294 = Enqueue Element(queue=w712, element=w710) -> (queue out=w711:refnum<queue>)  [unwired: 2 in, 2 out]
                    }
                  }
                }
                n295 = Or(x=w690, y=w692) -> (x .or. y?=w691:bool)
                n296 = Select(t=State_Type_Definitions,_for_0.26g_versions_and_later_2."True Stop" ("Enum"), s=w692, f=State_Type_Definitions,_for_0.26g_versions_and_later_2."Task 2:Sensor Mode" ("Enum")) -> (s? t:f=w693:T16)
                n297 = Select(t=w693, s=w691, f=State_Type_Definitions,_for_0.26g_versions_and_later_2."Task 2:Reverse Mode" ("Enum")) -> (s? t:f=w699:T16)
              }
              frame "Exit" {
                n298 = for {
                  shift-right: [w719] -> w716
                  shift-left: w715 -> [w720]
                  tunnel: string[] ["STOP", "RESET ENCODERS", "RESET YAW", "ARDUINO MODE 0"] -> [w718] mode=indexing
                  n299 = Enqueue Element(queue=w720, element=w718) -> (queue out=w719:refnum<queue>)  [unwired: 2 in, 2 out]
                }
              }
            }
          }
          frame 11 {
            # ">>> Motor control cluster >>>"
            # ">>> yStepper command>>>"
            n300 = Dequeue Element(queue=w736, timeout in ms (-1)=w735, error in (no error)=w734) -> (element=w725:T8)  [unwired: 3 out]
            n301 = Less?(x=w733, y=-160.0) -> (x < y?=w730:bool)
            n302 = Or(x=w730, y=w731) -> (x .or. y?=w726:bool)
            n303 = case shown="\"Start Task 1\", Default" w725 {
              tunnel: w726 -> [w739 _]
              tunnel: [w743 State_Type_Definitions,_for_0.26g_versions_and_later_2."True Stop" ("Enum")] -> w727
              tunnel: w729 -> [w740 w759]
              tunnel: [w738 w758] -> w728
              tunnel: [State_Type_Definitions,_for_0.26g_versions_and_later_2."Idle" ("Enum") State_Type_Definitions,_for_0.26g_versions_and_later_2."Shutdown" ("Enum")] -> w724
              frame "Start Task 1", Default {
                n304 = case shown="False" w739 {
                  tunnel: w740 -> [w746 w752]
                  tunnel: [w745 w750] -> w738
                  frame False {
                    n305 = for {
                      shift-right: [w748] -> w745
                      shift-left: w746 -> [w749]
                      tunnel: string[] ["READ ENCODERS", "R-CW"] ("element") -> [w747] mode=indexing
                      n306 = Enqueue Element(queue=w749, element=w747) -> (queue out=w748:refnum<queue>)  [unwired: 2 in, 2 out]
                    }
                  }
                  frame True {
                    n307 = for {
                      shift-right: [w754] -> w750
                      shift-left: w752 -> [w755]
                      tunnel: string[] ["RESET YAW", "RESET ENCODERS", "STOP", "ARDUINO MODE 0"] -> [w753] mode=indexing
                      n308 = Enqueue Element(queue=w755, element=w753) -> (queue out=w754:refnum<queue>)  [unwired: 2 in, 2 out]
                    }
                  }
                }
                n309 = Select(t=State_Type_Definitions,_for_0.26g_versions_and_later_2."True Stop" ("Enum"), s=w739, f=State_Type_Definitions,_for_0.26g_versions_and_later_2."Task 3" ("Enum")) -> (s? t:f=w743:T16)
              }
              frame "Exit" {
                n310 = for {
                  shift-right: [w762] -> w758
                  shift-left: w759 -> [w763]
                  tunnel: string[] ["STOP", "RESET ENCODERS", "RESET YAW", ""] -> [w761] mode=indexing
                  n311 = Enqueue Element(queue=w763, element=w761) -> (queue out=w762:refnum<queue>)  [unwired: 2 in, 2 out]
                }
              }
            }
          }
          frame 12 {
            # ">> Stepper height reeached >>"
            # ">>> yStepper command>>>"
            # ">> Manual override >>"
            n312 = Dequeue Element(queue=w777, timeout in ms (-1)=w776, error in (no error)=w775) -> (element=w774:T8)  [unwired: 3 out]
            n313 = Equal?(x=w768, y=u8 60) -> (x = y?=w766:bool)
            n314 = case shown="\"Start Task 1\", Default" w774 {
              tunnel: [w789 State_Type_Definitions,_for_0.26g_versions_and_later_2."True Stop" ("Enum")] -> w773
              tunnel: [w787 w805] -> w772
              tunnel: w778 -> [w786 w802]
              tunnel: w771 -> [w780 _]
              tunnel: [State_Type_Definitions,_for_0.26g_versions_and_later_2."Idle" ("Enum") State_Type_Definitions,_for_0.26g_versions_and_later_2."Shutdown" ("Enum")] -> w770
              tunnel: w766 -> [w779 _]
              frame "Start Task 1", Default {
                # ">> WIill proceed to part ii if not manual override >>"
                # ">>If ENABLE or Trigger is set to true>>"
                n315 = Or(x=w779, y=w780) -> (x .or. y?=w781:bool)
                n316 = case shown="False" w779 {
                  tunnel: [w792 w798] -> w787
                  tunnel: w786 -> [w791 w797]
                  frame False {
                    n317 = for {
                      shift-right: [w794] -> w792
                      shift-left: w791 -> [w795]
                      tunnel: string[] ["Z STEPPER CAM HEIGHT", "READ STEPPER VALUES"] ("element") -> [w793] mode=indexing
                      n318 = Enqueue Element(queue=w795, element=w793) -> (queue out=w794:refnum<queue>)  [unwired: 2 in, 2 out]
                    }
                  }
                  frame True {
                    n319 = for {
                      shift-right: [w800] -> w798
                      shift-left: w797 -> [w801]
                      tunnel: string[] ["ARDUINO - ULTRASONIC", "READ ULTRASONIC", "FORWARD", "", "", ""] -> [w799] mode=indexing
                      n320 = Enqueue Element(queue=w801, element=w799) -> (queue out=w800:refnum<queue>)  [unwired: 2 in, 2 out]
                    }
                  }
                }
                n321 = Select(t=State_Type_Definitions,_for_0.26g_versions_and_later_2."True Stop" ("Enum"), s=w780, f=State_Type_Definitions,_for_0.26g_versions_and_later_2."Task 4_B" ("Enum")) -> (s? t:f=w783:T16)
                n322 = Select(t=w783, s=w781, f=State_Type_Definitions,_for_0.26g_versions_and_later_2."Task 4_A" ("Enum")) -> (s? t:f=w789:T16)
              }
              frame "Exit" {
                n323 = for {
                  shift-right: [w808] -> w805
                  shift-left: w802 -> [w809]
                  tunnel: string[] ["STOP", "RESET ENCODERS", "RESET YAW", ""] -> [w807] mode=indexing
                  n324 = Enqueue Element(queue=w809, element=w807) -> (queue out=w808:refnum<queue>)  [unwired: 2 in, 2 out]
                }
              }
            }
          }
          frame 13 {
            w815 = u8 20
            # ">> Path blocked >>"
            # ">>> yStepper command>>>"
            # ">> Manual override >>"
            n325 = Dequeue Element(queue=w824, timeout in ms (-1)=w823, error in (no error)=w822) -> (element=w821:T8)  [unwired: 3 out]
            n326 = Less?(x=w817, y=w815) -> (x < y?=w812:bool)
            n327 = Less?(x=w816, y=w815) -> (x < y?=w813:bool)
            n328 = And(x=w813, y=w812) -> (x .and. y?=w814:bool)
            n329 = case shown="\"Start Task 1\", Default" w821 {
              tunnel: [w838 State_Type_Definitions,_for_0.26g_versions_and_later_2."True Stop" ("Enum")] -> w826
              tunnel: [w836 w853] -> w827
              tunnel: w820 -> [w835 _]
              tunnel: w825 -> [w829 _]
              tunnel: [State_Type_Definitions,_for_0.26g_versions_and_later_2."Idle" ("Enum") State_Type_Definitions,_for_0.26g_versions_and_later_2."Shutdown" ("Enum")] -> w819
              tunnel: w814 -> [w828 _]
              frame "Start Task 1", Default {
                # ">> Manual override forces program to true stop >>"
                # ">>If ENABLE or Trigger is set to true>>"
                n330 = Or(x=w828, y=w829) -> (x .or. y?=w834:bool)
                n331 = case shown="False" w828 {
                  tunnel: [w841 w846] -> w836
                  tunnel: w835 -> [w840 w845]
                  frame False {
                    n332 = for {
                      shift-right: [w843] -> w841
                      shift-left: w840 -> [w844]
                      tunnel: string[] ["FORWARD", "READ ULTRASONIC", "READ NAVX"] ("element") -> [w842] mode=indexing
                      n333 = Enqueue Element(queue=w844, element=w842) -> (queue out=w843:refnum<queue>)  [unwired: 2 in, 2 out]
                    }
                  }
                  frame True {
                    n334 = for {
                      shift-right: [w849] -> w846
                      shift-left: w845 -> [w850]
                      tunnel: string[] ["STOP", "RESET YAW", "RESET ENCODERS", "RESET FLAGS"] -> [w848] mode=indexing
                      n335 = Enqueue Element(queue=w850, element=w848) -> (queue out=w849:refnum<queue>)  [unwired: 2 in, 2 out]
                    }
                  }
                }
                n336 = Select(t=State_Type_Definitions,_for_0.26g_versions_and_later_2."True Stop" ("Enum"), s=w829, f=State_Type_Definitions,_for_0.26g_versions_and_later_2."Task 4_C" ("Enum")) -> (s? t:f=w831:T16)
                n337 = Select(t=w831, s=w834, f=State_Type_Definitions,_for_0.26g_versions_and_later_2."Task 4_B" ("Enum")) -> (s? t:f=w838:T16)
              }
              frame "Exit" {
                n338 = for {
                  shift-right: [w856] -> w853
                  shift-left: _ -> [w857]
                  tunnel: string[] ["STOP", "RESET ENCODERS", "RESET YAW", ""] -> [w855] mode=indexing
                  n339 = Enqueue Element(queue=w857, element=w855) -> (queue out=w856:refnum<queue>)  [unwired: 2 in, 2 out]
                }
              }
            }
          }
          frame 14 {
            w869 = u8 20
            # ">> xDistance travelled>>"
            # ">> Path NOT blocked >>"
            # ">>> yStepper command>>>"
            # ">> Manual override >>"
            n340 = Dequeue Element(queue=w879, timeout in ms (-1)=w872, error in (no error)=w871) -> (element=w873:T8)  [unwired: 3 out]
            n341 = Greater?(x=w861, y=w869) -> (0:w867:bool)
            n342 = Greater?(x=w866, y=80.0) -> (0:w864:bool)
            n343 = Greater?(x=w860, y=w869) -> (0:w868:bool)
            n344 = And(x=w868, y=w867) -> (x .and. y?=w863:bool)
            n345 = And(x=w864, y=w863) -> (x .and. y?=w862:bool)
            n346 = case shown="\"Start Task 1\", Default" w873 {
              tunnel: [w890 State_Type_Definitions,_for_0.26g_versions_and_later_2."True Stop" ("Enum")] -> w876
              tunnel: [w888 w906] -> w875
              tunnel: w878 -> [w887 w903]
              tunnel: w877 -> [w881 _]
              tunnel: [State_Type_Definitions,_for_0.26g_versions_and_later_2."Idle" ("t") State_Type_Definitions,_for_0.26g_versions_and_later_2."Shutdown" ("Enum")] -> w874
              tunnel: w862 -> [w880 _]
              frame "Start Task 1", Default {
                # ">> Manual override forces program to true stop >>"
                # ">>If ENABLE or Trigger is set to true>>"
                n347 = Or(x=w880, y=w881) -> (x .or. y?=w886:bool)
                n348 = case shown="False" w880 {
                  tunnel: [w893 w898] -> w888
                  tunnel: w887 -> [w891 w897]
                  frame False {
                    n349 = for {
                      shift-right: [w895] -> w893
                      shift-left: w891 -> [w896]
                      tunnel: string[] ["RIGHT", "READ NAVX", "READ ENCODERS", "READ ULTRASONIC"] ("element") -> [w894] mode=indexing
                      n350 = Enqueue Element(queue=w896, element=w894) -> (queue out=w895:refnum<queue>)  [unwired: 2 in, 2 out]
                    }
                  }
                  frame True {
                    n351 = for {
                      shift-right: [w901] -> w898
                      shift-left: w897 -> [w902]
                      tunnel: string[] ["STOP", "RESET YAW", "RESET ENCODERS", "ARDUINO - ULTRASONIC"] -> [w900] mode=indexing
                      n352 = Enqueue Element(queue=w902, element=w900) -> (queue out=w901:refnum<queue>)  [unwired: 2 in, 2 out]
                    }
                  }
                }
                n353 = Select(t=State_Type_Definitions,_for_0.26g_versions_and_later_2."True Stop" ("Enum"), s=w881, f=State_Type_Definitions,_for_0.26g_versions_and_later_2."Task 4_D" ("Enum")) -> (s? t:f=w882:T16)
                n354 = Select(t=w882, s=w886, f=State_Type_Definitions,_for_0.26g_versions_and_later_2."Task 4_C" ("Enum")) -> (s? t:f=w890:T16)
              }
              frame "Exit" {
                n355 = for {
                  shift-right: [w909] -> w906
                  shift-left: w903 -> [w910]
                  tunnel: string[] ["STOP", "RESET ENCODERS", "RESET YAW", ""] -> [w908] mode=indexing
                  n356 = Enqueue Element(queue=w910, element=w908) -> (queue out=w909:refnum<queue>)  [unwired: 2 in, 2 out]
                }
              }
            }
          }
          frame 15 {
            w933 = u8 20
            # ">>> Motor control cluster >>>"
            # ">> Line detected >>"
            # ">> yDistance travelled>>"
            # ">> Path blocked >>"
            # ">>> yStepper command>>>"
            # ">> Manual override >>"
            n357 = Less?(x=w918, y=w933) -> (x < y?=w931:bool)
            n358 = Greater?(x=w922, y=200.0) -> (0:w929:bool)
            n359 = Less?(x=w917, y=w933) -> (x < y?=w932:bool)
            n360 = And(x=w932, y=w931) -> (x .and. y?=w928:bool)
            n361 = Dequeue Element(queue=w925, timeout in ms (-1)=w924, error in (no error)=w923) -> (element=w934:T8)  [unwired: 3 out]
            n362 = Or(x=w929, y=w928) -> (x .or. y?=w912:bool)
            n363 = And(x=w913, y=w912) -> (x .and. y?=w911:bool)
            n364 = case shown="\"Start Task 1\", Default" w934 {
              tunnel: [w945 State_Type_Definitions,_for_0.26g_versions_and_later_2."True Stop" ("Enum")] -> w921
              tunnel: [w943 w961] -> w919
              tunnel: w926 -> [w942 w958]
              tunnel: w927 -> [w936 _]
              tunnel: [State_Type_Definitions,_for_0.26g_versions_and_later_2."Idle" ("t") State_Type_Definitions,_for_0.26g_versions_and_later_2."Shutdown" ("Enum")] -> w920
              tunnel: w911 -> [w935 _]
              frame "Start Task 1", Default {
                # ">> Manual override forces program to true stop >>"
                # ">>If ENABLE or Trigger is set to true>>"
                n365 = Or(x=w935, y=w936) -> (x .or. y?=w941:bool)
                n366 = case shown="False" w935 {
                  tunnel: [w948 w953] -> w943
                  tunnel: w942 -> [w946 w952]
                  frame False {
                    n367 = for {
                      shift-right: [w950] -> w948
                      shift-left: w946 -> [w951]
                      tunnel: string[] ["FORWARD", "READ NAVX", "READ ENCODERS", "READ ULTRASONIC", "READ LINE SENSOR"] ("element") -> [w949] mode=indexing
                      n368 = Enqueue Element(queue=w951, element=w949) -> (queue out=w950:refnum<queue>)  [unwired: 2 in, 2 out]
                    }
                  }
                  frame True {
                    n369 = for {
                      shift-right: [w956] -> w953
                      shift-left: w952 -> [w957]
                      tunnel: string[] ["STOP", "RESET YAW", "RESET ENCODERS", "RESET FLAGS"] -> [w955] mode=indexing
                      n370 = Enqueue Element(queue=w957, element=w955) -> (queue out=w956:refnum<queue>)  [unwired: 2 in, 2 out]
                    }
                  }
                }
                n371 = Select(t=State_Type_Definitions,_for_0.26g_versions_and_later_2."True Stop" ("Enum"), s=w936, f=State_Type_Definitions,_for_0.26g_versions_and_later_2."True Stop" ("Enum")) -> (s? t:f=w937:T16)
                n372 = Select(t=w937, s=w941, f=State_Type_Definitions,_for_0.26g_versions_and_later_2."Task 4_D" ("Enum")) -> (s? t:f=w945:T16)
              }
              frame "Exit" {
                n373 = for {
                  shift-right: [w964] -> w961
                  shift-left: w958 -> [w965]
                  tunnel: string[] ["STOP", "RESET ENCODERS", "RESET YAW", ""] -> [w963] mode=indexing
                  n374 = Enqueue Element(queue=w965, element=w963) -> (queue out=w964:refnum<queue>)  [unwired: 2 in, 2 out]
                }
              }
            }
          }
          frame 16 {
            # "Stays in Task 5_A until stepper reaches desired \nheight"
            # ">>> Motor control cluster >>>"
            # ">>> yStepper command>>>"
            # ">> Manual override >>"
            n375 = Dequeue Element(queue=w976, timeout in ms (-1)=w975, error in (no error)=w977) -> (element=w974:T8)  [unwired: 3 out]
            n376 = Equal?(x=w973, y=u8 1) -> (x = y?=w971:bool)
            n377 = case shown="\"Start Task 1\", Default" w974 {
              tunnel: [w987 State_Type_Definitions,_for_0.26g_versions_and_later_2."True Stop" ("Enum")] -> w978
              tunnel: [w990 w1007] -> w979
              tunnel: [State_Type_Definitions,_for_0.26g_versions_and_later_2."Idle" ("Enum") State_Type_Definitions,_for_0.26g_versions_and_later_2."Shutdown" ("Enum")] -> w980
              tunnel: w971 -> [w986 _]
              tunnel: w970 -> [w985 _]
              tunnel: w969 -> [w981 w1004]
              frame "Start Task 1", Default {
                # "T: Go back to idle, F: Continue with task\""
                # ">> Manual override >>"
                n378 = case shown="True" w986 {
                  tunnel: [w994 w1000] -> w990
                  tunnel: w981 -> [w992 w998]
                  frame False {
                    n379 = for {
                      tunnel: string[] ["Z STEPPER GRAB HEIGHT", "READ STEPPER VALUES"] ("element") -> [w995] mode=indexing
                      shift-right: [w997] -> w994
                      shift-left: w992 -> [w996]
                      n380 = Enqueue Element(queue=w996, element=w995) -> (queue out=w997:refnum<queue>)  [unwired: 2 in, 2 out]
                    }
                  }
                  frame True {
                    n381 = for {
                      shift-right: [w1002] -> w1000
                      shift-left: w998 -> [w1003]
                      tunnel: string[] ["SET TIMER 2", "", ""] -> [w1001] mode=indexing
                      n382 = Enqueue Element(queue=w1003, element=w1001) -> (queue out=w1002:refnum<queue>)  [unwired: 2 in, 2 out]
                    }
                  }
                }
                n383 = Or(x=w986, y=w985) -> (x .or. y?=w988:bool)
                n384 = Select(t=State_Type_Definitions,_for_0.26g_versions_and_later_2."True Stop" ("Enum"), s=w985, f=State_Type_Definitions,_for_0.26g_versions_and_later_2."Task 5B" ("Enum")) -> (s? t:f=w982:T16)
                n385 = Select(t=w982, s=w988, f=State_Type_Definitions,_for_0.26g_versions_and_later_2."Task 5A" ("Enum")) -> (s? t:f=w987:T16)
              }
              frame "Exit" {
                n386 = for {
                  shift-right: [w1010] -> w1007
                  shift-left: w1004 -> [w1011]
                  tunnel: string[] ["STOP", "RESET ENCODERS", "RESET YAW", "ARDUINO MODE 0"] -> [w1009] mode=indexing
                  n387 = Enqueue Element(queue=w1011, element=w1009) -> (queue out=w1010:refnum<queue>)  [unwired: 2 in, 2 out]
                }
              }
            }
          }
          frame 17 {
            # ">>> yStepper command>>>"
            n388 = Dequeue Element(queue=w1018, timeout in ms (-1)=w1017, error in (no error)=w1019) -> (element=w1016:T8)  [unwired: 3 out]
            n389 = case shown="\"Start Task 1\", Default" w1016 {
              tunnel: [w1031 State_Type_Definitions,_for_0.26g_versions_and_later_2."True Stop" ("Enum")] -> w1021
              tunnel: [w1034 w1051] -> w1020
              tunnel: [State_Type_Definitions,_for_0.26g_versions_and_later_2."Idle" ("Enum") State_Type_Definitions,_for_0.26g_versions_and_later_2."Shutdown" ("Enum")] -> w1022
              tunnel: w1024 -> [w1030 _]
              tunnel: w1023 -> [w1026 w1048]
              tunnel: w1012 -> [w1025 _]
              frame "Start Task 1", Default {
                # "T: Go back to idle, F: Continue with task\""
                # ">> Manual override >>"
                n390 = case shown="True" w1025 {
                  tunnel: [w1038 w1044] -> w1034
                  tunnel: w1026 -> [w1036 w1042]
                  frame False {
                    n391 = for {
                      tunnel: string[] ["CLOSE CLAW", "START TIMER", ""] ("element") -> [w1039] mode=indexing
                      shift-right: [w1041] -> w1038
                      shift-left: w1036 -> [w1040]
                      n392 = Enqueue Element(queue=w1040, element=w1039) -> (queue out=w1041:refnum<queue>)  [unwired: 2 in, 2 out]
                    }
                  }
                  frame True {
                    n393 = for {
                      shift-right: [w1046] -> w1044
                      shift-left: w1042 -> [w1047]
                      tunnel: string[] ["STOP", "", "", ""] -> [w1045] mode=indexing
                      n394 = Enqueue Element(queue=w1047, element=w1045) -> (queue out=w1046:refnum<queue>)  [unwired: 2 in, 2 out]
                    }
                  }
                }
                n395 = Or(x=w1025, y=w1030) -> (x .or. y?=w1032:bool)
                n396 = Select(t=State_Type_Definitions,_for_0.26g_versions_and_later_2."True Stop" ("Enum"), s=w1030, f=State_Type_Definitions,_for_0.26g_versions_and_later_2."Task 5C" ("Enum")) -> (s? t:f=w1027:T16)
                n397 = Select(t=w1027, s=w1032, f=State_Type_Definitions,_for_0.26g_versions_and_later_2."Task 5B" ("Enum")) -> (s? t:f=w1031:T16)
              }
              frame "Exit" {
                n398 = for {
                  shift-right: [w1054] -> w1051
                  shift-left: w1048 -> [w1055]
                  tunnel: string[] ["STOP", "RESET ENCODERS", "RESET YAW", "ARDUINO MODE 0"] -> [w1053] mode=indexing
                  n399 = Enqueue Element(queue=w1055, element=w1053) -> (queue out=w1054:refnum<queue>)  [unwired: 2 in, 2 out]
                }
              }
            }
          }
          frame 18 {
            # ">>> Motor control cluster >>>"
            # ">>> yStepper command>>>"
            # ">> Manual override >>"
            n400 = Equal?(x=w1058, y=u8 60) -> (x = y?=w1056:bool)
            n401 = Dequeue Element(queue=w1068, timeout in ms (-1)=w1067, error in (no error)=w1066) -> (element=w1065:T8)  [unwired: 3 out]
            n402 = case shown="\"Start Task 1\", Default" w1065 {
              tunnel: [w1077 State_Type_Definitions,_for_0.26g_versions_and_later_2."True Stop" ("Enum")] -> w1070
              tunnel: [w1080 w1097] -> w1063
              tunnel: [State_Type_Definitions,_for_0.26g_versions_and_later_2."Idle" ("Enum") State_Type_Definitions,_for_0.26g_versions_and_later_2."Shutdown" ("Enum")] -> w1062
              tunnel: w1064 -> [w1071 _]
              tunnel: w1069 -> [w1076 w1094]
              tunnel: w1056 -> [w1075 _]
              frame "Start Task 1", Default {
                # ">> Is time up? >>"
                # "Determines if object is in range to pick up"
                # ">> Manual override >>"
                n403 = case shown="True" w1075 {
                  tunnel: [w1084 w1090] -> w1080
                  tunnel: w1076 -> [w1082 w1088]
                  frame False {
                    n404 = for {
                      tunnel: string[] ["Z STEPPER CAM HEIGHT", "READ STEPPER VALUES"] ("element") -> [w1085] mode=indexing
                      shift-right: [w1087] -> w1084
                      shift-left: w1082 -> [w1086]
                      n405 = Enqueue Element(queue=w1086, element=w1085) -> (queue out=w1087:refnum<queue>)  [unwired: 2 in, 2 out]
                    }
                  }
                  frame True {
                    n406 = for {
                      shift-right: [w1092] -> w1090
                      shift-left: w1088 -> [w1093]
                      tunnel: string[] ["SET TIMER 5", "", ""] -> [w1091] mode=indexing
                      n407 = Enqueue Element(queue=w1093, element=w1091) -> (queue out=w1092:refnum<queue>)  [unwired: 2 in, 2 out]
                    }
                  }
                }
                n408 = Or(x=w1075, y=w1071) -> (x .or. y?=w1078:bool)
                n409 = Select(t=State_Type_Definitions,_for_0.26g_versions_and_later_2."True Stop" ("Enum"), s=w1071, f=State_Type_Definitions,_for_0.26g_versions_and_later_2."Task 5D" ("Enum")) -> (s? t:f=w1073:T16)
                n410 = Select(t=w1073, s=w1078, f=State_Type_Definitions,_for_0.26g_versions_and_later_2."Task 5C" ("Enum")) -> (s? t:f=w1077:T16)
              }
              frame "Exit" {
                n411 = for {
                  shift-right: [w1100] -> w1097
                  shift-left: w1094 -> [w1101]
                  tunnel: string[] ["STOP", "RESET ENCODERS", "RESET YAW", "ARDUINO MODE 0"] -> [w1099] mode=indexing
                  n412 = Enqueue Element(queue=w1101, element=w1099) -> (queue out=w1100:refnum<queue>)  [unwired: 2 in, 2 out]
                }
              }
            }
          }
          frame 19 {
            # ">>> yStepper command>>>"
            n413 = Dequeue Element(queue=w1109, timeout in ms (-1)=w1108, error in (no error)=w1107) -> (element=w1106:T8)  [unwired: 3 out]
            n414 = case shown="\"Start Task 1\", Default" w1106 {
              tunnel: [w1121 State_Type_Definitions,_for_0.26g_versions_and_later_2."True Stop" ("Enum")] -> w1113
              tunnel: [w1124 w1141] -> w1112
              tunnel: [State_Type_Definitions,_for_0.26g_versions_and_later_2."Idle" ("Enum") State_Type_Definitions,_for_0.26g_versions_and_later_2."Shutdown" ("Enum")] -> w1114
              tunnel: w1110 -> [w1120 _]
              tunnel: w1111 -> [w1116 w1138]
              tunnel: w1104 -> [w1115 _]
              frame "Start Task 1", Default {
                # ">> T: Breaks out of state loop; F: Stays in loop>>"
                # ">> Manual override >>"
                # ">> Checks if time is up>>"
                # "Stays in Task 5D until the object is detected"
                # "T: Go back to idle, F: Continue with task\""
                # ">> Manual override >>"
                n415 = case shown="False" w1115 {
                  tunnel: [w1128 w1134] -> w1124
                  tunnel: w1116 -> [w1126 w1132]
                  frame False {
                    n416 = for {
                      tunnel: string[] ["START TIMER", "OPEN CLAW", ""] ("element") -> [w1129] mode=indexing
                      shift-right: [w1131] -> w1128
                      shift-left: w1126 -> [w1130]
                      n417 = Enqueue Element(queue=w1130, element=w1129) -> (queue out=w1131:refnum<queue>)  [unwired: 2 in, 2 out]
                    }
                  }
                  frame True {
                    n418 = for {
                      shift-right: [w1136] -> w1134
                      shift-left: w1132 -> [w1137]
                      tunnel: string[] ["CAM CLOSE", "", ""] -> [w1135] mode=indexing
                      n419 = Enqueue Element(queue=w1137, element=w1135) -> (queue out=w1136:refnum<queue>)  [unwired: 2 in, 2 out]
                    }
                  }
                }
                n420 = Or(x=w1115, y=w1120) -> (x .or. y?=w1122:bool)
                n421 = Select(t=State_Type_Definitions,_for_0.26g_versions_and_later_2."True Stop" ("Enum"), s=w1120, f=State_Type_Definitions,_for_0.26g_versions_and_later_2."True Stop" ("Enum")) -> (s? t:f=w1117:T16)
                n422 = Select(t=w1117, s=w1122, f=State_Type_Definitions,_for_0.26g_versions_and_later_2."Task 5D" ("Enum")) -> (s? t:f=w1121:T16)
              }
              frame "Exit" {
                n423 = for {
                  shift-right: [w1144] -> w1141
                  shift-left: w1138 -> [w1145]
                  tunnel: string[] ["STOP", "RESET ENCODERS", "RESET YAW", "ARDUINO MODE 0"] -> [w1143] mode=indexing
                  n424 = Enqueue Element(queue=w1145, element=w1143) -> (queue out=w1144:refnum<queue>)  [unwired: 2 in, 2 out]
                }
              }
            }
          }
          frame 20 {
            # ">>> yStepper command>>>"
            n425 = Dequeue Element(queue=w1159, timeout in ms (-1)=w1160, error in (no error)=w1161) -> (element=w1163:T8)  [unwired: 3 out]
            n426 = formula code="if (pos < 100)\ny = 41;\n\nelse if (pos >= 100 && pos <= 140)\ny = 30;\n\nelse if (pos >= 141 && pos <= 170)\ny = 25;\n\nelse if (pos >= 171 &&pos <= 180) \ny = 20;\n\nelse if (pos >= 181&& pos <= 200)\ny = 15;\n\nelse if (pos >= 201 && pos <= 230)\ny = 10;\n\nelse if (pos >= 231 && pos <= 320)\ny = 8;\n\nelse if (pos > 320)\ny = 0;"("pos"=w1151) -> ("y"=w1154:dbl)
            n427 = To Unsigned Byte Integer(number=w1154) -> (unsigned 8bit integer=w1149:u8)
            n428 = Equal?(x=w1150, y=w1149) -> (x = y?=w1148:bool)
            n429 = case shown="\"Start Task 1\", Default" w1163 {
              tunnel: [w1170 State_Type_Definitions,_for_0.26g_versions_and_later_2."True Stop" ("Enum")] -> w1157
              tunnel: [w1173 w1190] -> w1155
              tunnel: [State_Type_Definitions,_for_0.26g_versions_and_later_2."Idle" ("Enum") State_Type_Definitions,_for_0.26g_versions_and_later_2."Shutdown" ("Enum")] -> w1156
              tunnel: w1162 -> [w1169 _]
              tunnel: w1158 -> [w1165 w1187]
              tunnel: w1148 -> [w1164 _]
              frame "Start Task 1", Default {
                # ">> T: Breaks out of state loop; F: Stays in loop>>"
                # ">> Manual override >>"
                # ">> Checks if time is up>>"
                # "Stays in Task 5D until the object is detected"
                # "T: Go back to idle, F: Continue with task\""
                # ">> Manual override >>"
                n430 = case shown="False" w1164 {
                  tunnel: [w1177 w1183] -> w1173
                  tunnel: w1165 -> [w1175 w1181]
                  frame False {
                    n431 = for {
                      tunnel: string[] ["READ STEPPER VALUES", "Y STEPPER CONTROL", ""] ("element") -> [w1178] mode=indexing
                      shift-right: [w1180] -> w1177
                      shift-left: w1175 -> [w1179]
                      n432 = Enqueue Element(queue=w1179, element=w1178) -> (queue out=w1180:refnum<queue>)  [unwired: 2 in, 2 out]
                    }
                  }
                  frame True {
                    n433 = for {
                      shift-right: [w1185] -> w1183
                      shift-left: w1181 -> [w1186]
                      tunnel: string[] ["CAM CLOSE", "DISPOSE BUFFERS", ""] -> [w1184] mode=indexing
                      n434 = Enqueue Element(queue=w1186, element=w1184) -> (queue out=w1185:refnum<queue>)  [unwired: 2 in, 2 out]
                    }
                  }
                }
                n435 = Or(x=w1164, y=w1169) -> (x .or. y?=w1171:bool)
                n436 = Select(t=State_Type_Definitions,_for_0.26g_versions_and_later_2."True Stop" ("Enum"), s=w1169, f=State_Type_Definitions,_for_0.26g_versions_and_later_2."Task 5F: ARM GRAB HEIGHT" ("Enum")) -> (s? t:f=w1166:T16)
                n437 = Select(t=w1166, s=w1171, f=State_Type_Definitions,_for_0.26g_versions_and_later_2."Task 5E: POSITION ARM" ("Enum")) -> (s? t:f=w1170:T16)
              }
              frame "Exit" {
                n438 = for {
                  shift-right: [w1193] -> w1190
                  shift-left: w1187 -> [w1194]
                  tunnel: string[] ["STOP", "RESET ENCODERS", "RESET YAW", "ARDUINO MODE 0"] -> [w1192] mode=indexing
                  n439 = Enqueue Element(queue=w1194, element=w1192) -> (queue out=w1193:refnum<queue>)  [unwired: 2 in, 2 out]
                }
              }
            }
            n440 = Bundle By Name(cluster=w1153, "yStepper desired"=w1149) -> (w1152:T18)
          }
          frame 21 {
            # ">>> Motor control cluster >>>"
            # ">>> yStepper command>>>"
            # ">> Manual override >>"
            n441 = Dequeue Element(queue=w1205, timeout in ms (-1)=w1204, error in (no error)=w1206) -> (element=w1203:T8)  [unwired: 3 out]
            n442 = Equal?(x=w1202, y=u8 1) -> (x = y?=w1200:bool)
            n443 = case shown="\"Start Task 1\", Default" w1203 {
              tunnel: [w1216 State_Type_Definitions,_for_0.26g_versions_and_later_2."True Stop" ("Enum")] -> w1207
              tunnel: [w1219 w1236] -> w1208
              tunnel: [State_Type_Definitions,_for_0.26g_versions_and_later_2."Idle" ("Enum") State_Type_Definitions,_for_0.26g_versions_and_later_2."Shutdown" ("Enum")] -> w1209
              tunnel: w1200 -> [w1215 _]
              tunnel: w1199 -> [w1214 _]
              tunnel: w1198 -> [w1210 w1233]
              frame "Start Task 1", Default {
                # "Stays in Task 5F until stepper reaches desired \nheight"
                # "T: Go back to idle, F: Continue with task\""
                # ">> Manual override >>"
                n444 = case shown="True" w1215 {
                  tunnel: [w1223 w1229] -> w1219
                  tunnel: w1210 -> [w1221 w1227]
                  frame False {
                    n445 = for {
                      tunnel: string[] ["Z STEPPER GRAB HEIGHT", "READ STEPPER VALUES"] ("element") -> [w1224] mode=indexing
                      shift-right: [w1226] -> w1223
                      shift-left: w1221 -> [w1225]
                      n446 = Enqueue Element(queue=w1225, element=w1224) -> (queue out=w1226:refnum<queue>)  [unwired: 2 in, 2 out]
                    }
                  }
                  frame True {
                    n447 = for {
                      shift-right: [w1231] -> w1229
                      shift-left: w1227 -> [w1232]
                      tunnel: string[] ["SET TIMER 5", "CLOSE CLAW", ""] -> [w1230] mode=indexing
                      n448 = Enqueue Element(queue=w1232, element=w1230) -> (queue out=w1231:refnum<queue>)  [unwired: 2 in, 2 out]
                    }
                  }
                }
                n449 = Or(x=w1215, y=w1214) -> (x .or. y?=w1217:bool)
                n450 = Select(t=State_Type_Definitions,_for_0.26g_versions_and_later_2."True Stop" ("Enum"), s=w1214, f=State_Type_Definitions,_for_0.26g_versions_and_later_2."Task 5G: CLOSE CLAW" ("Enum")) -> (s? t:f=w1211:T16)
                n451 = Select(t=w1211, s=w1217, f=State_Type_Definitions,_for_0.26g_versions_and_later_2."Task 5F: ARM GRAB HEIGHT" ("Enum")) -> (s? t:f=w1216:T16)
              }
              frame "Exit" {
                n452 = for {
                  shift-right: [w1239] -> w1236
                  shift-left: w1233 -> [w1240]
                  tunnel: string[] ["STOP", "RESET ENCODERS", "RESET YAW", "ARDUINO MODE 0"] -> [w1238] mode=indexing
                  n453 = Enqueue Element(queue=w1240, element=w1238) -> (queue out=w1239:refnum<queue>)  [unwired: 2 in, 2 out]
                }
              }
            }
          }
          frame 22 {
            # ">>> yStepper command>>>"
            # ">> Manual override >>"
            n454 = Dequeue Element(queue=w1251, timeout in ms (-1)=w1250, error in (no error)=w1249) -> (element=w1248:T8)  [unwired: 3 out]
            n455 = case shown="\"Start Task 1\", Default" w1248 {
              tunnel: [w1260 State_Type_Definitions,_for_0.26g_versions_and_later_2."True Stop" ("Enum")] -> w1253
              tunnel: [w1263 w1280] -> w1246
              tunnel: [State_Type_Definitions,_for_0.26g_versions_and_later_2."Idle" ("Enum") State_Type_Definitions,_for_0.26g_versions_and_later_2."Shutdown" ("Enum")] -> w1245
              tunnel: w1247 -> [w1254 _]
              tunnel: w1252 -> [w1259 w1277]
              tunnel: w1243 -> [w1258 _]
              frame "Start Task 1", Default {
                # ">> Is time up? >>"
                # "Determines if object is in range to pick up"
                # ">> Manual override >>"
                n456 = case shown="True" w1258 {
                  tunnel: [w1267 w1273] -> w1263
                  tunnel: w1259 -> [w1265 w1271]
                  frame False {
                    n457 = for {
                      tunnel: string[] ["CLOSE CLAW", "START TIMER"] ("element") -> [w1268] mode=indexing
                      shift-right: [w1270] -> w1267
                      shift-left: w1265 -> [w1269]
                      n458 = Enqueue Element(queue=w1269, element=w1268) -> (queue out=w1270:refnum<queue>)  [unwired: 2 in, 2 out]
                    }
                  }
                  frame True {
                    n459 = for {
                      shift-right: [w1275] -> w1273
                      shift-left: w1271 -> [w1276]
                      tunnel: string[] ["READ STEPPER VALUES", "", ""] -> [w1274] mode=indexing
                      n460 = Enqueue Element(queue=w1276, element=w1274) -> (queue out=w1275:refnum<queue>)  [unwired: 2 in, 2 out]
                    }
                  }
                }
                n461 = Or(x=w1258, y=w1254) -> (x .or. y?=w1261:bool)
                n462 = Select(t=State_Type_Definitions,_for_0.26g_versions_and_later_2."True Stop" ("Enum"), s=w1254, f=State_Type_Definitions,_for_0.26g_versions_and_later_2."Task 5H: RAISE ARM" ("Enum")) -> (s? t:f=w1256:T16)
                n463 = Select(t=w1256, s=w1261, f=State_Type_Definitions,_for_0.26g_versions_and_later_2."Task 5G: CLOSE CLAW" ("Enum")) -> (s? t:f=w1260:T16)
              }
              frame "Exit" {
                n464 = for {
                  shift-right: [w1283] -> w1280
                  shift-left: w1277 -> [w1284]
                  tunnel: string[] ["STOP", "RESET ENCODERS", "RESET YAW", "ARDUINO MODE 0"] -> [w1282] mode=indexing
                  n465 = Enqueue Element(queue=w1284, element=w1282) -> (queue out=w1283:refnum<queue>)  [unwired: 2 in, 2 out]
                }
              }
            }
          }
          frame 23 {
            # ">>> yStepper command>>>"
            # ">> Manual override >>"
            n466 = Dequeue Element(queue=w1295, timeout in ms (-1)=w1294, error in (no error)=w1296) -> (element=w1293:T8)  [unwired: 3 out]
            n467 = Equal?(x=w1292, y=u8 60) -> (x = y?=w1290:bool)
            n468 = case shown="\"Start Task 1\", Default" w1293 {
              tunnel: [w1306 State_Type_Definitions,_for_0.26g_versions_and_later_2."True Stop" ("Enum")] -> w1297
              tunnel: [w1309 w1326] -> w1298
              tunnel: [State_Type_Definitions,_for_0.26g_versions_and_later_2."Idle" ("Enum") State_Type_Definitions,_for_0.26g_versions_and_later_2."Shutdown" ("Enum")] -> w1299
              tunnel: w1290 -> [w1305 _]
              tunnel: w1289 -> [w1304 _]
              tunnel: w1288 -> [w1300 w1323]
              frame "Start Task 1", Default {
                # "Stays in Task 5_A until stepper reaches desired \nheight"
                # "T: Go back to idle, F: Continue with task\""
                # ">> Manual override >>"
                n469 = case shown="False" w1305 {
                  tunnel: [w1313 w1319] -> w1309
                  tunnel: w1300 -> [w1311 w1317]
                  frame False {
                    n470 = for {
                      tunnel: string[] ["Z STEPPER CAM HEIGHT", "READ STEPPER VALUES"] ("element") -> [w1314] mode=indexing
                      shift-right: [w1316] -> w1313
                      shift-left: w1311 -> [w1315]
                      n471 = Enqueue Element(queue=w1315, element=w1314) -> (queue out=w1316:refnum<queue>)  [unwired: 2 in, 2 out]
                    }
                  }
                  frame True {
                    n472 = for {
                      shift-right: [w1321] -> w1319
                      shift-left: w1317 -> [w1322]
                      tunnel: string[] ["ARDUINO - ULTRASONIC", "READ ULTRASONIC", ""] -> [w1320] mode=indexing
                      n473 = Enqueue Element(queue=w1322, element=w1320) -> (queue out=w1321:refnum<queue>)  [unwired: 2 in, 2 out]
                    }
                  }
                }
                n474 = Or(x=w1305, y=w1304) -> (x .or. y?=w1307:bool)
                n475 = Select(t=State_Type_Definitions,_for_0.26g_versions_and_later_2."True Stop" ("Enum"), s=w1304, f=State_Type_Definitions,_for_0.26g_versions_and_later_2."True Stop" ("Enum")) -> (s? t:f=w1301:T16)
                n476 = Select(t=w1301, s=w1307, f=State_Type_Definitions,_for_0.26g_versions_and_later_2."Task 5H: RAISE ARM" ("Enum")) -> (s? t:f=w1306:T16)
              }
              frame "Exit" {
                n477 = for {
                  shift-right: [w1329] -> w1326
                  shift-left: w1323 -> [w1330]
                  tunnel: string[] ["STOP", "RESET ENCODERS", "RESET YAW", "ARDUINO MODE 0"] -> [w1328] mode=indexing
                  n478 = Enqueue Element(queue=w1330, element=w1328) -> (queue out=w1329:refnum<queue>)  [unwired: 2 in, 2 out]
                }
              }
            }
          }
          frame 24 {
            # ">>> yStepper command>>>"
            n479 = Dequeue Element(queue=w1340, timeout in ms (-1)=w1339, error in (no error)=w1338) -> (element=w1345:T8)  [unwired: 3 out]
            n480 = Equal?(x=w1336, y=u8 60) -> (x = y?=w1335:bool)
            n481 = case shown="\"Start Task 1\", Default" w1345 {
              tunnel: [w1352 State_Type_Definitions,_for_0.26g_versions_and_later_2."True Stop" ("Enum")] -> w1343
              tunnel: [w1351 w1369] -> w1342
              tunnel: [State_Type_Definitions,_for_0.26g_versions_and_later_2."Idle" ("Enum") State_Type_Definitions,_for_0.26g_versions_and_later_2."Shutdown" ("Enum")] -> w1344
              tunnel: w1341 -> [w1347 _]
              tunnel: w1337 -> [w1349 _]
              tunnel: w1335 -> [w1346 _]
              frame "Start Task 1", Default {
                n482 = case shown="False" w1346 {
                  tunnel: [w1357 w1363] -> w1351
                  tunnel: w1349 -> [w1355 w1361]
                  frame False {
                    n483 = for {
                      tunnel: string[] ["Z STEPPER CAM HEIGHT", "READ STEPPER VALUES"] ("element") -> [w1358] mode=indexing
                      shift-right: [w1360] -> w1357
                      shift-left: w1355 -> [w1359]
                      n484 = Enqueue Element(queue=w1359, element=w1358) -> (queue out=w1360:refnum<queue>)  [unwired: 2 in, 2 out]
                    }
                  }
                  frame True {
                    n485 = for {
                      shift-right: [w1365] -> w1363
                      shift-left: w1361 -> [w1366]
                      tunnel: string[] ["CAM ACQ", "OPEN LOG CAM"] -> [w1364] mode=indexing
                      n486 = Enqueue Element(queue=w1366, element=w1364) -> (queue out=w1365:refnum<queue>)  [unwired: 2 in, 2 out]
                    }
                  }
                }
                n487 = Or(x=w1346, y=w1347) -> (x .or. y?=w1348:bool)
                n488 = Select(t=State_Type_Definitions,_for_0.26g_versions_and_later_2."Task 6_B" ("Enum"), s=w1348, f=State_Type_Definitions,_for_0.26g_versions_and_later_2."Task 6_A" ("Enum")) -> (s? t:f=w1352:T16)
              }
              frame "Exit" {
                n489 = for {
                  shift-right: [w1372] -> w1369
                  shift-left: _ -> [w1373]
                  tunnel: string[] ["STOP", "RESET ENCODERS", "RESET YAW", "ARDUINO MODE 0"] -> [w1371] mode=indexing
                  n490 = Enqueue Element(queue=w1373, element=w1371) -> (queue out=w1372:refnum<queue>)  [unwired: 2 in, 2 out]
                }
              }
            }
          }
          frame 25 {
            # ">>> yStepper command>>>"
            n491 = Dequeue Element(queue=w1385, timeout in ms (-1)=w1383, error in (no error)=w1384) -> (element=w1382:T8)  [unwired: 3 out]
            n492 = case shown="\"Start Task 1\", Default" w1382 {
              tunnel: [w1392 State_Type_Definitions,_for_0.26g_versions_and_later_2."True Stop" ("Enum")] -> w1378
              tunnel: [w1391 w1410] -> w1386
              tunnel: [State_Type_Definitions,_for_0.26g_versions_and_later_2."Idle" ("Enum") State_Type_Definitions,_for_0.26g_versions_and_later_2."Shutdown" ("Enum")] -> w1379
              tunnel: w1381 -> [w1387 _]
              tunnel: w1380 -> [w1389 _]
              tunnel: w1377 -> [w1388 w1407]
              frame "Start Task 1", Default {
                # ">> Manual override >>"
                n493 = case shown="False" w1389 {
                  tunnel: [w1397 w1403] -> w1391
                  tunnel: w1388 -> [w1396 w1401]
                  frame False {
                    n494 = for {
                      shift-right: [w1400] -> w1397
                      shift-left: w1396 -> [w1399]
                      tunnel: string[] ["CAM ACQ", "PROCESS IMAGE", "OPEN CLAW"] -> [w1398] mode=indexing
                      n495 = Enqueue Element(queue=w1399, element=w1398) -> (queue out=w1400:refnum<queue>)  [unwired: 2 in, 2 out]
                    }
                  }
                  frame True {
                    n496 = for {
                      shift-right: [w1405] -> w1403
                      shift-left: w1401 -> [w1406]
                      tunnel: string[] ["CAM ACQ", "PROCESS IMAGE", "CLOSE CLAW"] -> [w1404] mode=indexing
                      n497 = Enqueue Element(queue=w1406, element=w1404) -> (queue out=w1405:refnum<queue>)  [unwired: 2 in, 2 out]
                    }
                  }
                }
                n498 = Select(t=State_Type_Definitions,_for_0.26g_versions_and_later_2."True Stop" ("Enum"), s=w1387, f=State_Type_Definitions,_for_0.26g_versions_and_later_2."Task 6_B" ("Enum")) -> (s? t:f=w1392:T16)
              }
              frame "Exit" {
                # ">> State after true stop >>"
                # ">> Goes to true stop >>"
                n499 = for {
                  shift-right: [w1413] -> w1410
                  shift-left: w1407 -> [w1414]
                  tunnel: string[] ["STOP", "RESET ENCODERS", "RESET YAW", ""] -> [w1412] mode=indexing
                  n500 = Enqueue Element(queue=w1414, element=w1412) -> (queue out=w1413:refnum<queue>)  [unwired: 2 in, 2 out]
                }
              }
            }
          }
          frame 26 {
          }
          frame 27 {
            # ">>> Motor control cluster >>>"
            # ">>> yStepper command>>>"
            # ">> Manual override >>"
            n501 = Dequeue Element(queue=w1431, timeout in ms (-1)=w1430, error in (no error)=w1432) -> (element=w1429:T8)  [unwired: 3 out]
            n502 = Equal?(x=w1428, y=u8 60) -> (x = y?=w1426:bool)
            n503 = case shown="\"Start Task 1\", Default" w1429 {
              tunnel: [w1442 State_Type_Definitions,_for_0.26g_versions_and_later_2."True Stop" ("Enum")] -> w1433
              tunnel: [w1445 w1462] -> w1434
              tunnel: [State_Type_Definitions,_for_0.26g_versions_and_later_2."Idle" ("Enum") State_Type_Definitions,_for_0.26g_versions_and_later_2."Shutdown" ("Enum")] -> w1435
              tunnel: w1426 -> [w1441 _]
              tunnel: w1425 -> [w1440 _]
              tunnel: w1424 -> [w1436 w1459]
              frame "Start Task 1", Default {
                # "Stays in Task 5_A until stepper reaches desired \nheight"
                # "T: Go back to idle, F: Continue with task\""
                # ">> Manual override >>"
                n504 = case shown="False" w1441 {
                  tunnel: [w1449 w1455] -> w1445
                  tunnel: w1436 -> [w1447 w1453]
                  frame False {
                    n505 = for {
                      tunnel: string[] ["Z STEPPER CAM HEIGHT", "READ STEPPER VALUES"] ("element") -> [w1450] mode=indexing
                      shift-right: [w1452] -> w1449
                      shift-left: w1447 -> [w1451]
                      n506 = Enqueue Element(queue=w1451, element=w1450) -> (queue out=w1452:refnum<queue>)  [unwired: 2 in, 2 out]
                    }
                  }
                  frame True {
                    n507 = for {
                      shift-right: [w1457] -> w1455
                      shift-left: w1453 -> [w1458]
                      tunnel: string[] ["ARDUINO - ULTRASONIC", "READ ULTRASONIC", ""] -> [w1456] mode=indexing
                      n508 = Enqueue Element(queue=w1458, element=w1456) -> (queue out=w1457:refnum<queue>)  [unwired: 2 in, 2 out]
                    }
                  }
                }
                n509 = Or(x=w1441, y=w1440) -> (x .or. y?=w1443:bool)
                n510 = Select(t=State_Type_Definitions,_for_0.26g_versions_and_later_2."True Stop" ("Enum"), s=w1440, f=State_Type_Definitions,_for_0.26g_versions_and_later_2."Task 8B: MOVE TO BOX" ("Enum")) -> (s? t:f=w1437:T16)
                n511 = Select(t=w1437, s=w1443, f=State_Type_Definitions,_for_0.26g_versions_and_later_2."Task 8A: RAISE ARM" ("Enum")) -> (s? t:f=w1442:T16)
              }
              frame "Exit" {
                n512 = for {
                  shift-right: [w1465] -> w1462
                  shift-left: w1459 -> [w1466]
                  tunnel: string[] ["STOP", "RESET ENCODERS", "RESET YAW", "ARDUINO MODE 0"] -> [w1464] mode=indexing
                  n513 = Enqueue Element(queue=w1466, element=w1464) -> (queue out=w1465:refnum<queue>)  [unwired: 2 in, 2 out]
                }
              }
            }
          }
          frame 28 {
            w1474 = u8 15 ("y")
            # ">>> yStepper command>>>"
            n514 = Less?(x=w1471, y=w1474) -> (x < y?=w1472:bool)
            n515 = Dequeue Element(queue=w1478, timeout in ms (-1)=w1477, error in (no error)=w1479) -> (element=w1476:T8)  [unwired: 3 out]
            n516 = Less?(x=w1470, y=w1474) -> (x < y?=w1473:bool)
            n517 = And(x=w1473, y=w1472) -> (x .and. y?=w1469:bool)
            n518 = case shown="\"Start Task 1\", Default" w1476 {
              tunnel: [w1491 State_Type_Definitions,_for_0.26g_versions_and_later_2."True Stop" ("Enum")] -> w1481
              tunnel: [w1494 w1511] -> w1480
              tunnel: [State_Type_Definitions,_for_0.26g_versions_and_later_2."Idle" ("Enum") State_Type_Definitions,_for_0.26g_versions_and_later_2."Shutdown" ("Enum")] -> w1482
              tunnel: w1484 -> [w1490 _]
              tunnel: w1483 -> [w1486 w1508]
              tunnel: w1469 -> [w1485 _]
              frame "Start Task 1", Default {
                # "Stays in Task 5_B to capture image over 5 seconds"
                # "T: Go back to idle, F: Continue with task\""
                # ">> Manual override >>"
                n519 = case shown="True" w1485 {
                  tunnel: [w1498 w1504] -> w1494
                  tunnel: w1486 -> [w1496 w1502]
                  frame False {
                    n520 = for {
                      tunnel: string[] ["FORWARD", "READ ULTRASONIC", "READ NAVX"] ("element") -> [w1499] mode=indexing
                      shift-right: [w1501] -> w1498
                      shift-left: w1496 -> [w1500]
                      n521 = Enqueue Element(queue=w1500, element=w1499) -> (queue out=w1501:refnum<queue>)  [unwired: 2 in, 2 out]
                    }
                  }
                  frame True {
                    n522 = for {
                      shift-right: [w1506] -> w1504
                      shift-left: w1502 -> [w1507]
                      tunnel: string[] ["STOP", "RESET ENCODERS", "OPEN LOG CAM", "SET TIMER 2", "OPEN IMAQ REF"] -> [w1505] mode=indexing
                      n523 = Enqueue Element(queue=w1507, element=w1505) -> (queue out=w1506:refnum<queue>)  [unwired: 2 in, 2 out]
                    }
                  }
                }
                n524 = Or(x=w1485, y=w1490) -> (x .or. y?=w1492:bool)
                n525 = Select(t=State_Type_Definitions,_for_0.26g_versions_and_later_2."True Stop" ("Enum"), s=w1490, f=State_Type_Definitions,_for_0.26g_versions_and_later_2."Task 8C: CAM BURST" ("Enum")) -> (s? t:f=w1487:T16)
                n526 = Select(t=w1487, s=w1492, f=State_Type_Definitions,_for_0.26g_versions_and_later_2."Task 8B: MOVE TO BOX" ("Enum")) -> (s? t:f=w1491:T16)
              }
              frame "Exit" {
                n527 = for {
                  shift-right: [w1514] -> w1511
                  shift-left: w1508 -> [w1515]
                  tunnel: string[] ["STOP", "RESET ENCODERS", "RESET YAW", "ARDUINO MODE 0"] -> [w1513] mode=indexing
                  n528 = Enqueue Element(queue=w1515, element=w1513) -> (queue out=w1514:refnum<queue>)  [unwired: 2 in, 2 out]
                }
              }
            }
          }
          frame 29 {
            # ">>> Motor control cluster >>>"
            # ">>> yStepper command>>>"
            # ">> Manual override >>"
            n529 = Dequeue Element(queue=w1526, timeout in ms (-1)=w1525, error in (no error)=w1524) -> (element=w1523:T8)  [unwired: 3 out]
            n530 = case shown="\"Start Task 1\", Default" w1523 {
              tunnel: [w1535 State_Type_Definitions,_for_0.26g_versions_and_later_2."True Stop" ("Enum")] -> w1528
              tunnel: [w1538 w1555] -> w1521
              tunnel: [State_Type_Definitions,_for_0.26g_versions_and_later_2."Idle" ("Enum") State_Type_Definitions,_for_0.26g_versions_and_later_2."Shutdown" ("Enum")] -> w1520
              tunnel: w1522 -> [w1529 _]
              tunnel: w1527 -> [w1534 w1552]
              tunnel: w1518 -> [w1533 _]
              frame "Start Task 1", Default {
                # ">> Is time up? >>"
                # "Determines if object is in range to pick up"
                # ">> Manual override >>"
                n531 = case shown="True" w1533 {
                  tunnel: [w1542 w1548] -> w1538
                  tunnel: w1534 -> [w1540 w1546]
                  frame False {
                    n532 = for {
                      tunnel: string[] ["CAM ACQ", "START TIMER"] ("element") -> [w1543] mode=indexing
                      shift-right: [w1545] -> w1542
                      shift-left: w1540 -> [w1544]
                      n533 = Enqueue Element(queue=w1544, element=w1543) -> (queue out=w1545:refnum<queue>)  [unwired: 2 in, 2 out]
                    }
                  }
                  frame True {
                    n534 = for {
                      shift-right: [w1550] -> w1548
                      shift-left: w1546 -> [w1551]
                      tunnel: string[] ["CAM CLOSE", "PROCESS IMAGE", "SET TIMER 5"] -> [w1549] mode=indexing
                      n535 = Enqueue Element(queue=w1551, element=w1549) -> (queue out=w1550:refnum<queue>)  [unwired: 2 in, 2 out]
                    }
                  }
                }
                n536 = Or(x=w1533, y=w1529) -> (x .or. y?=w1536:bool)
                n537 = Select(t=State_Type_Definitions,_for_0.26g_versions_and_later_2."True Stop" ("Enum"), s=w1529, f=State_Type_Definitions,_for_0.26g_versions_and_later_2."Task 8D: PROCESS IMAGE" ("Enum")) -> (s? t:f=w1531:T16)
                n538 = Select(t=w1531, s=w1536, f=State_Type_Definitions,_for_0.26g_versions_and_later_2."Task 8C: CAM BURST" ("Enum")) -> (s? t:f=w1535:T16)
              }
              frame "Exit" {
                n539 = for {
                  shift-right: [w1558] -> w1555
                  shift-left: w1552 -> [w1559]
                  tunnel: string[] ["STOP", "RESET ENCODERS", "RESET YAW", "ARDUINO MODE 0"] -> [w1557] mode=indexing
                  n540 = Enqueue Element(queue=w1559, element=w1557) -> (queue out=w1558:refnum<queue>)  [unwired: 2 in, 2 out]
                }
              }
            }
          }
          frame 30 {
            # ">>> yStepper command>>>"
            n541 = Dequeue Element(queue=w1567, timeout in ms (-1)=w1566, error in (no error)=w1565) -> (element=w1564:T8)  [unwired: 3 out]
            n542 = case shown="\"Start Task 1\", Default" w1564 {
              tunnel: [w1579 State_Type_Definitions,_for_0.26g_versions_and_later_2."True Stop" ("Enum")] -> w1571
              tunnel: [w1582 w1599] -> w1570
              tunnel: [State_Type_Definitions,_for_0.26g_versions_and_later_2."Idle" ("Enum") State_Type_Definitions,_for_0.26g_versions_and_later_2."Shutdown" ("Enum")] -> w1572
              tunnel: w1568 -> [w1578 _]
              tunnel: w1569 -> [w1574 w1596]
              tunnel: w1562 -> [w1573 _]
              frame "Start Task 1", Default {
                # ">> T: Breaks out of state loop; F: Stays in loop>>"
                # ">> Manual override >>"
                # ">> Checks if time is up>>"
                # "Stays in Task 5D until the object is detected"
                # "T: Go back to idle, F: Continue with task\""
                # ">> Manual override >>"
                n543 = case shown="True" w1573 {
                  tunnel: [w1586 w1592] -> w1582
                  tunnel: w1574 -> [w1584 w1590]
                  frame False {
                    n544 = for {
                      tunnel: string[] ["START TIMER", "PROCESS IMAGE", ""] ("element") -> [w1587] mode=indexing
                      shift-right: [w1589] -> w1586
                      shift-left: w1584 -> [w1588]
                      n545 = Enqueue Element(queue=w1588, element=w1587) -> (queue out=w1589:refnum<queue>)  [unwired: 2 in, 2 out]
                    }
                  }
                  frame True {
                    n546 = for {
                      shift-right: [w1594] -> w1592
                      shift-left: w1590 -> [w1595]
                      tunnel: string[] ["RESET ENCODERS", "", ""] -> [w1593] mode=indexing
                      n547 = Enqueue Element(queue=w1595, element=w1593) -> (queue out=w1594:refnum<queue>)  [unwired: 2 in, 2 out]
                    }
                  }
                }
                n548 = Or(x=w1573, y=w1578) -> (x .or. y?=w1580:bool)
                n549 = Select(t=State_Type_Definitions,_for_0.26g_versions_and_later_2."True Stop" ("Enum"), s=w1578, f=State_Type_Definitions,_for_0.26g_versions_and_later_2."Task 8E: ROBOT ADJUST" ("Enum")) -> (s? t:f=w1575:T16)
                n550 = Select(t=w1575, s=w1580, f=State_Type_Definitions,_for_0.26g_versions_and_later_2."Task 8D: PROCESS IMAGE" ("Enum")) -> (s? t:f=w1579:T16)
              }
              frame "Exit" {
                n551 = for {
                  shift-right: [w1602] -> w1599
                  shift-left: w1596 -> [w1603]
                  tunnel: string[] ["STOP", "RESET ENCODERS", "RESET YAW", "ARDUINO MODE 0"] -> [w1601] mode=indexing
                  n552 = Enqueue Element(queue=w1603, element=w1601) -> (queue out=w1602:refnum<queue>)  [unwired: 2 in, 2 out]
                }
              }
            }
          }
          frame 31 {
            # ">>> Motor control cluster >>>"
            # ">>> yStepper command>>>"
            n553 = Dequeue Element(queue=w1620, timeout in ms (-1)=w1619, error in (no error)=w1618) -> (element=w1617:T8)  [unwired: 3 out]
            n554 = Subtract(x=w1615, y=300.0) -> (x-y=w1613:dbl)
            "x-y" <- w1613
            n555 = formula code="if (error <= -61&&error > -300){\ndistance = -15;\nxSpeed = -30;\n}\n\nelse if (error <= -51 && error >= -60){\ndistance = -10;\nxSpeed = -30;\n}\n\nelse if (error >= -50 && error <= 50){\ndistance = 0;\nxSpeed = 0;\n}\n\nelse if (error >= 51 && error <= 80){\ndistance = 10;\nxSpeed = 30;\n}\n\nelse if (error >= 81 && error <= 100){\ndistance = 15;\nxSpeed = 30;\n}\n\nelse if (error >= 101 && error <= 120){\ndistance = 20;\nxSpeed = 30;\n}\n\nelse if (error >= 121 && error < 300){\ndistance = 25;\nxSpeed = 30;\n}\n\nelse{\ndistance = 0;\nxSpeed = 0;\n}"("error"=w1613) -> ("distance"=w1608:dbl, "xSpeed"=w1610:dbl)
            n556 = formula code="if (target > 0){\nif (current  >= target)\noutput = 1;\n\nelse if (current != target)\noutput = 0;\n}\n\nelse if (target == 0){\nif (current == target)\noutput = 1;\n\nelse if (current != target)\noutput = 0;\n}\n\nelse if (target < 0){\nif (current <= target)\noutput = 1;\n\nelse if (current != target)\noutput = 0;\n}\n\nelse if (current != target)\noutput = 0;"("target"=w1608, "current"=w1609) -> ("output"=w1607:dbl)
            n557 = Bundle By Name(cluster=w1612, "xSpeed"=w1610) -> (w1611:T17)
            n558 = Equal?(x=w1607, y=1.0) -> (x = y?=w1605:bool)
            n559 = case shown="\"Start Task 1\", Default" w1617 {
              tunnel: [w1632 State_Type_Definitions,_for_0.26g_versions_and_later_2."True Stop" ("Enum")] -> w1624
              tunnel: [w1635 w1652] -> w1623
              tunnel: [State_Type_Definitions,_for_0.26g_versions_and_later_2."Idle" ("Enum") State_Type_Definitions,_for_0.26g_versions_and_later_2."Shutdown" ("Enum")] -> w1625
              tunnel: w1621 -> [w1631 _]
              tunnel: w1622 -> [w1627 w1649]
              tunnel: w1605 -> [w1626 _]
              frame "Start Task 1", Default {
                # ">> T: Breaks out of state loop; F: Stays in loop>>"
                # ">> Manual override >>"
                # ">> Checks if time is up>>"
                # "Stays in Task 5D until the object is detected"
                # "T: Go back to idle, F: Continue with task\""
                # ">> Manual override >>"
                n560 = case shown="True" w1626 {
                  tunnel: [w1639 w1645] -> w1635
                  tunnel: w1627 -> [w1637 w1643]
                  frame False {
                    n561 = for {
                      tunnel: string[] ["X AXIS - SLOW", "READ ENCODERS", "READ NAVX"] ("element") -> [w1640] mode=indexing
                      shift-right: [w1642] -> w1639
                      shift-left: w1637 -> [w1641]
                      n562 = Enqueue Element(queue=w1641, element=w1640) -> (queue out=w1642:refnum<queue>)  [unwired: 2 in, 2 out]
                    }
                  }
                  frame True {
                    n563 = for {
                      shift-right: [w1647] -> w1645
                      shift-left: w1643 -> [w1648]
                      tunnel: string[] ["SET TIMER 2", "STOP", "READ STEPPER VALUES", ""] -> [w1646] mode=indexing
                      n564 = Enqueue Element(queue=w1648, element=w1646) -> (queue out=w1647:refnum<queue>)  [unwired: 2 in, 2 out]
                    }
                  }
                }
                n565 = Or(x=w1626, y=w1631) -> (x .or. y?=w1633:bool)
                n566 = Select(t=State_Type_Definitions,_for_0.26g_versions_and_later_2."True Stop" ("Enum"), s=w1631, f=State_Type_Definitions,_for_0.26g_versions_and_later_2."Task 8H: ARM ADJUST" ("Enum")) -> (s? t:f=w1628:T16)
                n567 = Select(t=w1628, s=w1633, f=State_Type_Definitions,_for_0.26g_versions_and_later_2."Task 8E: ROBOT ADJUST" ("Enum")) -> (s? t:f=w1632:T16)
              }
              frame "Exit" {
                n568 = for {
                  shift-right: [w1655] -> w1652
                  shift-left: w1649 -> [w1656]
                  tunnel: string[] ["STOP", "RESET ENCODERS", "RESET YAW", "ARDUINO MODE 0"] -> [w1654] mode=indexing
                  n569 = Enqueue Element(queue=w1656, element=w1654) -> (queue out=w1655:refnum<queue>)  [unwired: 2 in, 2 out]
                }
              }
            }
          }
          frame 32 {
            # ">>> Motor control cluster >>>"
            # ">>> yStepper command>>>"
            # ">> Manual override >>"
            n570 = Dequeue Element(queue=w1667, timeout in ms (-1)=w1666, error in (no error)=w1665) -> (element=w1664:T8)  [unwired: 3 out]
            n571 = case shown="\"Start Task 1\", Default" w1664 {
              tunnel: [w1676 State_Type_Definitions,_for_0.26g_versions_and_later_2."True Stop" ("Enum")] -> w1669
              tunnel: [w1679 w1696] -> w1662
              tunnel: [State_Type_Definitions,_for_0.26g_versions_and_later_2."Idle" ("Enum") State_Type_Definitions,_for_0.26g_versions_and_later_2."Shutdown" ("Enum")] -> w1661
              tunnel: w1663 -> [w1670 _]
              tunnel: w1668 -> [w1675 w1693]
              tunnel: w1659 -> [w1674 _]
              frame "Start Task 1", Default {
                # ">> Is time up? >>"
                # "Determines if object is in range to pick up"
                # ">> Manual override >>"
                n572 = case shown="False" w1674 {
                  tunnel: [w1683 w1689] -> w1679
                  tunnel: w1675 -> [w1681 w1687]
                  frame False {
                    n573 = for {
                      tunnel: string[] ["CAM ACQ", "START TIMER"] ("element") -> [w1684] mode=indexing
                      shift-right: [w1686] -> w1683
                      shift-left: w1681 -> [w1685]
                      n574 = Enqueue Element(queue=w1685, element=w1684) -> (queue out=w1686:refnum<queue>)  [unwired: 2 in, 2 out]
                    }
                  }
                  frame True {
                    n575 = for {
                      shift-right: [w1691] -> w1689
                      shift-left: w1687 -> [w1692]
                      tunnel: string[] ["CAM CLOSE", "PROCESS IMAGE", "SET TIMER 3"] -> [w1690] mode=indexing
                      n576 = Enqueue Element(queue=w1692, element=w1690) -> (queue out=w1691:refnum<queue>)  [unwired: 2 in, 2 out]
                    }
                  }
                }
                n577 = Or(x=w1674, y=w1670) -> (x .or. y?=w1677:bool)
                n578 = Select(t=State_Type_Definitions,_for_0.26g_versions_and_later_2."True Stop" ("Enum"), s=w1670, f=State_Type_Definitions,_for_0.26g_versions_and_later_2."Task 8G: PROCESS IMAGE 2" ("Enum")) -> (s? t:f=w1672:T16)
                n579 = Select(t=w1672, s=w1677, f=State_Type_Definitions,_for_0.26g_versions_and_later_2."Task 8F: CAM BURST 2" ("Enum")) -> (s? t:f=w1676:T16)
              }
              frame "Exit" {
                n580 = for {
                  shift-right: [w1699] -> w1696
                  shift-left: w1693 -> [w1700]
                  tunnel: string[] ["STOP", "RESET ENCODERS", "RESET YAW", "ARDUINO MODE 0"] -> [w1698] mode=indexing
                  n581 = Enqueue Element(queue=w1700, element=w1698) -> (queue out=w1699:refnum<queue>)  [unwired: 2 in, 2 out]
                }
              }
            }
          }
          frame 33 {
            # ">>> yStepper command>>>"
            n582 = Dequeue Element(queue=w1708, timeout in ms (-1)=w1707, error in (no error)=w1706) -> (element=w1705:T8)  [unwired: 3 out]
            n583 = case shown="\"Start Task 1\", Default" w1705 {
              tunnel: [w1720 State_Type_Definitions,_for_0.26g_versions_and_later_2."True Stop" ("Enum")] -> w1712
              tunnel: [w1723 w1740] -> w1711
              tunnel: [State_Type_Definitions,_for_0.26g_versions_and_later_2."Idle" ("Enum") State_Type_Definitions,_for_0.26g_versions_and_later_2."Shutdown" ("Enum")] -> w1713
              tunnel: w1709 -> [w1719 _]
              tunnel: w1710 -> [w1715 w1737]
              tunnel: w1703 -> [w1714 _]
              frame "Start Task 1", Default {
                # ">> T: Breaks out of state loop; F: Stays in loop>>"
                # ">> Manual override >>"
                # ">> Checks if time is up>>"
                # "Stays in Task 5D until the object is detected"
                # "T: Go back to idle, F: Continue with task\""
                # ">> Manual override >>"
                n584 = case shown="False" w1714 {
                  tunnel: [w1727 w1733] -> w1723
                  tunnel: w1715 -> [w1725 w1731]
                  frame False {
                    n585 = for {
                      tunnel: string[] ["START TIMER", "PROCESS IMAGE", ""] ("element") -> [w1728] mode=indexing
                      shift-right: [w1730] -> w1727
                      shift-left: w1725 -> [w1729]
                      n586 = Enqueue Element(queue=w1729, element=w1728) -> (queue out=w1730:refnum<queue>)  [unwired: 2 in, 2 out]
                    }
                  }
                  frame True {
                    n587 = for {
                      shift-right: [w1735] -> w1733
                      shift-left: w1731 -> [w1736]
                      tunnel: string[] ["READ STEPPER VALUES", "Y STEPPER CONTROL", ""] -> [w1734] mode=indexing
                      n588 = Enqueue Element(queue=w1736, element=w1734) -> (queue out=w1735:refnum<queue>)  [unwired: 2 in, 2 out]
                    }
                  }
                }
                n589 = Or(x=w1714, y=w1719) -> (x .or. y?=w1721:bool)
                n590 = Select(t=State_Type_Definitions,_for_0.26g_versions_and_later_2."True Stop" ("Enum"), s=w1719, f=State_Type_Definitions,_for_0.26g_versions_and_later_2."Task 8H: ARM ADJUST" ("Enum")) -> (s? t:f=w1716:T16)
                n591 = Select(t=w1716, s=w1721, f=State_Type_Definitions,_for_0.26g_versions_and_later_2."Task 8G: PROCESS IMAGE 2" ("Enum")) -> (s? t:f=w1720:T16)
              }
              frame "Exit" {
                n592 = for {
                  shift-right: [w1743] -> w1740
                  shift-left: w1737 -> [w1744]
                  tunnel: string[] ["STOP", "RESET ENCODERS", "RESET YAW", "ARDUINO MODE 0"] -> [w1742] mode=indexing
                  n593 = Enqueue Element(queue=w1744, element=w1742) -> (queue out=w1743:refnum<queue>)  [unwired: 2 in, 2 out]
                }
              }
            }
          }
          frame 34 {
            # ">>> yStepper command>>>"
            n594 = Dequeue Element(queue=w1758, timeout in ms (-1)=w1759, error in (no error)=w1760) -> (element=w1762:T8)  [unwired: 3 out]
            n595 = formula code="if (pos < 70)\ny = 43;\n\nelse if (pos >= 71 &&pos <= 80)\ny = 40;\n\nelse if (pos >= 81 && pos <= 90)\ny = 38;\n\nelse if (pos >= 91 &&pos <= 120)\ny = 35;\n\nelse if (pos >= 121 && pos <= 140)\ny = 30;\n\nelse if (pos >= 141 && pos <= 170)\ny = 26;\n\nelse if (pos >= 171 &&pos <= 220) \ny = 20;\n\nelse if (pos >= 221&& pos <= 240)\ny = 15;\n\nelse if (pos >= 241 && pos <= 250)\ny = 10;\n\nelse if (pos >= 251)\ny = 0;"("pos"=w1750) -> ("y"=w1753:dbl)
            n596 = To Unsigned Byte Integer(number=w1753) -> (unsigned 8bit integer=w1748:u8)
            "Correcte stepper" <- w1748
            n597 = Equal?(x=w1749, y=w1748) -> (x = y?=w1747:bool)
            n598 = case shown="\"Start Task 1\", Default" w1762 {
              tunnel: [w1769 State_Type_Definitions,_for_0.26g_versions_and_later_2."True Stop" ("Enum")] -> w1756
              tunnel: [w1772 w1789] -> w1754
              tunnel: [State_Type_Definitions,_for_0.26g_versions_and_later_2."Idle" ("Enum") State_Type_Definitions,_for_0.26g_versions_and_later_2."Shutdown" ("Enum")] -> w1755
              tunnel: w1761 -> [w1768 _]
              tunnel: w1757 -> [w1764 w1786]
              tunnel: w1747 -> [w1763 _]
              frame "Start Task 1", Default {
                # ">> T: Breaks out of state loop; F: Stays in loop>>"
                # ">> Manual override >>"
                # ">> Checks if time is up>>"
                # "Stays in Task 5D until the object is detected"
                # "T: Go back to idle, F: Continue with task\""
                # ">> Manual override >>"
                n599 = case shown="False" w1763 {
                  tunnel: [w1776 w1782] -> w1772
                  tunnel: w1764 -> [w1774 w1780]
                  frame False {
                    n600 = for {
                      tunnel: string[] ["READ STEPPER VALUES", "Y STEPPER CONTROL", ""] ("element") -> [w1777] mode=indexing
                      shift-right: [w1779] -> w1776
                      shift-left: w1774 -> [w1778]
                      n601 = Enqueue Element(queue=w1778, element=w1777) -> (queue out=w1779:refnum<queue>)  [unwired: 2 in, 2 out]
                    }
                  }
                  frame True {
                    n602 = for {
                      shift-right: [w1784] -> w1782
                      shift-left: w1780 -> [w1785]
                      tunnel: string[] ["DISPOSE BUFFERS", "READ STEPPER VALUES", ""] -> [w1783] mode=indexing
                      n603 = Enqueue Element(queue=w1785, element=w1783) -> (queue out=w1784:refnum<queue>)  [unwired: 2 in, 2 out]
                    }
                  }
                }
                n604 = Or(x=w1763, y=w1768) -> (x .or. y?=w1770:bool)
                n605 = Select(t=State_Type_Definitions,_for_0.26g_versions_and_later_2."True Stop" ("Enum"), s=w1768, f=State_Type_Definitions,_for_0.26g_versions_and_later_2."Task 8I: ARM GRAB HEIGHT" ("Enum")) -> (s? t:f=w1765:T16)
                n606 = Select(t=w1765, s=w1770, f=State_Type_Definitions,_for_0.26g_versions_and_later_2."Task 8H: ARM ADJUST" ("Enum")) -> (s? t:f=w1769:T16)
              }
              frame "Exit" {
                n607 = for {
                  shift-right: [w1792] -> w1789
                  shift-left: w1786 -> [w1793]
                  tunnel: string[] ["STOP", "RESET ENCODERS", "RESET YAW", "ARDUINO MODE 0"] -> [w1791] mode=indexing
                  n608 = Enqueue Element(queue=w1793, element=w1791) -> (queue out=w1792:refnum<queue>)  [unwired: 2 in, 2 out]
                }
              }
            }
            n609 = Bundle By Name(cluster=w1752, "yStepper desired"=w1748) -> (w1751:T18)
          }
          frame 35 {
            # ">>> Motor control cluster >>>"
            # ">>> yStepper command>>>"
            # ">> Manual override >>"
            n610 = Dequeue Element(queue=w1804, timeout in ms (-1)=w1803, error in (no error)=w1805) -> (element=w1802:T8)  [unwired: 3 out]
            n611 = Equal?(x=w1801, y=u8 1) -> (x = y?=w1799:bool)
            n612 = case shown="\"Start Task 1\", Default" w1802 {
              tunnel: [w1815 State_Type_Definitions,_for_0.26g_versions_and_later_2."True Stop" ("Enum")] -> w1806
              tunnel: [w1818 w1835] -> w1807
              tunnel: [State_Type_Definitions,_for_0.26g_versions_and_later_2."Idle" ("Enum") State_Type_Definitions,_for_0.26g_versions_and_later_2."Shutdown" ("Enum")] -> w1808
              tunnel: w1799 -> [w1814 _]
              tunnel: w1798 -> [w1813 _]
              tunnel: w1797 -> [w1809 w1832]
              frame "Start Task 1", Default {
                # "Stays in Task 5F until stepper reaches desired \nheight"
                # "T: Go back to idle, F: Continue with task\""
                # ">> Manual override >>"
                n613 = case shown="True" w1814 {
                  tunnel: [w1822 w1828] -> w1818
                  tunnel: w1809 -> [w1820 w1826]
                  frame False {
                    n614 = for {
                      tunnel: string[] ["Z STEPPER GRAB HEIGHT", "READ STEPPER VALUES"] ("element") -> [w1823] mode=indexing
                      shift-right: [w1825] -> w1822
                      shift-left: w1820 -> [w1824]
                      n615 = Enqueue Element(queue=w1824, element=w1823) -> (queue out=w1825:refnum<queue>)  [unwired: 2 in, 2 out]
                    }
                  }
                  frame True {
                    n616 = for {
                      shift-right: [w1830] -> w1828
                      shift-left: w1826 -> [w1831]
                      tunnel: string[] ["SET TIMER 2", "CLOSE CLAW", ""] -> [w1829] mode=indexing
                      n617 = Enqueue Element(queue=w1831, element=w1829) -> (queue out=w1830:refnum<queue>)  [unwired: 2 in, 2 out]
                    }
                  }
                }
                n618 = Or(x=w1814, y=w1813) -> (x .or. y?=w1816:bool)
                n619 = Select(t=State_Type_Definitions,_for_0.26g_versions_and_later_2."True Stop" ("Enum"), s=w1813, f=State_Type_Definitions,_for_0.26g_versions_and_later_2."Task 8J: CLOSE CLAW" ("Enum")) -> (s? t:f=w1810:T16)
                n620 = Select(t=w1810, s=w1816, f=State_Type_Definitions,_for_0.26g_versions_and_later_2."Task 8I: ARM GRAB HEIGHT" ("Enum")) -> (s? t:f=w1815:T16)
              }
              frame "Exit" {
                n621 = for {
                  shift-right: [w1838] -> w1835
                  shift-left: w1832 -> [w1839]
                  tunnel: string[] ["STOP", "RESET ENCODERS", "RESET YAW", "ARDUINO MODE 0"] -> [w1837] mode=indexing
                  n622 = Enqueue Element(queue=w1839, element=w1837) -> (queue out=w1838:refnum<queue>)  [unwired: 2 in, 2 out]
                }
              }
            }
          }
          frame 36 {
            # ">>> yStepper command>>>"
            # ">> Manual override >>"
            n623 = Dequeue Element(queue=w1850, timeout in ms (-1)=w1849, error in (no error)=w1848) -> (element=w1847:T8)  [unwired: 3 out]
            n624 = case shown="\"Start Task 1\", Default" w1847 {
              tunnel: [w1859 State_Type_Definitions,_for_0.26g_versions_and_later_2."True Stop" ("Enum")] -> w1852
              tunnel: [w1862 w1879] -> w1845
              tunnel: [State_Type_Definitions,_for_0.26g_versions_and_later_2."Idle" ("Enum") State_Type_Definitions,_for_0.26g_versions_and_later_2."Shutdown" ("Enum")] -> w1844
              tunnel: w1846 -> [w1853 _]
              tunnel: w1851 -> [w1858 w1876]
              tunnel: w1842 -> [w1857 _]
              frame "Start Task 1", Default {
                # ">> Is time up? >>"
                # "Determines if object is in range to pick up"
                # ">> Manual override >>"
                n625 = case shown="True" w1857 {
                  tunnel: [w1866 w1872] -> w1862
                  tunnel: w1858 -> [w1864 w1870]
                  frame False {
                    n626 = for {
                      tunnel: string[] ["CLOSE CLAW", "START TIMER"] ("element") -> [w1867] mode=indexing
                      shift-right: [w1869] -> w1866
                      shift-left: w1864 -> [w1868]
                      n627 = Enqueue Element(queue=w1868, element=w1867) -> (queue out=w1869:refnum<queue>)  [unwired: 2 in, 2 out]
                    }
                  }
                  frame True {
                    n628 = for {
                      shift-right: [w1874] -> w1872
                      shift-left: w1870 -> [w1875]
                      tunnel: string[] ["READ STEPPER VALUES", "", ""] -> [w1873] mode=indexing
                      n629 = Enqueue Element(queue=w1875, element=w1873) -> (queue out=w1874:refnum<queue>)  [unwired: 2 in, 2 out]
                    }
                  }
                }
                n630 = Or(x=w1857, y=w1853) -> (x .or. y?=w1860:bool)
                n631 = Select(t=State_Type_Definitions,_for_0.26g_versions_and_later_2."True Stop" ("Enum"), s=w1853, f=State_Type_Definitions,_for_0.26g_versions_and_later_2."Task 8K: RAISE MY SWORD" ("Enum")) -> (s? t:f=w1855:T16)
                n632 = Select(t=w1855, s=w1860, f=State_Type_Definitions,_for_0.26g_versions_and_later_2."Task 8J: CLOSE CLAW" ("Enum")) -> (s? t:f=w1859:T16)
              }
              frame "Exit" {
                n633 = for {
                  shift-right: [w1882] -> w1879
                  shift-left: w1876 -> [w1883]
                  tunnel: string[] ["STOP", "RESET ENCODERS", "RESET YAW", "ARDUINO MODE 0"] -> [w1881] mode=indexing
                  n634 = Enqueue Element(queue=w1883, element=w1881) -> (queue out=w1882:refnum<queue>)  [unwired: 2 in, 2 out]
                }
              }
            }
          }
          frame 37 {
            # ">>> yStepper command>>>"
            # ">> Manual override >>"
            n635 = Dequeue Element(queue=w1894, timeout in ms (-1)=w1893, error in (no error)=w1895) -> (element=w1892:T8)  [unwired: 3 out]
            n636 = Equal?(x=w1891, y=u8 60) -> (x = y?=w1889:bool)
            n637 = case shown="\"Start Task 1\", Default" w1892 {
              tunnel: [w1905 State_Type_Definitions,_for_0.26g_versions_and_later_2."True Stop" ("Enum")] -> w1896
              tunnel: [w1908 w1925] -> w1897
              tunnel: [State_Type_Definitions,_for_0.26g_versions_and_later_2."Idle" ("Enum") State_Type_Definitions,_for_0.26g_versions_and_later_2."Shutdown" ("Enum")] -> w1898
              tunnel: w1889 -> [w1904 _]
              tunnel: w1888 -> [w1903 _]
              tunnel: w1887 -> [w1899 w1922]
              frame "Start Task 1", Default {
                # "Stays in Task 5_A until stepper reaches desired \nheight"
                # "T: Go back to idle, F: Continue with task\""
                # ">> Manual override >>"
                n638 = case shown="True" w1904 {
                  tunnel: [w1912 w1918] -> w1908
                  tunnel: w1899 -> [w1910 w1916]
                  frame False {
                    n639 = for {
                      tunnel: string[] ["Z STEPPER CAM HEIGHT", "READ STEPPER VALUES"] ("element") -> [w1913] mode=indexing
                      shift-right: [w1915] -> w1912
                      shift-left: w1910 -> [w1914]
                      n640 = Enqueue Element(queue=w1914, element=w1913) -> (queue out=w1915:refnum<queue>)  [unwired: 2 in, 2 out]
                    }
                  }
                  frame True {
                    n641 = for {
                      shift-right: [w1920] -> w1918
                      shift-left: w1916 -> [w1921]
                      tunnel: string[] ["CAM CLOSE", "DISPOSE CAM BUFFERS", "DISPOSE PROC BUFFERS", "RESET ENCODERS"] -> [w1919] mode=indexing
                      n642 = Enqueue Element(queue=w1921, element=w1919) -> (queue out=w1920:refnum<queue>)  [unwired: 2 in, 2 out]
                    }
                  }
                }
                n643 = Or(x=w1904, y=w1903) -> (x .or. y?=w1906:bool)
                n644 = Select(t=State_Type_Definitions,_for_0.26g_versions_and_later_2."True Stop" ("Enum"), s=w1903, f=State_Type_Definitions,_for_0.26g_versions_and_later_2."True Stop" ("Enum")) -> (s? t:f=w1900:T16)
                n645 = Select(t=w1900, s=w1906, f=State_Type_Definitions,_for_0.26g_versions_and_later_2."Task 8K: RAISE MY SWORD" ("Enum")) -> (s? t:f=w1905:T16)
              }
              frame "Exit" {
                n646 = for {
                  shift-right: [w1928] -> w1925
                  shift-left: w1922 -> [w1929]
                  tunnel: string[] ["STOP", "RESET ENCODERS", "RESET YAW", "ARDUINO MODE 0"] -> [w1927] mode=indexing
                  n647 = Enqueue Element(queue=w1929, element=w1927) -> (queue out=w1928:refnum<queue>)  [unwired: 2 in, 2 out]
                }
              }
            }
          }
          frame 38 {
            # ">>> Motor control cluster >>>"
            # ">> Stepper height reeached >>"
            # ">>> yStepper command>>>"
            # ">> Manual override >>"
            n648 = Dequeue Element(queue=w1941, timeout in ms (-1)=w1936, error in (no error)=w1940) -> (element=w1944:T8)  [unwired: 3 out]
            n649 = Equal?(x=w1938, y=u8 40) -> (x = y?=w1942:bool)
            n650 = case shown="\"Start Task 1\", Default" w1944 {
              tunnel: [w1955 State_Type_Definitions,_for_0.26g_versions_and_later_2."True Stop" ("Enum")] -> w1934
              tunnel: [w1953 w1970] -> w1933
              tunnel: w1937 -> [w1952 _]
              tunnel: w1939 -> [w1946 _]
              tunnel: [State_Type_Definitions,_for_0.26g_versions_and_later_2."Idle" ("Enum") State_Type_Definitions,_for_0.26g_versions_and_later_2."Shutdown" ("Enum")] -> w1935
              tunnel: w1942 -> [w1945 _]
              frame "Start Task 1", Default {
                # ">> WIill proceed to part ii if not manual override >>"
                # ">>If ENABLE or Trigger is set to true>>"
                n651 = Or(x=w1945, y=w1946) -> (x .or. y?=w1947:bool)
                n652 = case shown="True" w1945 {
                  tunnel: [w1958 w1964] -> w1953
                  tunnel: w1952 -> [w1957 w1963]
                  frame False {
                    n653 = for {
                      shift-right: [w1960] -> w1958
                      shift-left: w1957 -> [w1961]
                      tunnel: string[] ["Z STEPPER BOX HEIGHT", "READ STEPPER VALUES"] ("element") -> [w1959] mode=indexing
                      n654 = Enqueue Element(queue=w1961, element=w1959) -> (queue out=w1960:refnum<queue>)  [unwired: 2 in, 2 out]
                    }
                  }
                  frame True {
                    n655 = for {
                      shift-right: [w1966] -> w1964
                      shift-left: w1963 -> [w1967]
                      tunnel: string[] ["ARDUINO - ULTRASONIC", "READ NAVX", "RESET FLAGS", "", "", ""] -> [w1965] mode=indexing
                      n656 = Enqueue Element(queue=w1967, element=w1965) -> (queue out=w1966:refnum<queue>)  [unwired: 2 in, 2 out]
                    }
                  }
                }
                n657 = Select(t=State_Type_Definitions,_for_0.26g_versions_and_later_2."True Stop" ("Enum"), s=w1946, f=State_Type_Definitions,_for_0.26g_versions_and_later_2."Task 9B: Rotate to Angle" ("Enum")) -> (s? t:f=w1949:T16)
                n658 = Select(t=w1949, s=w1947, f=State_Type_Definitions,_for_0.26g_versions_and_later_2."Task 9A: Raise Arm" ("Enum")) -> (s? t:f=w1955:T16)
              }
              frame "Exit" {
                n659 = for {
                  shift-right: [w1973] -> w1970
                  shift-left: _ -> [w1974]
                  tunnel: string[] ["STOP", "RESET ENCODERS", "RESET YAW", ""] -> [w1972] mode=indexing
                  n660 = Enqueue Element(queue=w1974, element=w1972) -> (queue out=w1973:refnum<queue>)  [unwired: 2 in, 2 out]
                }
              }
            }
          }
          frame 39 {
            # ">>> Motor control cluster >>>"
            # ">>> yStepper command>>>"
            n661 = Dequeue Element(queue=w1988, timeout in ms (-1)=w1987, error in (no error)=w1986) -> (element=w1990:T8)  [unwired: 3 out]
            n662 = In Range and Coerce(upper limit=65.0, x=w1980, lower limit=55.0) -> (In Range?=w1977:bool)  [unwired: 1 out]
            n663 = case shown="\"Start Task 1\", Default" w1990 {
              tunnel: w1981 -> [w1993 _]
              tunnel: [w2001 State_Type_Definitions,_for_0.26g_versions_and_later_2."True Stop" ("Enum")] -> w1983
              tunnel: w1989 -> [w1999 w2017]
              tunnel: [w1998 w2016] -> w1982
              tunnel: [State_Type_Definitions,_for_0.26g_versions_and_later_2."Idle" ("Enum") State_Type_Definitions,_for_0.26g_versions_and_later_2."Shutdown" ("Enum")] -> w1984
              tunnel: w1977 -> [w1991 _]
              frame "Start Task 1", Default {
                n664 = Or(x=w1991, y=w1993) -> (x .or. y?=w1992:bool)
                n665 = case shown="True" w1991 {
                  tunnel: w1999 -> [w2004 w2010]
                  tunnel: [w2003 w2008] -> w1998
                  frame False {
                    n666 = for {
                      shift-right: [w2006] -> w2003
                      shift-left: w2004 -> [w2007]
                      tunnel: string[] ["READ NAVX", "R-CW", "READ ULTRASONIC"] ("element") -> [w2005] mode=indexing
                      n667 = Enqueue Element(queue=w2007, element=w2005) -> (queue out=w2006:refnum<queue>)  [unwired: 2 in, 2 out]
                    }
                  }
                  frame True {
                    n668 = for {
                      shift-right: [w2012] -> w2008
                      shift-left: w2010 -> [w2013]
                      tunnel: string[] ["STOP", "RESET ENCODERS", "RESET YAW", "ARDUINO - ULTRASONIC", ""] -> [w2011] mode=indexing
                      n669 = Enqueue Element(queue=w2013, element=w2011) -> (queue out=w2012:refnum<queue>)  [unwired: 2 in, 2 out]
                    }
                  }
                }
                n670 = Select(t=State_Type_Definitions,_for_0.26g_versions_and_later_2."True Stop" ("Enum"), s=w1993, f=State_Type_Definitions,_for_0.26g_versions_and_later_2."Task 9C: Detect Box") -> (s? t:f=w1995:T16)
                n671 = Select(t=w1995, s=w1992, f=State_Type_Definitions,_for_0.26g_versions_and_later_2."Task 9B: Rotate to Angle" ("Enum")) -> (s? t:f=w2001:T16)
              }
              frame "Exit" {
                n672 = for {
                  shift-right: [w2020] -> w2016
                  shift-left: w2017 -> [w2021]
                  tunnel: string[] ["STOP", "RESET ENCODERS", "RESET YAW", ""] -> [w2019] mode=indexing
                  n673 = Enqueue Element(queue=w2021, element=w2019) -> (queue out=w2020:refnum<queue>)  [unwired: 2 in, 2 out]
                }
              }
            }
          }
          frame 40 {
            # ">>> Motor control cluster >>>"
            # ">>Line Detected>>"
            # ">>Action Queue>>"
            # ">>> yStepper command>>>"
            n674 = Dequeue Element(queue=w2033, timeout in ms (-1)=w2032, error in (no error)=w2031) -> (element=w2034:T8)  [unwired: 3 out]
            n675 = case shown="\"Start Task 1\", Default" w2034 {
              tunnel: w2029 -> [w2035 _]
              tunnel: [w2045 State_Type_Definitions,_for_0.26g_versions_and_later_2."True Stop" ("Enum")] -> w2026
              tunnel: w2030 -> [w2043 w2061]
              tunnel: [w2042 w2060] -> w2025
              tunnel: [State_Type_Definitions,_for_0.26g_versions_and_later_2."Idle" ("Enum") State_Type_Definitions,_for_0.26g_versions_and_later_2."Shutdown" ("Enum")] -> w2028
              tunnel: w2023 -> [w2036 _]
              frame "Start Task 1", Default {
                n676 = Or(x=w2035, y=w2036) -> (x .or. y?=w2037:bool)
                n677 = case shown="True" w2036 {
                  tunnel: w2043 -> [w2048 w2054]
                  tunnel: [w2047 w2052] -> w2042
                  frame False {
                    n678 = for {
                      shift-right: [w2050] -> w2047
                      shift-left: w2048 -> [w2051]
                      tunnel: string[] ["READ IR", "READ LINE SENSOR", "FORWARD - IR ASSIST"] ("element") -> [w2049] mode=indexing
                      n679 = Enqueue Element(queue=w2051, element=w2049) -> (queue out=w2050:refnum<queue>)  [unwired: 2 in, 2 out]
                    }
                  }
                  frame True {
                    n680 = for {
                      shift-right: [w2056] -> w2052
                      shift-left: w2054 -> [w2057]
                      tunnel: string[] ["STOP", "RESET ENCODERS", "RESET YAW", ""] -> [w2055] mode=indexing
                      n681 = Enqueue Element(queue=w2057, element=w2055) -> (queue out=w2056:refnum<queue>)  [unwired: 2 in, 2 out]
                    }
                  }
                }
                n682 = Select(t=State_Type_Definitions,_for_0.26g_versions_and_later_2."True Stop" ("Enum"), s=w2035, f=State_Type_Definitions,_for_0.26g_versions_and_later_2."Task 9D: MOVE FORWARD") -> (s? t:f=w2039:T16)
                n683 = Select(t=w2039, s=w2037, f=State_Type_Definitions,_for_0.26g_versions_and_later_2."Task 9C: Detect Box" ("Enum")) -> (s? t:f=w2045:T16)
              }
              frame "Exit" {
                n684 = for {
                  shift-right: [w2064] -> w2060
                  shift-left: w2061 -> [w2065]
                  tunnel: string[] ["STOP", "RESET ENCODERS", "RESET YAW", ""] -> [w2063] mode=indexing
                  n685 = Enqueue Element(queue=w2065, element=w2063) -> (queue out=w2064:refnum<queue>)  [unwired: 2 in, 2 out]
                }
              }
            }
          }
          frame 41 {
            w2069 = u8 35 ("y")
            # ">> Wall detected >>"
            # ">> Manual override >>"
            # ">>Table Detected>>"
            # ">>> Motor control cluster >>>"
            # ">>Table or wall detectected>>"
            # ">>Action Queue>>"
            # ">>> yStepper command>>>"
            n686 = Less?(x=w2073, y=w2069) -> (x < y?=w2071:bool)
            n687 = Less?(x=w2072, y=w2069) -> (x < y?=w2070:bool)
            n688 = Less Or Equal?(x=w2075, y=15.0) -> (x <= y?=w2066:bool)
            n689 = And(x=w2071, y=w2070) -> (x .and. y?=w2068:bool)
            "Front Wall detected" <- w2068
            n690 = Dequeue Element(queue=w2086, timeout in ms (-1)=w2085, error in (no error)=w2084) -> (element=w2087:T8)  [unwired: 3 out]
            n691 = Or(x=w2066, y=w2068) -> (x .or. y?=w2067:bool)
            n692 = case shown="\"Start Task 1\", Default" w2087 {
              tunnel: w2082 -> [w2088 _]
              tunnel: [w2098 State_Type_Definitions,_for_0.26g_versions_and_later_2."True Stop" ("Enum")] -> w2079
              tunnel: w2083 -> [w2096 w2114]
              tunnel: [w2095 w2113] -> w2078
              tunnel: [State_Type_Definitions,_for_0.26g_versions_and_later_2."Idle" ("Enum") State_Type_Definitions,_for_0.26g_versions_and_later_2."Shutdown" ("Enum")] -> w2081
              tunnel: w2067 -> [w2089 _]
              frame "Start Task 1", Default {
                n693 = Or(x=w2088, y=w2089) -> (x .or. y?=w2090:bool)
                n694 = case shown="False" w2089 {
                  tunnel: w2096 -> [w2101 w2107]
                  tunnel: [w2100 w2105] -> w2095
                  frame False {
                    n695 = for {
                      shift-right: [w2103] -> w2100
                      shift-left: w2101 -> [w2104]
                      tunnel: string[] ["READ IR", "FORWARD - IR ASSIST", "READ ULTRASONIC"] ("element") -> [w2102] mode=indexing
                      n696 = Enqueue Element(queue=w2104, element=w2102) -> (queue out=w2103:refnum<queue>)  [unwired: 2 in, 2 out]
                    }
                  }
                  frame True {
                    n697 = for {
                      shift-right: [w2109] -> w2105
                      shift-left: w2107 -> [w2110]
                      tunnel: string[] ["STOP", "RESET ENCODERS", "RESET YAW", ""] -> [w2108] mode=indexing
                      n698 = Enqueue Element(queue=w2110, element=w2108) -> (queue out=w2109:refnum<queue>)  [unwired: 2 in, 2 out]
                    }
                  }
                }
                n699 = Select(t=State_Type_Definitions,_for_0.26g_versions_and_later_2."True Stop" ("Enum"), s=w2088, f=State_Type_Definitions,_for_0.26g_versions_and_later_2."True Stop") -> (s? t:f=w2092:T16)
                n700 = Select(t=w2092, s=w2090, f=State_Type_Definitions,_for_0.26g_versions_and_later_2."Task 9D: MOVE FORWARD" ("Enum")) -> (s? t:f=w2098:T16)
              }
              frame "Exit" {
                n701 = for {
                  shift-right: [w2117] -> w2113
                  shift-left: w2114 -> [w2118]
                  tunnel: string[] ["STOP", "RESET ENCODERS", "RESET YAW", ""] -> [w2116] mode=indexing
                  n702 = Enqueue Element(queue=w2118, element=w2116) -> (queue out=w2117:refnum<queue>)  [unwired: 2 in, 2 out]
                }
              }
            }
          }
          frame 42 {
            # ">> Item Selection Bias >>"
            # ">> Line detected? >>"
            # ">> Manual override >>"
            # ">>> Motor control cluster >>>"
            # ">>Action Queue>>"
            # ">>> yStepper command>>>"
            n703 = Dequeue Element(queue=w2130, timeout in ms (-1)=w2129, error in (no error)=w2128) -> (element=w2131:T8)  [unwired: 3 out]
            n704 = case shown="\"Start Task 1\", Default" w2131 {
              tunnel: w2126 -> [w2132 _]
              tunnel: [w2142 State_Type_Definitions,_for_0.26g_versions_and_later_2."True Stop" ("Enum")] -> w2123
              tunnel: w2127 -> [w2140 w2158]
              tunnel: [w2139 w2157] -> w2122
              tunnel: [State_Type_Definitions,_for_0.26g_versions_and_later_2."Idle" ("Enum") State_Type_Definitions,_for_0.26g_versions_and_later_2."Shutdown" ("Enum")] -> w2125
              tunnel: w2119 -> [w2133 _]
              frame "Start Task 1", Default {
                n705 = Or(x=w2132, y=w2133) -> (x .or. y?=w2134:bool)
                n706 = case shown="False" w2133 {
                  tunnel: w2140 -> [w2145 w2151]
                  tunnel: [w2144 w2149] -> w2139
                  frame False {
                    n707 = for {
                      shift-right: [w2147] -> w2144
                      shift-left: w2145 -> [w2148]
                      tunnel: string[] ["LEFT", "READ NAVX", "READ LINE SENSOR", ""] ("element") -> [w2146] mode=indexing
                      n708 = Enqueue Element(queue=w2148, element=w2146) -> (queue out=w2147:refnum<queue>)  [unwired: 2 in, 2 out]
                    }
                  }
                  frame True {
                    n709 = for {
                      shift-right: [w2153] -> w2149
                      shift-left: w2151 -> [w2154]
                      tunnel: string[] ["STOP", "RESET ENCODERS", "RESET YAW", "RESET FLAGS", "OPEN LIFE CAM", "SET TIMER 2"] -> [w2152] mode=indexing
                      n710 = Enqueue Element(queue=w2154, element=w2152) -> (queue out=w2153:refnum<queue>)  [unwired: 2 in, 2 out]
                    }
                  }
                }
                n711 = Select(t=State_Type_Definitions,_for_0.26g_versions_and_later_2."True Stop" ("Enum"), s=w2132, f=State_Type_Definitions."Task 9F: SCAN IMAGE") -> (s? t:f=w2136:u16)
                n712 = Select(t=w2136, s=w2134, f=State_Type_Definitions,_for_0.26g_versions_and_later_2."Task 9E: MOVE LEFT" ("Enum")) -> (s? t:f=w2142:u16)
              }
              frame "Exit" {
                n713 = for {
                  shift-right: [w2161] -> w2157
                  shift-left: w2158 -> [w2162]
                  tunnel: string[] ["STOP", "RESET ENCODERS", "RESET YAW", ""] -> [w2160] mode=indexing
                  n714 = Enqueue Element(queue=w2162, element=w2160) -> (queue out=w2161:refnum<queue>)  [unwired: 2 in, 2 out]
                }
              }
            }
          }
          frame 43 {
            # ">>> Motor control cluster >>>"
            # ">>Time up? >>"
            # ">>> yStepper command>>>"
            # ">> Manual override >>"
            n715 = Dequeue Element(queue=w2174, timeout in ms (-1)=w2170, error in (no error)=w2173) -> (element=w2175:T8)  [unwired: 3 out]
            n716 = case shown="\"Start Task 1\", Default" w2175 {
              tunnel: [w2186 State_Type_Definitions,_for_0.26g_versions_and_later_2."True Stop" ("Enum")] -> w2168
              tunnel: [w2184 w2202] -> w2167
              tunnel: w2171 -> [w2183 w2199]
              tunnel: w2172 -> [w2177 _]
              tunnel: [State_Type_Definitions,_for_0.26g_versions_and_later_2."Idle" ("Enum") State_Type_Definitions,_for_0.26g_versions_and_later_2."Shutdown" ("Enum")] -> w2169
              tunnel: w2163 -> [w2176 _]
              frame "Start Task 1", Default {
                # ">> WIill proceed to part ii if not manual override >>"
                # ">>If ENABLE or Trigger is set to true>>"
                n717 = Or(x=w2176, y=w2177) -> (x .or. y?=w2178:bool)
                n718 = case shown="True" w2176 {
                  tunnel: [w2189 w2195] -> w2184
                  tunnel: w2183 -> [w2188 w2194]
                  frame False {
                    n719 = for {
                      shift-right: [w2191] -> w2189
                      shift-left: w2188 -> [w2192]
                      tunnel: string[] ["CAM ACQ", "START TIMER"] ("element") -> [w2190] mode=indexing
                      n720 = Enqueue Element(queue=w2192, element=w2190) -> (queue out=w2191:refnum<queue>)  [unwired: 2 in, 2 out]
                    }
                  }
                  frame True {
                    n721 = for {
                      shift-right: [w2197] -> w2195
                      shift-left: w2194 -> [w2198]
                      tunnel: string[] ["CLOSE CAM", "SET TIMER 5", "", "", "", ""] -> [w2196] mode=indexing
                      n722 = Enqueue Element(queue=w2198, element=w2196) -> (queue out=w2197:refnum<queue>)  [unwired: 2 in, 2 out]
                    }
                  }
                }
                n723 = Select(t=State_Type_Definitions,_for_0.26g_versions_and_later_2."True Stop" ("Enum"), s=w2177, f=State_Type_Definitions."Task 9G: PROCESS COLOUR" ("Enum")) -> (s? t:f=w2180:u16)
                n724 = Select(t=w2180, s=w2178, f=State_Type_Definitions."Task 9F: SCAN IMAGE" ("Enum")) -> (s? t:f=w2186:u16)
              }
              frame "Exit" {
                n725 = for {
                  shift-right: [w2205] -> w2202
                  shift-left: w2199 -> [w2206]
                  tunnel: string[] ["STOP", "RESET ENCODERS", "RESET YAW", ""] -> [w2204] mode=indexing
                  n726 = Enqueue Element(queue=w2206, element=w2204) -> (queue out=w2205:refnum<queue>)  [unwired: 2 in, 2 out]
                }
              }
            }
          }
          frame 44 {
            # ">>> Motor control cluster >>>"
            # ">>> yStepper command>>>"
            # ">>Object detected>>"
            n727 = Less Or Equal?(x=w2210, y=30.0) -> (x <= y?=w2208:bool)
            "Table obstruct" <- w2208
            n728 = Dequeue Element(queue=w2216, timeout in ms (-1)=w2215, error in (no error)=w2214) -> (element=w2221:T8)  [unwired: 3 out]
            n729 = case shown="\"Start Task 1\", Default" w2221 {
              tunnel: w2208 -> [w2224 _]
              tunnel: [w2231 State_Type_Definitions,_for_0.26g_versions_and_later_2."True Stop" ("Enum")] -> w2220
              tunnel: w2213 -> [w2223 _]
              tunnel: w2217 -> [w2230 w2247]
              tunnel: [w2229 w2248] -> w2219
              tunnel: [State_Type_Definitions,_for_0.26g_versions_and_later_2."Idle" ("Enum") State_Type_Definitions,_for_0.26g_versions_and_later_2."Shutdown" ("Enum")] -> w2218
              frame "Start Task 1", Default {
                n730 = case shown="True" w2224 {
                  tunnel: w2230 -> [w2234 w2241]
                  tunnel: [w2235 w2240] -> w2229
                  frame False {
                    n731 = for {
                      tunnel: string[] ["START TIMER", "COLOUR PROCESSING", ""] ("element") -> [w2236] mode=indexing
                      shift-right: [w2238] -> w2235
                      shift-left: w2234 -> [w2237]
                      n732 = Enqueue Element(queue=w2237, element=w2236) -> (queue out=w2238:refnum<queue>)  [unwired: 2 in, 2 out]
                    }
                  }
                  frame True {
                    n733 = for {
                      shift-right: [w2243] -> w2240
                      shift-left: w2241 -> [w2244]
                      tunnel: string[] ["DISPOSE BUFFERS", "CLOSE CAM", "RESET ENCODERS", "RESET YAW", "RESET FLAGS"] -> [w2242] mode=indexing
                      n734 = Enqueue Element(queue=w2244, element=w2242) -> (queue out=w2243:refnum<queue>)  [unwired: 2 in, 2 out]
                    }
                  }
                }
                n735 = Or(x=w2224, y=w2223) -> (x .or. y?=w2222:bool)
                n736 = Select(t=State_Type_Definitions,_for_0.26g_versions_and_later_2."True Stop" ("Enum"), s=w2223, f=State_Type_Definitions."Task 9H: MOVE RIGHT" ("Enum")) -> (s? t:f=w2225:u16)
                n737 = Select(t=w2225, s=w2222, f=State_Type_Definitions."Task 9G: PROCESS COLOUR" ("Enum")) -> (s? t:f=w2231:u16)
              }
              frame "Exit" {
                n738 = for {
                  shift-right: [w2251] -> w2248
                  shift-left: w2247 -> [w2252]
                  tunnel: string[] ["STOP", "RESET ENCODERS", "RESET YAW", "ARDUINO MODE 0"] -> [w2250] mode=indexing
                  n739 = Enqueue Element(queue=w2252, element=w2250) -> (queue out=w2251:refnum<queue>)  [unwired: 2 in, 2 out]
                }
              }
            }
          }
          frame 45 {
            # ">> Item Selection Bias >>"
            # ">>> Motor control cluster >>>"
            # ">>> yStepper command>>>"
            n740 = Dequeue Element(queue=w2262, timeout in ms (-1)=w2263, error in (no error)=w2264) -> (element=w2266:T8)  [unwired: 3 out]
            n741 = Greater?(x=w2254, y=50.0) -> (0:w2255:bool)
            n742 = And(x=w2256, y=w2255) -> (x .and. y?=w2257:bool)
            n743 = case shown="\"Start Task 1\", Default" w2266 {
              tunnel: w2257 -> [w2272 _]
              tunnel: [w2279 State_Type_Definitions,_for_0.26g_versions_and_later_2."True Stop" ("Enum")] -> w2259
              tunnel: w2265 -> [w2271 _]
              tunnel: w2261 -> [w2278 w2295]
              tunnel: [w2277 w2296] -> w2260
              tunnel: [State_Type_Definitions,_for_0.26g_versions_and_later_2."Idle" ("Enum") State_Type_Definitions,_for_0.26g_versions_and_later_2."Shutdown" ("Enum")] -> w2258
              frame "Start Task 1", Default {
                n744 = case shown="False" w2272 {
                  tunnel: w2278 -> [w2282 w2289]
                  tunnel: [w2283 w2288] -> w2277
                  frame False {
                    n745 = for {
                      tunnel: string[] ["READ LINE SENSOR", "READ NAVX", "RIGHT", "READ ENCODERS"] ("element") -> [w2284] mode=indexing
                      shift-right: [w2286] -> w2283
                      shift-left: w2282 -> [w2285]
                      n746 = Enqueue Element(queue=w2285, element=w2284) -> (queue out=w2286:refnum<queue>)  [unwired: 2 in, 2 out]
                    }
                  }
                  frame True {
                    n747 = for {
                      shift-right: [w2291] -> w2288
                      shift-left: w2289 -> [w2292]
                      tunnel: string[] ["STOP", "RESET ENCODERS", "RESET YAW", "OPEN LIFE CAM", "SET TIMER 2", "RESET FLAGS"] -> [w2290] mode=indexing
                      n748 = Enqueue Element(queue=w2292, element=w2290) -> (queue out=w2291:refnum<queue>)  [unwired: 2 in, 2 out]
                    }
                  }
                }
                n749 = Or(x=w2272, y=w2271) -> (x .or. y?=w2270:bool)
                n750 = Select(t=State_Type_Definitions,_for_0.26g_versions_and_later_2."True Stop" ("Enum"), s=w2271, f=State_Type_Definitions."Task 9I: SCAN IMAGE" ("Enum")) -> (s? t:f=w2273:u16)
                n751 = Select(t=w2273, s=w2270, f=State_Type_Definitions."Task 9H: MOVE RIGHT" ("Enum")) -> (s? t:f=w2279:u16)
              }
              frame "Exit" {
                n752 = for {
                  shift-right: [w2299] -> w2296
                  shift-left: w2295 -> [w2300]
                  tunnel: string[] ["STOP", "RESET ENCODERS", "RESET YAW", "ARDUINO MODE 0"] -> [w2298] mode=indexing
                  n753 = Enqueue Element(queue=w2300, element=w2298) -> (queue out=w2299:refnum<queue>)  [unwired: 2 in, 2 out]
                }
              }
            }
          }
          frame 46 {
            # ">> Item Selection Bias >>"
            n754 = Dequeue Element(queue=w2302, timeout in ms (-1)=w2303, error in (no error)=w2304) -> (element=w2310:T8)  [unwired: 3 out]
            n755 = case shown="\"Start Task 1\", Default" w2310 {
              tunnel: w2301 -> [w2316 _]
              tunnel: [w2323 State_Type_Definitions,_for_0.26g_versions_and_later_2."True Stop" ("Enum")] -> w2307
              tunnel: w2305 -> [w2315 _]
              tunnel: w2309 -> [w2322 w2339]
              tunnel: [w2321 w2340] -> w2308
              tunnel: [State_Type_Definitions,_for_0.26g_versions_and_later_2."Idle" ("Enum") State_Type_Definitions,_for_0.26g_versions_and_later_2."Shutdown" ("Enum")] -> w2306
              frame "Start Task 1", Default {
                n756 = case shown="True" w2316 {
                  tunnel: w2322 -> [w2326 w2333]
                  tunnel: [w2327 w2332] -> w2321
                  frame False {
                    n757 = for {
                      tunnel: string[] ["START TIMER", "CAM ACQ", ""] ("element") -> [w2328] mode=indexing
                      shift-right: [w2330] -> w2327
                      shift-left: w2326 -> [w2329]
                      n758 = Enqueue Element(queue=w2329, element=w2328) -> (queue out=w2330:refnum<queue>)  [unwired: 2 in, 2 out]
                    }
                  }
                  frame True {
                    n759 = for {
                      shift-right: [w2335] -> w2332
                      shift-left: w2333 -> [w2336]
                      tunnel: string[] ["CLOSE CAM", "SET TIMER 5", "", "", "", ""] -> [w2334] mode=indexing
                      n760 = Enqueue Element(queue=w2336, element=w2334) -> (queue out=w2335:refnum<queue>)  [unwired: 2 in, 2 out]
                    }
                  }
                }
                n761 = Or(x=w2316, y=w2315) -> (x .or. y?=w2314:bool)
                n762 = Select(t=State_Type_Definitions,_for_0.26g_versions_and_later_2."True Stop" ("Enum"), s=w2315, f=State_Type_Definitions."Task 9J: PROCESS COLOUR" ("Enum")) -> (s? t:f=w2317:u16)
                n763 = Select(t=w2317, s=w2314, f=State_Type_Definitions."Task 9I: SCAN IMAGE" ("Enum")) -> (s? t:f=w2323:u16)
              }
              frame "Exit" {
                n764 = for {
                  shift-right: [w2343] -> w2340
                  shift-left: w2339 -> [w2344]
                  tunnel: string[] ["STOP", "RESET ENCODERS", "RESET YAW", "ARDUINO MODE 0"] -> [w2342] mode=indexing
                  n765 = Enqueue Element(queue=w2344, element=w2342) -> (queue out=w2343:refnum<queue>)  [unwired: 2 in, 2 out]
                }
              }
            }
          }
          frame 47 {
            # ">> Item Selection Bias >>"
            n766 = Dequeue Element(queue=w2350, timeout in ms (-1)=w2351, error in (no error)=w2352) -> (element=w2354:T8)  [unwired: 3 out]
            n767 = case shown="\"Start Task 1\", Default" w2354 {
              tunnel: w2345 -> [w2360 _]
              tunnel: [w2367 State_Type_Definitions,_for_0.26g_versions_and_later_2."True Stop" ("Enum")] -> w2348
              tunnel: w2353 -> [w2359 _]
              tunnel: w2349 -> [w2366 w2383]
              tunnel: [w2365 w2384] -> w2347
              tunnel: [State_Type_Definitions,_for_0.26g_versions_and_later_2."Idle" ("Enum") State_Type_Definitions,_for_0.26g_versions_and_later_2."Shutdown" ("Enum")] -> w2346
              frame "Start Task 1", Default {
                n768 = case shown="True" w2360 {
                  tunnel: w2366 -> [w2370 w2377]
                  tunnel: [w2371 w2376] -> w2365
                  frame False {
                    n769 = for {
                      tunnel: string[] ["START TIMER", "COLOUR PROCESSING", ""] ("element") -> [w2372] mode=indexing
                      shift-right: [w2374] -> w2371
                      shift-left: w2370 -> [w2373]
                      n770 = Enqueue Element(queue=w2373, element=w2372) -> (queue out=w2374:refnum<queue>)  [unwired: 2 in, 2 out]
                    }
                  }
                  frame True {
                    n771 = for {
                      shift-right: [w2379] -> w2376
                      shift-left: w2377 -> [w2380]
                      tunnel: string[] ["CLOSE CAM", "DISPOSE BUFFERS", "RESET ENCODERS", "RESET YAW", "RESET FLAGS", ""] -> [w2378] mode=indexing
                      n772 = Enqueue Element(queue=w2380, element=w2378) -> (queue out=w2379:refnum<queue>)  [unwired: 2 in, 2 out]
                    }
                  }
                }
                n773 = Or(x=w2360, y=w2359) -> (x .or. y?=w2358:bool)
                n774 = Select(t=State_Type_Definitions,_for_0.26g_versions_and_later_2."True Stop" ("Enum"), s=w2359, f=State_Type_Definitions."Task 9K: ROTATE 90 CW" ("Enum")) -> (s? t:f=w2361:u16)
                n775 = Select(t=w2361, s=w2358, f=State_Type_Definitions."Task 9J: PROCESS COLOUR" ("Enum")) -> (s? t:f=w2367:u16)
              }
              frame "Exit" {
                n776 = for {
                  shift-right: [w2387] -> w2384
                  shift-left: w2383 -> [w2388]
                  tunnel: string[] ["STOP", "RESET ENCODERS", "RESET YAW", "ARDUINO MODE 0"] -> [w2386] mode=indexing
                  n777 = Enqueue Element(queue=w2388, element=w2386) -> (queue out=w2387:refnum<queue>)  [unwired: 2 in, 2 out]
                }
              }
            }
          }
          frame 48 {
            # ">>> Motor control cluster >>>"
            # ">>> yStepper command>>>"
            # ">> Item Selection Bias >>"
            n778 = Less?(x=w2392, y=-38.0) -> (x < y?=w2390:bool)
            n779 = Dequeue Element(queue=w2398, timeout in ms (-1)=w2397, error in (no error)=w2396) -> (element=w2400:T8)  [unwired: 3 out]
            n780 = case shown="\"Start Task 1\", Default" w2400 {
              tunnel: w2390 -> [w2406 _]
              tunnel: [w2413 State_Type_Definitions,_for_0.26g_versions_and_later_2."True Stop" ("Enum")] -> w2394
              tunnel: w2395 -> [w2405 _]
              tunnel: w2399 -> [w2412 w2429]
              tunnel: [w2411 w2430] -> w2389
              tunnel: [State_Type_Definitions,_for_0.26g_versions_and_later_2."Idle" ("Enum") State_Type_Definitions,_for_0.26g_versions_and_later_2."Shutdown" ("Enum")] -> w2393
              frame "Start Task 1", Default {
                n781 = case shown="True" w2406 {
                  tunnel: w2412 -> [w2416 w2423]
                  tunnel: [w2417 w2422] -> w2411
                  frame False {
                    n782 = for {
                      tunnel: string[] ["READ ENCODERS", "R-CW"] ("element") -> [w2418] mode=indexing
                      shift-right: [w2420] -> w2417
                      shift-left: w2416 -> [w2419]
                      n783 = Enqueue Element(queue=w2419, element=w2418) -> (queue out=w2420:refnum<queue>)  [unwired: 2 in, 2 out]
                    }
                  }
                  frame True {
                    n784 = for {
                      shift-right: [w2425] -> w2422
                      shift-left: w2423 -> [w2426]
                      tunnel: string[] ["STOP", "RESET ENCODERS", "RESET FLAGS", "RESET YAW", "READ IR", "ARDUINO - ULTRASONIC"] -> [w2424] mode=indexing
                      n785 = Enqueue Element(queue=w2426, element=w2424) -> (queue out=w2425:refnum<queue>)  [unwired: 2 in, 2 out]
                    }
                  }
                }
                n786 = Or(x=w2406, y=w2405) -> (x .or. y?=w2404:bool)
                n787 = Select(t=State_Type_Definitions,_for_0.26g_versions_and_later_2."True Stop" ("Enum"), s=w2405, f=State_Type_Definitions."Task 9L: MOVE FORWARD" ("Enum")) -> (s? t:f=w2407:u16)
                n788 = Select(t=w2407, s=w2404, f=State_Type_Definitions."Task 9K: ROTATE 90 CW" ("Enum")) -> (s? t:f=w2413:u16)
              }
              frame "Exit" {
                n789 = for {
                  shift-right: [w2433] -> w2430
                  shift-left: w2429 -> [w2434]
                  tunnel: string[] ["STOP", "RESET ENCODERS", "RESET YAW", "ARDUINO MODE 0"] -> [w2432] mode=indexing
                  n790 = Enqueue Element(queue=w2434, element=w2432) -> (queue out=w2433:refnum<queue>)  [unwired: 2 in, 2 out]
                }
              }
            }
          }
          frame 49 {
            w2447 = u8 50 ("y")
            # ">>> Motor control cluster >>>"
            # ">>> yStepper command>>>"
            # ">> Item Selection Bias >>"
            n791 = Less?(x=w2449, y=w2447) -> (x < y?=w2442:bool)
            n792 = Dequeue Element(queue=w2453, timeout in ms (-1)=w2452, error in (no error)=w2451) -> (element=w2457:T8)  [unwired: 3 out]
            n793 = Less?(x=w2448, y=w2447) -> (x < y?=w2443:bool)
            n794 = And(x=w2443, y=w2442) -> (x .and. y?=w2435:bool)
            n795 = Less Or Equal?(x=w2446, y=15.0) -> (x <= y?=w2441:bool)
            n796 = Greater?(x=w2440, y=100.0) -> (0:w2439:bool)
            n797 = Or(x=w2441, y=w2435) -> (x .or. y?=w2437:bool)
            n798 = And(x=w2439, y=w2437) -> (x .and. y?=w2438:bool)
            "Stop?" <- w2438
            n799 = case shown="\"Start Task 1\", Default" w2457 {
              tunnel: w2438 -> [w2463 _]
              tunnel: [w2470 State_Type_Definitions,_for_0.26g_versions_and_later_2."True Stop" ("Enum")] -> w2455
              tunnel: w2450 -> [w2462 _]
              tunnel: w2454 -> [w2469 w2486]
              tunnel: [w2468 w2487] -> w2444
              tunnel: [State_Type_Definitions,_for_0.26g_versions_and_later_2."Idle" ("Enum") State_Type_Definitions,_for_0.26g_versions_and_later_2."Shutdown" ("Enum")] -> w2456
              frame "Start Task 1", Default {
                n800 = case shown="True" w2463 {
                  tunnel: w2469 -> [w2473 w2480]
                  tunnel: [w2474 w2479] -> w2468
                  frame False {
                    n801 = for {
                      tunnel: string[] ["READ IR", "FORWARD", "READ NAVX", "READ ENCODERS"] ("element") -> [w2475] mode=indexing
                      shift-right: [w2477] -> w2474
                      shift-left: w2473 -> [w2476]
                      n802 = Enqueue Element(queue=w2476, element=w2475) -> (queue out=w2477:refnum<queue>)  [unwired: 2 in, 2 out]
                    }
                  }
                  frame True {
                    n803 = for {
                      shift-right: [w2482] -> w2479
                      shift-left: w2480 -> [w2483]
                      tunnel: string[] ["STOP", "RESET ENCODERS", "RESET FLAGS", "RESET YAW", "", ""] -> [w2481] mode=indexing
                      n804 = Enqueue Element(queue=w2483, element=w2481) -> (queue out=w2482:refnum<queue>)  [unwired: 2 in, 2 out]
                    }
                  }
                }
                n805 = Or(x=w2463, y=w2462) -> (x .or. y?=w2461:bool)
                n806 = Select(t=State_Type_Definitions,_for_0.26g_versions_and_later_2."True Stop" ("Enum"), s=w2462, f=State_Type_Definitions,_for_0.26g_versions_and_later_2."True Stop" ("Enum")) -> (s? t:f=w2464:T16)
                n807 = Select(t=w2464, s=w2461, f=State_Type_Definitions."Task 9L: MOVE FORWARD" ("Enum")) -> (s? t:f=w2470:u16)
              }
              frame "Exit" {
                n808 = for {
                  shift-right: [w2490] -> w2487
                  shift-left: w2486 -> [w2491]
                  tunnel: string[] ["STOP", "RESET ENCODERS", "RESET YAW", "ARDUINO MODE 0"] -> [w2489] mode=indexing
                  n809 = Enqueue Element(queue=w2491, element=w2489) -> (queue out=w2490:refnum<queue>)  [unwired: 2 in, 2 out]
                }
              }
            }
          }
          frame 50 {
            # ">> Item Selection Bias >>"
            n810 = Dequeue Element(queue=w2496, timeout in ms (-1)=w2495, error in (no error)=w2494) -> (element=w2501:T8)  [unwired: 3 out]
            n811 = case shown="\"Start Task 1\", Default" w2501 {
              tunnel: w2492 -> [w2507 _]
              tunnel: [w2514 State_Type_Definitions,_for_0.26g_versions_and_later_2."True Stop" ("Enum")] -> w2499
              tunnel: w2493 -> [w2506 _]
              tunnel: w2497 -> [w2513 w2530]
              tunnel: [w2512 w2531] -> w2498
              tunnel: [State_Type_Definitions,_for_0.26g_versions_and_later_2."Idle" ("Enum") State_Type_Definitions,_for_0.26g_versions_and_later_2."Shutdown" ("Enum")] -> w2500
              frame "Start Task 1", Default {
                n812 = case shown="False" w2507 {
                  tunnel: w2513 -> [w2517 w2524]
                  tunnel: [w2518 w2523] -> w2512
                  frame False {
                    n813 = for {
                      tunnel: string[] ["READ LINE SENSOR", "READ NAVX", "RIGHT", "READ ENCODERS"] ("element") -> [w2519] mode=indexing
                      shift-right: [w2521] -> w2518
                      shift-left: w2517 -> [w2520]
                      n814 = Enqueue Element(queue=w2520, element=w2519) -> (queue out=w2521:refnum<queue>)  [unwired: 2 in, 2 out]
                    }
                  }
                  frame True {
                    n815 = for {
                      shift-right: [w2526] -> w2523
                      shift-left: w2524 -> [w2527]
                      tunnel: string[] ["STOP", "RESET ENCODERS", "RESET YAW", "OPEN LIFE CAM", "SET TIMER 2", "RESET FLAGS"] -> [w2525] mode=indexing
                      n816 = Enqueue Element(queue=w2527, element=w2525) -> (queue out=w2526:refnum<queue>)  [unwired: 2 in, 2 out]
                    }
                  }
                }
                n817 = Or(x=w2507, y=w2506) -> (x .or. y?=w2505:bool)
                n818 = Select(t=State_Type_Definitions,_for_0.26g_versions_and_later_2."True Stop" ("Enum"), s=w2506, f=State_Type_Definitions."Task 9N: SCAN IMAGE" ("Enum")) -> (s? t:f=w2508:u16)
                n819 = Select(t=w2508, s=w2505, f=State_Type_Definitions,_for_0.26g_versions_and_later_2."Task 9M: MOVE RIGHT" ("Enum")) -> (s? t:f=w2514:u16)
              }
              frame "Exit" {
                n820 = for {
                  shift-right: [w2534] -> w2531
                  shift-left: w2530 -> [w2535]
                  tunnel: string[] ["STOP", "RESET ENCODERS", "RESET YAW", "ARDUINO MODE 0"] -> [w2533] mode=indexing
                  n821 = Enqueue Element(queue=w2535, element=w2533) -> (queue out=w2534:refnum<queue>)  [unwired: 2 in, 2 out]
                }
              }
            }
          }
          frame 51 {
            # ">> Manual override >>"
            n822 = Dequeue Element(queue=w2544, timeout in ms (-1)=w2543, error in (no error)=w2542) -> (element=w2545:T8)  [unwired: 3 out]
            n823 = case shown="\"Start Task 1\", Default" w2545 {
              tunnel: [w2559 State_Type_Definitions,_for_0.26g_versions_and_later_2."True Stop" ("Enum")] -> w2537
              tunnel: [w2557 w2575] -> w2536
              tunnel: w2540 -> [w2556 w2572]
              tunnel: w2541 -> [w2550 _]
              tunnel: [State_Type_Definitions,_for_0.26g_versions_and_later_2."Idle" ("Enum") State_Type_Definitions,_for_0.26g_versions_and_later_2."Shutdown" ("Enum")] -> w2538
              tunnel: w2539 -> [w2549 _]
              frame "Start Task 1", Default {
                # ">> WIill proceed to part ii if not manual override >>"
                # ">>If ENABLE or Trigger is set to true>>"
                n824 = Or(x=w2549, y=w2550) -> (x .or. y?=w2551:bool)
                n825 = case shown="False" w2549 {
                  tunnel: [w2562 w2568] -> w2557
                  tunnel: w2556 -> [w2561 w2567]
                  frame False {
                    n826 = for {
                      shift-right: [w2564] -> w2562
                      shift-left: w2561 -> [w2565]
                      tunnel: string[] ["CAM ACQ", "START TIMER"] ("element") -> [w2563] mode=indexing
                      n827 = Enqueue Element(queue=w2565, element=w2563) -> (queue out=w2564:refnum<queue>)  [unwired: 2 in, 2 out]
                    }
                  }
                  frame True {
                    n828 = for {
                      shift-right: [w2570] -> w2568
                      shift-left: w2567 -> [w2571]
                      tunnel: string[] ["CLOSE CAM", "SET TIMER 5", "", "", "", ""] -> [w2569] mode=indexing
                      n829 = Enqueue Element(queue=w2571, element=w2569) -> (queue out=w2570:refnum<queue>)  [unwired: 2 in, 2 out]
                    }
                  }
                }
                n830 = Select(t=State_Type_Definitions,_for_0.26g_versions_and_later_2."True Stop" ("Enum"), s=w2550, f=State_Type_Definitions."Task 9O: PROCESS COLOUR" ("Enum")) -> (s? t:f=w2553:u16)
                n831 = Select(t=w2553, s=w2551, f=State_Type_Definitions."Task 9N: SCAN IMAGE" ("Enum")) -> (s? t:f=w2559:u16)
              }
              frame "Exit" {
                n832 = for {
                  shift-right: [w2578] -> w2575
                  shift-left: w2572 -> [w2579]
                  tunnel: string[] ["STOP", "RESET ENCODERS", "RESET YAW", ""] -> [w2577] mode=indexing
                  n833 = Enqueue Element(queue=w2579, element=w2577) -> (queue out=w2578:refnum<queue>)  [unwired: 2 in, 2 out]
                }
              }
            }
          }
          frame 52 {
            # ">> Item Selection Bias >>"
            n834 = Dequeue Element(queue=w2587, timeout in ms (-1)=w2586, error in (no error)=w2585) -> (element=w2589:T8)  [unwired: 3 out]
            n835 = case shown="\"Start Task 1\", Default" w2589 {
              tunnel: w2580 -> [w2595 _]
              tunnel: [w2602 State_Type_Definitions,_for_0.26g_versions_and_later_2."True Stop" ("Enum")] -> w2583
              tunnel: w2584 -> [w2594 _]
              tunnel: w2588 -> [w2601 w2618]
              tunnel: [w2600 w2619] -> w2582
              tunnel: [State_Type_Definitions,_for_0.26g_versions_and_later_2."Idle" ("Enum") State_Type_Definitions,_for_0.26g_versions_and_later_2."Shutdown" ("Enum")] -> w2581
              frame "Start Task 1", Default {
                n836 = case shown="False" w2595 {
                  tunnel: w2601 -> [w2605 w2612]
                  tunnel: [w2606 w2611] -> w2600
                  frame False {
                    n837 = for {
                      tunnel: string[] ["START TIMER", "COLOUR PROCESSING", ""] ("element") -> [w2607] mode=indexing
                      shift-right: [w2609] -> w2606
                      shift-left: w2605 -> [w2608]
                      n838 = Enqueue Element(queue=w2608, element=w2607) -> (queue out=w2609:refnum<queue>)  [unwired: 2 in, 2 out]
                    }
                  }
                  frame True {
                    n839 = for {
                      shift-right: [w2614] -> w2611
                      shift-left: w2612 -> [w2615]
                      tunnel: string[] ["CLOSE CAM", "DISPOSE BUFFERS", "RESET ENCODERS", "RESET YAW", "RESET FLAGS", ""] -> [w2613] mode=indexing
                      n840 = Enqueue Element(queue=w2615, element=w2613) -> (queue out=w2614:refnum<queue>)  [unwired: 2 in, 2 out]
                    }
                  }
                }
                n841 = Or(x=w2595, y=w2594) -> (x .or. y?=w2593:bool)
                n842 = Select(t=State_Type_Definitions,_for_0.26g_versions_and_later_2."True Stop" ("Enum"), s=w2594, f=State_Type_Definitions."Task 9P: MOVE RIGHT" ("Enum")) -> (s? t:f=w2596:u16)
                n843 = Select(t=w2596, s=w2593, f=State_Type_Definitions."Task 9O: PROCESS COLOUR" ("Enum")) -> (s? t:f=w2602:u16)
              }
              frame "Exit" {
                n844 = for {
                  shift-right: [w2622] -> w2619
                  shift-left: w2618 -> [w2623]
                  tunnel: string[] ["STOP", "RESET ENCODERS", "RESET YAW", "ARDUINO MODE 0"] -> [w2621] mode=indexing
                  n845 = Enqueue Element(queue=w2623, element=w2621) -> (queue out=w2622:refnum<queue>)  [unwired: 2 in, 2 out]
                }
              }
            }
          }
          frame 53 {
            # ">> Item Selection Bias >>"
            n846 = Dequeue Element(queue=w2629, timeout in ms (-1)=w2628, error in (no error)=w2627) -> (element=w2637:T8)  [unwired: 3 out]
            n847 = Greater?(x=w2625, y=50.0) -> (0:w2635:bool)
            n848 = And(x=w2624, y=w2635) -> (x .and. y?=w2636:bool)
            n849 = case shown="\"Start Task 1\", Default" w2637 {
              tunnel: w2636 -> [w2643 _]
              tunnel: [w2650 State_Type_Definitions,_for_0.26g_versions_and_later_2."True Stop" ("Enum")] -> w2632
              tunnel: w2626 -> [w2642 _]
              tunnel: w2630 -> [w2649 w2666]
              tunnel: [w2648 w2667] -> w2631
              tunnel: [State_Type_Definitions,_for_0.26g_versions_and_later_2."Idle" ("Enum") State_Type_Definitions,_for_0.26g_versions_and_later_2."Shutdown" ("Enum")] -> w2633
              frame "Start Task 1", Default {
                n850 = case shown="False" w2643 {
                  tunnel: w2649 -> [w2653 w2660]
                  tunnel: [w2654 w2659] -> w2648
                  frame False {
                    n851 = for {
                      tunnel: string[] ["READ LINE SENSOR", "READ NAVX", "RIGHT", "READ ENCODERS"] ("element") -> [w2655] mode=indexing
                      shift-right: [w2657] -> w2654
                      shift-left: w2653 -> [w2656]
                      n852 = Enqueue Element(queue=w2656, element=w2655) -> (queue out=w2657:refnum<queue>)  [unwired: 2 in, 2 out]
                    }
                  }
                  frame True {
                    n853 = for {
                      shift-right: [w2662] -> w2659
                      shift-left: w2660 -> [w2663]
                      tunnel: string[] ["STOP", "RESET ENCODERS", "RESET YAW", "OPEN LIFE CAM", "SET TIMER 2", "RESET FLAGS"] -> [w2661] mode=indexing
                      n854 = Enqueue Element(queue=w2663, element=w2661) -> (queue out=w2662:refnum<queue>)  [unwired: 2 in, 2 out]
                    }
                  }
                }
                n855 = Or(x=w2643, y=w2642) -> (x .or. y?=w2641:bool)
                n856 = Select(t=State_Type_Definitions,_for_0.26g_versions_and_later_2."True Stop" ("Enum"), s=w2642, f=State_Type_Definitions."Task 9Q: SCAN IMAGE" ("Enum")) -> (s? t:f=w2644:u16)
                n857 = Select(t=w2644, s=w2641, f=State_Type_Definitions."Task 9P: MOVE RIGHT" ("Enum")) -> (s? t:f=w2650:u16)
              }
              frame "Exit" {
                n858 = for {
                  shift-right: [w2670] -> w2667
                  shift-left: w2666 -> [w2671]
                  tunnel: string[] ["STOP", "RESET ENCODERS", "RESET YAW", "ARDUINO MODE 0"] -> [w2669] mode=indexing
                  n859 = Enqueue Element(queue=w2671, element=w2669) -> (queue out=w2670:refnum<queue>)  [unwired: 2 in, 2 out]
                }
              }
            }
          }
          frame 54 {
            # ">> Manual override >>"
            n860 = Dequeue Element(queue=w2680, timeout in ms (-1)=w2679, error in (no error)=w2678) -> (element=w2681:T8)  [unwired: 3 out]
            n861 = case shown="\"Start Task 1\", Default" w2681 {
              tunnel: [w2695 State_Type_Definitions,_for_0.26g_versions_and_later_2."True Stop" ("Enum")] -> w2673
              tunnel: [w2693 w2711] -> w2672
              tunnel: w2676 -> [w2692 w2708]
              tunnel: w2677 -> [w2686 _]
              tunnel: [State_Type_Definitions,_for_0.26g_versions_and_later_2."Idle" ("Enum") State_Type_Definitions,_for_0.26g_versions_and_later_2."Shutdown" ("Enum")] -> w2674
              tunnel: w2675 -> [w2685 _]
              frame "Start Task 1", Default {
                # ">> WIill proceed to part ii if not manual override >>"
                # ">>If ENABLE or Trigger is set to true>>"
                n862 = Or(x=w2685, y=w2686) -> (x .or. y?=w2687:bool)
                n863 = case shown="False" w2685 {
                  tunnel: [w2698 w2704] -> w2693
                  tunnel: w2692 -> [w2697 w2703]
                  frame False {
                    n864 = for {
                      shift-right: [w2700] -> w2698
                      shift-left: w2697 -> [w2701]
                      tunnel: string[] ["CAM ACQ", "START TIMER"] ("element") -> [w2699] mode=indexing
                      n865 = Enqueue Element(queue=w2701, element=w2699) -> (queue out=w2700:refnum<queue>)  [unwired: 2 in, 2 out]
                    }
                  }
                  frame True {
                    n866 = for {
                      shift-right: [w2706] -> w2704
                      shift-left: w2703 -> [w2707]
                      tunnel: string[] ["CLOSE CAM", "SET TIMER 5", "", "", "", ""] -> [w2705] mode=indexing
                      n867 = Enqueue Element(queue=w2707, element=w2705) -> (queue out=w2706:refnum<queue>)  [unwired: 2 in, 2 out]
                    }
                  }
                }
                n868 = Select(t=State_Type_Definitions,_for_0.26g_versions_and_later_2."True Stop" ("Enum"), s=w2686, f=State_Type_Definitions,_for_0.26g_versions_and_later_2."Task 9R: PROCESS COLOUR" ("Enum")) -> (s? t:f=w2689:T16)
                n869 = Select(t=w2689, s=w2687, f=State_Type_Definitions."Task 9Q: SCAN IMAGE" ("Enum")) -> (s? t:f=w2695:u16)
              }
              frame "Exit" {
                n870 = for {
                  shift-right: [w2714] -> w2711
                  shift-left: w2708 -> [w2715]
                  tunnel: string[] ["STOP", "RESET ENCODERS", "RESET YAW", ""] -> [w2713] mode=indexing
                  n871 = Enqueue Element(queue=w2715, element=w2713) -> (queue out=w2714:refnum<queue>)  [unwired: 2 in, 2 out]
                }
              }
            }
          }
          frame 55 {
            # ">> Item Selection Bias >>"
            # ">>> Motor control cluster >>>"
            # ">>> yStepper command>>>"
            n872 = Dequeue Element(queue=w2721, timeout in ms (-1)=w2722, error in (no error)=w2723) -> (element=w2725:T8)  [unwired: 3 out]
            n873 = case shown="\"Start Task 1\", Default" w2725 {
              tunnel: w2719 -> [w2731 _]
              tunnel: [w2738 State_Type_Definitions,_for_0.26g_versions_and_later_2."True Stop" ("Enum")] -> w2717
              tunnel: w2724 -> [w2730 _]
              tunnel: w2720 -> [w2737 w2754]
              tunnel: [w2736 w2755] -> w2716
              tunnel: [State_Type_Definitions,_for_0.26g_versions_and_later_2."Idle" ("Enum") State_Type_Definitions,_for_0.26g_versions_and_later_2."Shutdown" ("Enum")] -> w2718
              frame "Start Task 1", Default {
                n874 = case shown="False" w2731 {
                  tunnel: w2737 -> [w2741 w2748]
                  tunnel: [w2742 w2747] -> w2736
                  frame False {
                    n875 = for {
                      tunnel: string[] ["START TIMER", "COLOUR PROCESSING", ""] ("element") -> [w2743] mode=indexing
                      shift-right: [w2745] -> w2742
                      shift-left: w2741 -> [w2744]
                      n876 = Enqueue Element(queue=w2744, element=w2743) -> (queue out=w2745:refnum<queue>)  [unwired: 2 in, 2 out]
                    }
                  }
                  frame True {
                    n877 = for {
                      shift-right: [w2750] -> w2747
                      shift-left: w2748 -> [w2751]
                      tunnel: string[] ["CLOSE CAM", "DISPOSE BUFFERS", "RESET ENCODERS", "RESET YAW", "RESET FLAGS", ""] -> [w2749] mode=indexing
                      n878 = Enqueue Element(queue=w2751, element=w2749) -> (queue out=w2750:refnum<queue>)  [unwired: 2 in, 2 out]
                    }
                  }
                }
                n879 = Or(x=w2731, y=w2730) -> (x .or. y?=w2729:bool)
                n880 = Select(t=State_Type_Definitions,_for_0.26g_versions_and_later_2."True Stop" ("Enum"), s=w2730, f=State_Type_Definitions,_for_0.26g_versions_and_later_2."True Stop" ("Enum")) -> (s? t:f=w2732:T16)
                n881 = Select(t=w2732, s=w2729, f=State_Type_Definitions,_for_0.26g_versions_and_later_2."Task 9R: PROCESS COLOUR" ("Enum")) -> (s? t:f=w2738:T16)
              }
              frame "Exit" {
                n882 = for {
                  shift-right: [w2758] -> w2755
                  shift-left: w2754 -> [w2759]
                  tunnel: string[] ["STOP", "RESET ENCODERS", "RESET YAW", "ARDUINO MODE 0"] -> [w2757] mode=indexing
                  n883 = Enqueue Element(queue=w2759, element=w2757) -> (queue out=w2758:refnum<queue>)  [unwired: 2 in, 2 out]
                }
              }
            }
          }
        }
        "Object Detection" <- w300
        "Ultrasonic sensors" <- w323
        "Encoder values" <- w312
        "Stepper position values" <- w296
        "NAVX Values" <- w294
        "Time up" <- w292
        "IR Sensors" <- w286
        "Line sensors" <- w281
      }
    }
    "Object recognition mode" <- w212
    n884 = local write "Green LED"(w222) -> ()
  }
  n885 = while {
    stop <- w3522 stop-if-true
    n886 = call "MOTOR CONTROL WITH PID AE.vi"("AE Mode"=MOTOR_CONTROL_WITH_PID_AE_DATA_MODE_TYPE_DEF."Read from AE") -> ("Speed & distance"=→"Speed & distance":T13)  [unwired: 3 in]
    n887 = call "FGV Bool.vi"("Init/Read/Write State"=States_for_Action_Engine."Read") -> ("Output node"=w3522:bool)  [unwired: 2 in, 1 out]
    n888 = Wait (ms)(milliseconds to wait=u32 5) -> ()  [unwired: 1 out]
  }
  n889 = call <vilib>:"DIO Close.vi"("error in (no error)"=w22, "DIO Info In"=w25) -> ()  [unwired: 9 in, 1 out]
  n890 = call <vilib>:"DIO Close.vi"("error in (no error)"=w32, "DIO Info In"=w34) -> ()  [unwired: 9 in, 1 out]
  n891 = call <vilib>:"NavX Close.vi"("error in (no error)"=w9, "NavX Info In"=w8) -> ()  [unwired: 9 in, 1 out]
  n892 = call <vilib>:"DIO Close.vi"("error in (no error)"=w27, "DIO Info In"=w29) -> ()  [unwired: 9 in, 1 out]
  n893 = call <vilib>:"DIO Close.vi"("error in (no error)"=w16, "DIO Info In"=w17) -> ()  [unwired: 9 in, 1 out]
  n894 = call <vilib>:"DIO Close.vi"("error in (no error)"=w11, "DIO Info In"=w12) -> ()  [unwired: 9 in, 1 out]
  n895 = Merge Errors "Merge Errors"(w62, w61) -> (w44:errorcluster)
  n896 = Merge Errors(w48, w44) -> (w43:errorcluster)
  n897 = Destroy User Event(user event=w66, error in=w43) -> ()  [unwired: 1 out]
  n898 = Release Queue(queue=w39, error in (no error)=w43) -> (error out=→"Queue Errors":errorcluster)  [unwired: 1 in, 2 out]
  n899 = Release Queue(queue=w56, error in (no error)=w43) -> ()  [unwired: 1 in, 3 out]
  n900 = Destroy User Event(user event=w65, error in=w43) -> ()  [unwired: 1 out]
  n901 = Unregister For Events(event registration refnum=w57, error in=w43) -> ()  [unwired: 1 out]
